vi "Optical Power Meter Utility.vi"() -> ()   [LabVIEW 2011]
uses:
  StateMachine.ctl
  <vilib>/printing/EasyPrintingControls.llb/layout_options.ctl
  <vilib>/printing/EasyPrintingControls.llb/orientation.ctl
  <vilib>/printing/EasyPrintingControls.llb/panel_scaling_for_page.ctl
  <vilib>/printing/EasyPrintingControls.llb/margins.ctl
  <vilib>/printing/EasyPrintingControls.llb/margin_values.ctl
  <vilib>/printing/EasyPrintingControls.llb/measurement_system.ctl
  <vilib>/printing/EasyPrintingControls.llb/printer_options.ctl
  <vilib>/printing/EasyPrintingControls.llb/printing_method.ctl
  <vilib>/printing/EasyPrintingControls.llb/color_or_monochrome.ctl
  <vilib>/printing/EasyPrintingControls.llb/page_header_options.ctl
  <vilib>/printing/EasyPrintingControls.llb/page_headers.ctl
  <vilib>/printing/EasyPrintingControls.llb/page_header_content_options.ctl
  <vilib>/printing/EasyPrintingControls.llb/report_type.ctl
  <vilib>/printing/EasyPrintingControls.llb/contents.ctl
  <vilib>/Utility/sysdir.llb/System Directory Type.ctl
  <vilib>/Instr/_visa.llb/VISA GPIB Control REN Mode.ctl
  <vilib>/Utility/config.llb/Write Key (I32).vi
  <vilib>/Utility/config.llb/Write Key (U32).vi
  <vilib>/Utility/config.llb/Write Key (Boolean).vi
  <vilib>/Utility/config.llb/Write Key (Double).vi
  <vilib>/printing/EasyPrinting.llb/Easy Print VI Panel or Documentation (path).vi
  <vilib>/Utility/config.llb/Read Key (I32).vi
  <vilib>/Utility/config.llb/Read Key (Double).vi
  <vilib>/Utility/config.llb/Read Key (Boolean).vi
  <vilib>/regexp/Match Regular Expression.xnode
  <vilib>/ptbypt/NI_PtbyPt.lvlib
  <vilib>/Utility/config.llb/NI_LVConfig.lvlib
  <vilib>/Utility/NIReport.llb/NI_ReportGenerationCore.lvlib
  <vilib>/Analysis/NI_AALBase.lvlib
panel:
  in  "Setup":string
  out "Res":bool
  out "Data_Dir":path
  in  "att":string
  in  "Print":bool
  in  "LTM":bool caption="Long Term Measurement"
  out "Log":bool
  in  "Arm":string
  out "VI_Path":path
  in  "Button9":bool
  in  "Button10":bool
  out "Adapter":i16
  in  "Flag1":string
  in  "Flag0":string
  out "Tau":dbl
  out "Tau?":bool
  out "Temp":bool
  out "ARM":bool
  out "Stop":bool
  in  "Frame":T1
  out "Sensor?":bool
  out "SensType":i32(ring) items=["No Sensor", "Photo", "Thermo", "Pyro"]
  out "AUTO?":bool
  out "DiaIni":dbl
  out "PM100D":refnum<visa-resource-name>
  in  "Type":u16
  in  "BW":u16(ring) items=["HIGH", "LOW"]
  in  "ACC":string(combo)
  in  "Trig":dbl=5.0
  out "AOutcm²":dbl=5.0
  in  "LambdaMax":dbl=1100.0
  in  "LambdaMin":dbl=400.0
  in  "Lambda":dbl=635.0
  in  "Range Array":string[](array[string])=["AUTO", "50nA", "500nA", "5uA", "50uA", "500uA", "5mA"]
  out "Dia":dbl
  out "SlideMulti":dbl
  in  "AVG":u32=100
  out "FileRefnum":refnum<file>
  in  "File?":bool
  in  "Samples":u32=100
  out "N":u32
  out "Data":dbl
  in  "Interval":dbl=500.0
  in  "MainUnits":enum16{"W", "V", "J", "dBm", "A"}(ring)
  in  "Digits":i32=4
  in  "Sub2":enum16{"Off", "Max", "Ratio", "Area", "Second"}(ring)=enum."Max"
  in  "Sub1":enum16{"Off", "Min", "Freq", "Temp", "Res"}(ring)=enum."Min"
  in  "Button8":bool
  in  "Button7":bool
  in  "Button6":bool
  in  "Button4":bool
  in  "Button3":bool
  in  "Button2":bool
  in  "Button5":bool
  in  "Button1":bool
  out "Header":string
  out "Slide":u32(slide) scale=0.0..1000.0
  out "Sub1":string
  out "Sub2":string
  out "Readout":string
  out "FastOut":bool
  in  "FastIn":bool
  in  "Int.":i32=10 caption="Intervals" min=1 max=9999 step=1
  in  "LogCfg":string
  in  "Stat2":string
  in  "Stat1":string
  in  "Stat0":string
  out "Histogram":T2(graph)
  in  "LogData":string
  out "YT":cluster{timestamp[], dbl[]}(graph)
  out "Unit":string="Power / W"
  out "Chart_E":dbl(graph)
  out "Chart_P":dbl(graph)
  in  "NPL":i32=1 min=1 max=100 step=1
  out "16":bool
  in  "Att":dbl format="%_6g"
  out "Wav":bool
  in  "Scale":bool
  out "H":dbl
  in  "Unt":string
  in  "LFP":path caption="Log-File Path"
  in  "Imp":bool
  out "N2":u32
  out "T":dbl
  in  "EMM":bool caption="Environmental Data"
  out "Hum":string caption="Rel. Humidity"
  out "Temp":string caption="Temperature"
  in  "Exp":bool
  in  "ClrGr":bool
  in  "XScaleFit":bool
  in  "YScaleRep":bool
  in  "YScaleFit":bool
  # "PM Series\nOptical Power and Energy Meters"
  # "Count >"
  # "Histogram"
  # "Y-Scale"
  # "Scale Fit"
  # "Map Mode"
  # "X-Scale"
  # "Scale Fit"
  # "Scale"
  # "PM100 Utility\nVersion 5.4\n12-MAY-2015\nwww.thorlabs.com"
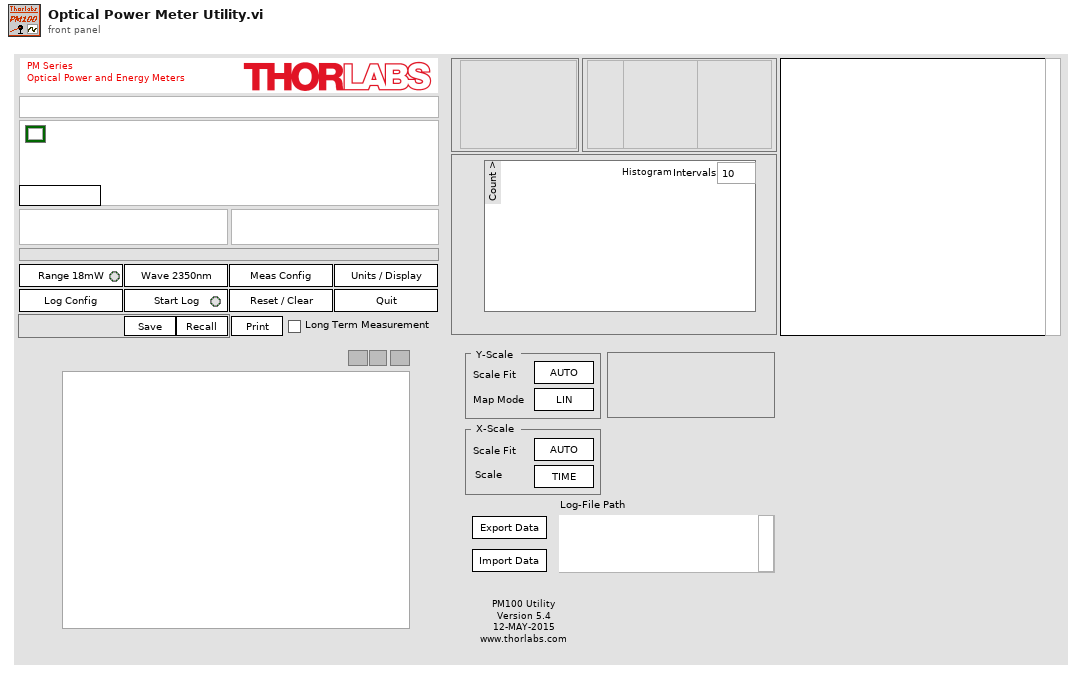
[diagram p1: front panel]
types:
  T1 = typedef "StateMachine.ctl" = enum16{"Initialize", "Load Settings", "20", "30", "40", "60", "80", "100", "120", "130", "140", "150", "160", "180", "200", "220", "240", "260", "280", "300", "320", "340", "360", "380", "400", "420", "440", "460", "480", "500", "Error", "Save Settings", "Stop"}
  T2 = cluster{"X Values":dbl[], "Histogram: h(x)":i32[]}
  T3 = enum16{"open", "replace", "create", "open or create", "replace or create", "replace or create with confirmation"}
  T4 = cluster{"X Values":i32[], "Histogram: h(x)":i32[]}
  T5 = typedef "NI_ReportGenerationCore.lvlib/layout_options.ctl" = cluster{"orientation (unchanged)":T6, "panel scaling for page (unchanged)":T7, "margins":T8, "printer options":T11, "page header options":T14}
  T6 = typedef "NI_ReportGenerationCore.lvlib/orientation.ctl" = u16
  T7 = typedef "NI_ReportGenerationCore.lvlib/panel_scaling_for_page.ctl" = u16
  T8 = typedef "NI_ReportGenerationCore.lvlib/margins.ctl" = cluster{"override VI margins (false)":bool, "margins (1.00)":T9, "measurement system (default)":T10}
  T9 = typedef "NI_ReportGenerationCore.lvlib/margin_values.ctl" = cluster{"top":dbl, "left":dbl, "right":dbl, "bottom":dbl}
  T10 = typedef "NI_ReportGenerationCore.lvlib/measurement_system.ctl" = u16
  T11 = typedef "NI_ReportGenerationCore.lvlib/printer_options.ctl" = cluster{"destination printer name (current)":string, "printing method (unchanged)":T12, "color or monochrome (unchanged)":T13}
  T12 = typedef "NI_ReportGenerationCore.lvlib/printing_method.ctl" = u16
  T13 = typedef "NI_ReportGenerationCore.lvlib/color_or_monochrome.ctl" = u16
  T14 = typedef "NI_ReportGenerationCore.lvlib/page_header_options.ctl" = cluster{"page headers (unchanged)":T15, "page header content options":T16}
  T15 = typedef "NI_ReportGenerationCore.lvlib/page_headers.ctl" = u16
  T16 = typedef "NI_ReportGenerationCore.lvlib/page_header_content_options.ctl" = cluster{"Include VI Name":bool, "Include VI Path":bool, "Include Last Modification Date":bool, "Include Date Printed":bool, "Include Page Number":bool, "Include VI Icon":bool}
  T17 = typedef "NI_LVConfig.lvlib/Config Data RefNum.ctl" = refnum<k1>
  T18 = typedef "NI_ReportGenerationCore.lvlib/report_type.ctl" = u16
  T19 = typedef "NI_ReportGenerationCore.lvlib/contents.ctl" = u16
  T20 = typedef "System Directory Type.ctl" = i32
  T21 = enum32{"invalid app kind", "Development System", "Run Time System", "Student Edition", "Embedded LabVIEW", "Evaluation", "Custom"}
  T22 = typedef "VISA GPIB Control REN Mode.ctl" = u16
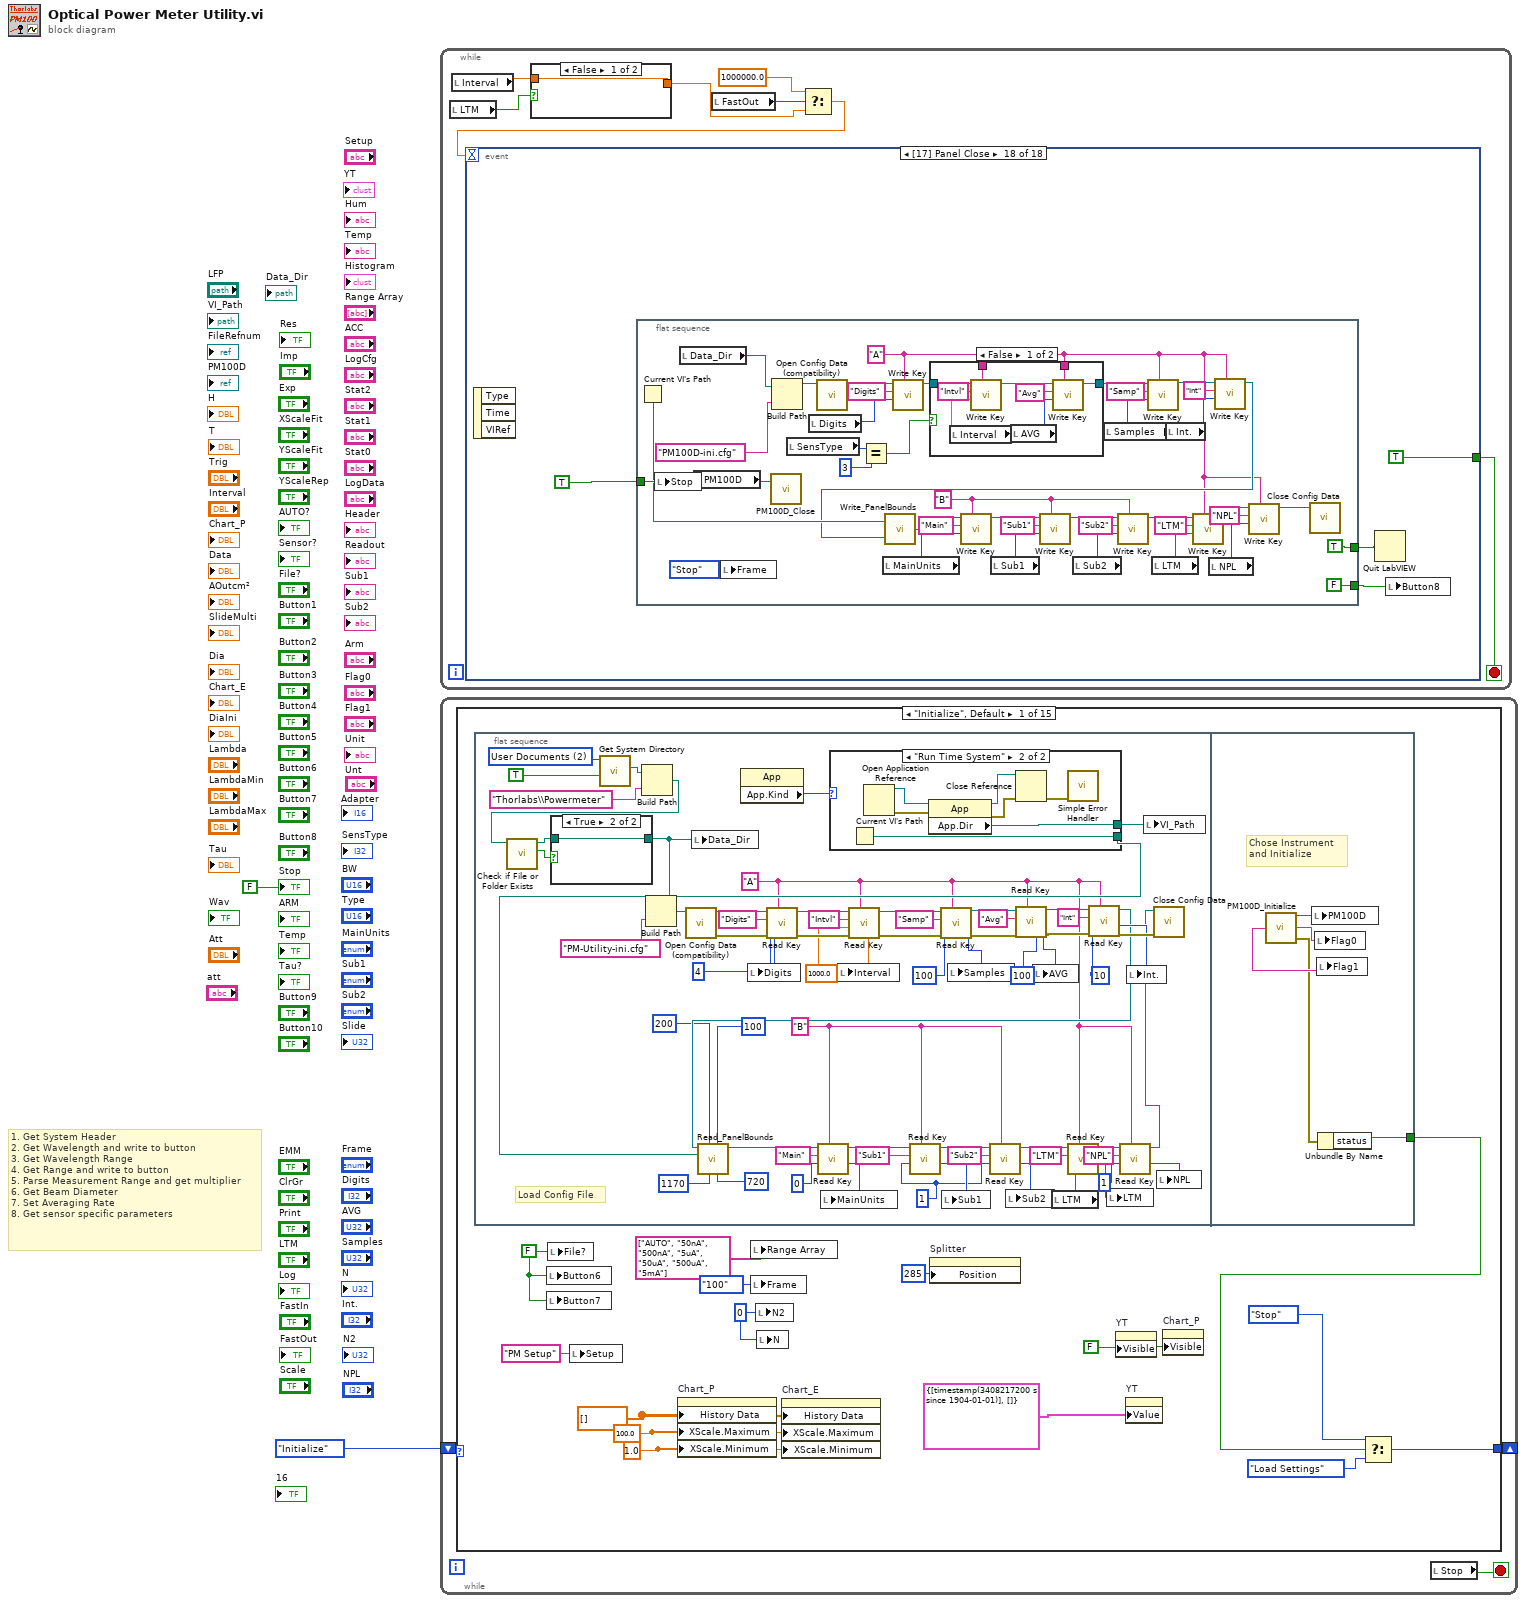
[diagram p0: block diagram]
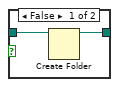
[diagram p2: hidden frame]
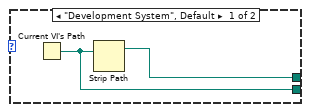
[diagram p3: hidden frame]
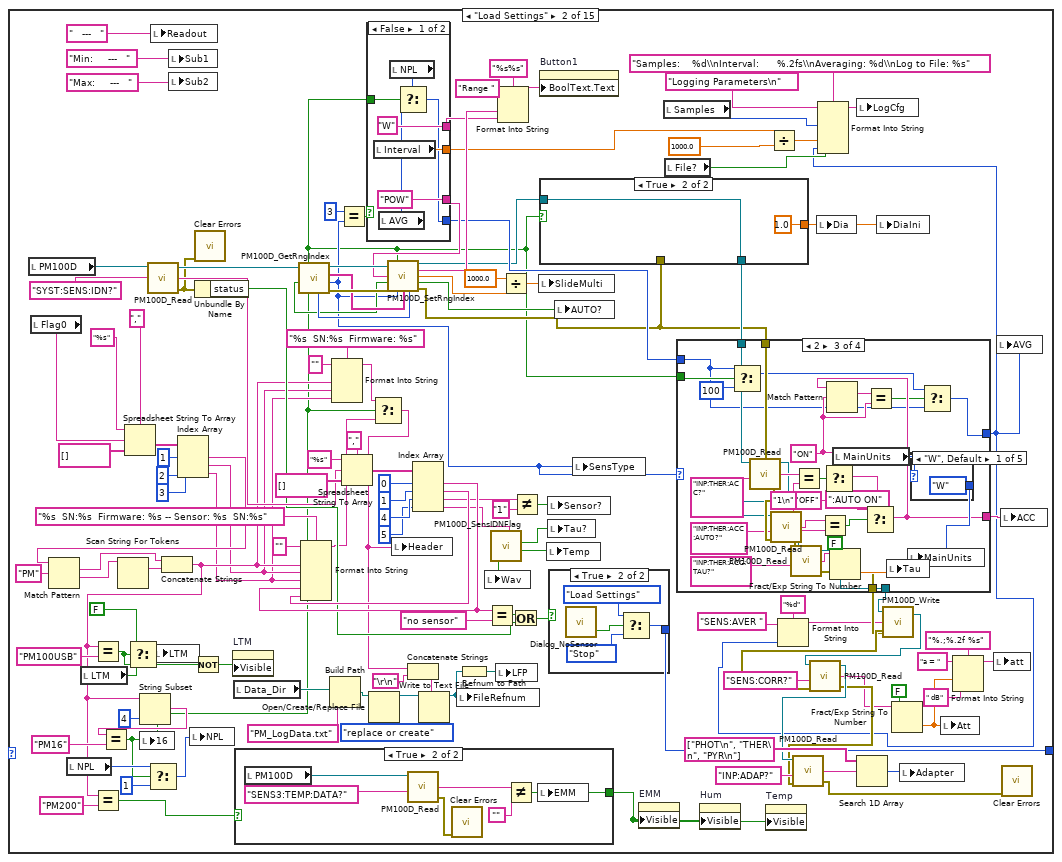
[diagram p4: hidden frame]
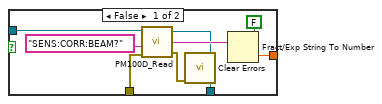
[diagram p5: hidden frame]
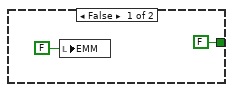
[diagram p6: hidden frame]
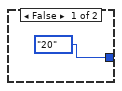
[diagram p7: hidden frame]
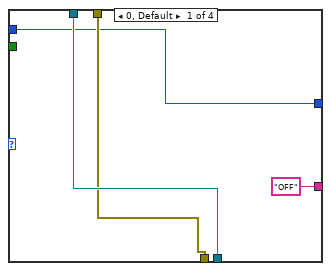
[diagram p8: hidden frame]
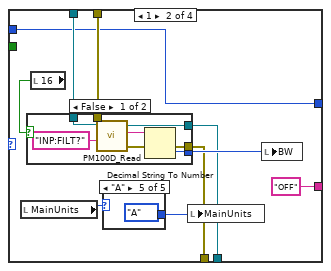
[diagram p9: hidden frame]
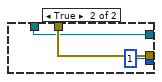
[diagram p10: hidden frame]
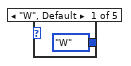
[diagram p11: hidden frame]
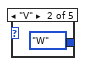
[diagram p12: hidden frame]
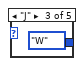
[diagram p13: hidden frame]
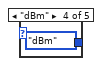
[diagram p14: hidden frame]
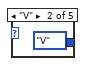
[diagram p15: hidden frame]
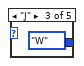
[diagram p16: hidden frame]
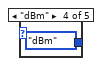
[diagram p17: hidden frame]
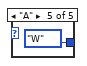
[diagram p18: hidden frame]
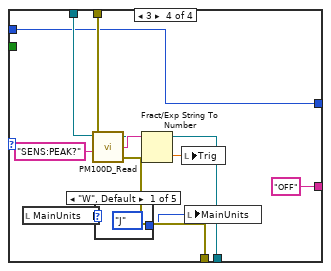
[diagram p19: hidden frame]
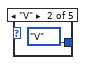
[diagram p20: hidden frame]
diagram:
  # "1. Get System Header\n2. Get Wavelength and write to button\n3. Get Wavelength Range\n4. Get Range and write to button\n5. Parse Measurement Range and get multiplier\n6. Get Beam Diameter\n7. Set Averaging Rate\n8. Get sensor specific parameters"
  n1 = while {
    stop <- w9 stop-if-true
    n2 = local read "LTM"() -> (w7:bool)
    n3 = local read "Interval"() -> (w8:dbl)
    n4 = case shown="False" w7 {
      tunnel: w8 -> [w10 w12]
      tunnel: [w10 w11] -> w4
      frame False {
      }
      frame True {
        n5 = Add(x=w12, y=100.0) -> (x+y=w11:dbl)
      }
    }
    n6 = local read "FastOut"() -> (w6:bool)
    n7 = Select(t=1000000.0, s=w6, f=w4) -> (s? t:f=w5:dbl)
    n8 = event shown="[17] Panel Close" {
      selector: _ -> [_ _ _ _ _ _ _ _ _ _ _ _ _ _ _ _ _ _]
      dyn-events: _ -> [_ _ _ _ _ _ _ _ _ _ _ _ _ _ _ _ _ _]
      timeout: w5 -> [_ _ _ _ _ _ _ _ _ _ _ _ _ _ _ _ _ _]
      tunnel: [_ _ _ _ _ _ _ _ _ TRUE ("NewVal") _ _ _ _ _ _ w537 TRUE ("NewVal")] -> w9
      event Timeout {
        # "Logging via Timeout\nmin. 0.1s interval"
        n9 = event-data() -> ()  [unwired: 1 in, 2 out]
        n10 = local read "Samples"() -> (w27:u32)
        n11 = local read "Button6"() -> (w15:bool)
        n12 = local read "SensType"() -> (w25:i32)
        n13 = local read "N"() -> (w29:u32)
        n14 = local read "Button1"() -> (w16:bool)
        n15 = local read "Button2"() -> (w17:bool)
        n16 = local read "Button3"() -> (w18:bool)
        n17 = local read "Button4"() -> (w19:bool)
        n18 = local read "Button5"() -> (w20:bool)
        n19 = Increment(x=w29) -> (x+1=w26:u32)
        n20 = Not Equal?(x=w25, y=3) -> (x != y?=w22:bool)
        n21 = Decrement(x=w26) -> (x-1=w28:u32)
        n22 = Not Equal?(x=w27, y=w28) -> (x != y?=w23:bool)
        n23 = local write "N"(w26) -> ()
        n24 = Compound Arithmetic op=AND(invert w16, invert w17, invert w18, invert w19, invert w20, w15, w22, w23) -> (w30:bool)
        n25 = case shown="True" w30 {
          tunnel: w27 -> [w36 w60]
          tunnel: w26 -> [w32 w59]
          tunnel: [0 w49] -> w21
          tunnel: w15 -> [w38 _]
          tunnel: [FALSE TRUE] -> w14
          frame False {
            n26 = Equal?(x=w38, y=TRUE) -> (x = y?=w35:bool)
            n27 = Less?(x=w32, y=w36) -> (x < y?=w34:bool)
            n28 = And(x=w35, y=w34) -> (x .and. y?=w33:bool)
            n29 = case shown="True" w33 {
              frame False {
                n30 = local write "Button6"(FALSE ("Button6")) -> ()
                n31 = local write "N"(i16 0 ("N")) -> ()
              }
              frame True {
                n32 = disable-structure shown="Enabled" {
                  frame Enabled {
                    n33 = local read "N"() -> (w43:u32)
                    n34 = Decrement(x=w43) -> (x-1=w42:u32)
                    n35 = local write "N"(w42) -> ()
                  }
                  frame Disabled {
                  }
                }
              }
            }
          }
          frame True {
            n36 = local read "PM100D"() -> (w46:refnum<visa-resource-name>)
            n37 = local read "MainUnits"() -> (w89:enum16{"W", "V", "J", "dBm", "A"})
            n38 = case shown="\"V\"" w89 {
              tunnel: ["W" "V" "J" "dBm" "A"] -> w53
              tunnel: [w133 w137 w140 FALSE w150] -> w73
              tunnel: [FALSE w137 TRUE FALSE w150] -> w72
              tunnel: [w133 TRUE w140 TRUE TRUE] -> w71
              tunnel: ["MEAS?" ("Command") "MEAS:VOLT?" ("Command") "MEAS:ENER?" ("Command") "MEAS?" ("Command") "MEAS:CURR?" ("Command")] -> w44
              frame "W", Default {
                w133 = TRUE
              }
              frame "V" {
                w137 = FALSE
              }
              frame "J" {
                w140 = FALSE
              }
              frame "dBm" {
              }
              frame "A" {
                w150 = FALSE
              }
            }
            n39 = disable-structure shown="Enabled" {
              disable-tunnel: [w99 w102] -> w57
              disable-tunnel: w46 -> [w97 w104]
              disable-tunnel: [w96 w101] -> w45
              disable-tunnel: w44 -> [w95 w103]
              frame Disabled {
                n40 = call "PM100D_Read.vi"("Command"=w95, "VISA in"=w97) -> ("error out"=w98:errorcluster, "ReadValue"=w99:string)  [unwired: 2 in, 1 out]
                n41 = Unbundle By Name(w98) -> ("status"=w96:bool)
                n42 = call <vilib>:"Clear Errors.vi"("error in (no error)"=w98) -> ()  [unwired: 6 in, 1 out]
              }
              frame Enabled {
                n43 = local read "NPL"() -> (w100:i32)
                n44 = call "PM100D_Meas_NPLC.vi"("Command"=w103, "NCPL"=w100, "VISA Refnum in"=w104) -> ("Error"=w101:bool, "Value"=w102:string)  [unwired: 5 in, 2 out]
              }
            }
            n45 = Equal?(x=i16 1, y=w59) -> (x = y?=w90:bool)
            n46 = case shown="True" w45 {
              tunnel: w46 -> [_ w105]
              frame False {
              }
              frame True {
                n47 = VISA Clear(VISA resource name=w105) -> ()  [unwired: 1 in, 2 out]
              }
            }
            n48 = Fract/Exp String To Number(use system decimal point (T)=FALSE, string=w57) -> (number=w55:dbl)  [unwired: 2 in, 1 out]
            n49 = local read "Int."() -> (w70:i32)
            n50 = Equal?(x="dBm", y=w53) -> (x = y?=w51:bool)
            n51 = local read "EMM"() -> (w66:bool)
            n52 = case shown="True" w51 {
              tunnel: w55 -> [w106 w108]
              tunnel: [w106 w107] -> w54
              frame False {
              }
              frame True {
                n53 = Multiply(x=w108, y=1000.0) -> (x*y=w110:dbl)
                n54 = Logarithm Base 10(1:w110) -> (0:w112:dbl)
                n55 = Multiply(x=10.0, y=w112) -> (x*y=w107:dbl)
              }
            }
            n56 = property on="Chart_E" class="WFChart (strict)"("Visible"=w72) -> ()  [unwired: 2 in, 2 out]
            n57 = property on="Chart_P" class="WFChart (strict)"("Visible"=w71) -> ()  [unwired: 2 in, 2 out]
            n58 = call <vilib>:"Histogram PtByPt.vi"("initialize"=w90, "sample length"=w60, "intervals"=w70, "x"=w54) -> ("Histogram Graph"=w93:T2)  [unwired: 4 in, 3 out]
            n59 = call <vilib>:"Array Max & Min PtByPt.vi"("input data point"=w54, "sample length"=w60, "initialize"=w90) -> ("max value"=w81:dbl, "min value"=w82:dbl)  [unwired: 3 out]
            n60 = call <vilib>:"Standard Deviation PtByPt.vi"("x"=w54, "sample length"=w60, "initialize"=w90) -> ("standard deviation"=w88:dbl, "mean"=w80:dbl)  [unwired: 1 out]
            n61 = call <vilib>:"RMS PtByPt.vi"("initialize"=w90, "sample length"=w60, "x"=w54) -> ("rms value"=w79:dbl)  [unwired: 1 in, 1 out]
            n62 = call "GetDateTime.vi"() -> ("date&time"=w47:string)
            n63 = Format Into String(format string="%d\\n%.3p%s\\n%.3p%s\\n%.3p%s\\n%.3p%s\\n%.3p%s", w59, w82, w53, w81, w53, w80, w53, w79, w53, w88, w53) -> (resulting string=w92:string)  [unwired: 2 in, 1 out]
            n64 = case shown="True" w66 {
              tunnel: [w124 w129] -> w50
              tunnel: w54 -> [w123 w128]
              tunnel: w53 -> [w122 w127]
              tunnel: w47 -> [w121 w126]
              frame True {
                n65 = local read "H"() -> (w119:dbl)
                n66 = local read "T"() -> (w120:dbl)
                n67 = Format Into String(format string="\\t%.4e\\t%s\\t%.1f\\t°C\\t%.1f\\tRH\\n", initial string=w121, w123, w122, w120, w119) -> (resulting string=w124:string)  [unwired: 1 in, 1 out]
              }
              frame False {
                n68 = Format Into String(format string="\\t%.4e\\t%s\\n", initial string=w126, w128, w127) -> (resulting string=w129:string)  [unwired: 1 in, 1 out]
              }
            }
            n69 = Concatenate Strings("Power / " ("string"), w53) -> (w68:string)
            n70 = local write "Unit"(w68) -> ()
            n71 = local write "Chart_E"(w54) -> ()
            n72 = call "lin-log.vi"("W In 1"=w79, "W In 2"=w80, "W In 3"=w81, "W In 4"=w82) -> ("dBm Out 1"=w83:dbl, "dBm Out 2"=w84:dbl, "dBm Out 3"=w85:dbl, "dBm Out 4"=w86:dbl)
            n73 = local write "Histogram"(w93) -> ()
            n74 = Format Into String(format string="%.3fdBm\\n%.3fdBm\\n%.3fdBm\\n%.3fdBm", initial string="\n", w86, w85, w84, w83) -> (resulting string=w77:string)  [unwired: 1 in, 1 out]
            n75 = local write "Chart_P"(w54) -> ()
            n76 = local read "FileRefnum"() -> (w63:refnum<file>)
            n77 = local write "Stat1"(w92) -> ()
            n78 = local write "Stat0"("Count:\nMin:\nMax:\nMean:\nRMS:\nSigma:" ("Stat0")) -> ()
            n79 = local read "LogData"() -> (w64:string)
            n80 = Select(t=w77, s=w73, f="") -> (s? t:f=w76:string)
            n81 = property on="YT" class="XYGraph (strict)"("Visible"=FALSE) -> ()  [unwired: 2 in, 2 out]
            n82 = Equal?(x=w60, y=w59) -> (x = y?=w61:bool)
            n83 = Concatenate Strings(w50, w64) -> (w65:string)
            n84 = local write "Stat2"(w76) -> ()
            n85 = Write to Text File(file (use dialog)=w63, text=w50) -> (refnum out=w58:refnum<file>)  [unwired: 2 in, 2 out]
            n86 = local write "LogData"(w65) -> ()
            n87 = case shown="True" w61 {
              tunnel: [StateMachine."120" ("Frame") StateMachine."300" ("Frame")] -> w62
              tunnel: w58 -> [_ w117]
              tunnel: [2 0] -> w49
              frame False {
              }
              frame True {
                n88 = Refnum to Path(1:w117) -> (0:w116:path)
                n89 = local write "LFP"(w116) -> ()
              }
            }
            n90 = local write "Frame"(w62) -> ()
          }
        }
        n91 = local write "Log"(w14) -> ()
        n92 = property on="Button1" class="Bool (strict)"("Disabled"=w21) -> ()  [unwired: 2 in, 2 out]
        n93 = property on="Button2" class="Bool (strict)"("Disabled"=w21) -> ()  [unwired: 2 in, 2 out]
        n94 = property on="Button3" class="Bool (strict)"("Disabled"=w21) -> ()  [unwired: 2 in, 2 out]
        n95 = property on="Button4" class="Bool (strict)"("Disabled"=w21) -> ()  [unwired: 2 in, 2 out]
        n96 = property on="Button5" class="Bool (strict)"("Disabled"=w21) -> ()  [unwired: 2 in, 2 out]
      }
      event "att": Mouse Down {
        n97 = event-data() -> ()  [unwired: 1 in, 8 out]
        n98 = local write "N2"(u32 0 ("N")) -> ()
        n99 = local write "Frame"(StateMachine."240" ("Frame")) -> ()
      }
      event "Button1": Value Change {
        # "Set Range - goto Frame 200"
        n100 = event-data() -> ("NewVal"=w157:bool)  [unwired: 1 in, 5 out]
        n101 = Equal?(x=w157, y=TRUE) -> (x = y?=w155:bool)
        n102 = case shown="True" w155 {
          frame False {
          }
          frame True {
            n103 = local write "Frame"(StateMachine."200" ("Frame")) -> ()
          }
        }
        n104 = local write "N2"(u32 0 ("N2")) -> ()
      }
      event "Button2": Value Change {
        # "Set Wavelength - goto Frame 220"
        n105 = event-data() -> ("NewVal"=w162:bool)  [unwired: 1 in, 5 out]
        n106 = Equal?(x=w162, y=TRUE) -> (x = y?=w160:bool)
        n107 = case shown="True" w160 {
          frame False {
          }
          frame True {
            n108 = local write "Frame"(StateMachine."220" ("Frame")) -> ()
          }
        }
        n109 = local write "N2"(u32 0 ("N2")) -> ()
      }
      event "Button3": Value Change {
        # "Set Measuremnt Configuration - goto Frame 240"
        n110 = event-data() -> ("NewVal"=w167:bool)  [unwired: 1 in, 5 out]
        n111 = Equal?(x=w167, y=TRUE) -> (x = y?=w165:bool)
        n112 = case shown="True" w165 {
          frame False {
          }
          frame True {
            n113 = local write "Frame"(StateMachine."240" ("Frame")) -> ()
          }
        }
        n114 = local write "N2"(u32 0 ("N2")) -> ()
      }
      event "Button4": Value Change {
        # "Set Units - goto Frame 260"
        n115 = event-data() -> ("NewVal"=w172:bool)  [unwired: 1 in, 5 out]
        n116 = Equal?(x=w172, y=TRUE) -> (x = y?=w170:bool)
        n117 = case shown="True" w170 {
          frame False {
          }
          frame True {
            n118 = local write "Frame"(StateMachine."260" ("Frame")) -> ()
          }
        }
        n119 = local write "N2"(u32 0 ("N2")) -> ()
      }
      event "Button5": Value Change {
        # "Set Logging Parameters Goto 280"
        n120 = event-data() -> ("NewVal"=w177:bool)  [unwired: 1 in, 5 out]
        n121 = Equal?(x=w177, y=TRUE) -> (x = y?=w175:bool)
        n122 = case shown="True" w175 {
          frame False {
          }
          frame True {
            n123 = local write "Frame"(StateMachine."280" ("Frame")) -> ()
          }
        }
        n124 = local write "N2"(u32 0 ("N2")) -> ()
      }
      event "Button6": Value Change {
        # "Start/Stop"
        n125 = event-data() -> ()  [unwired: 1 in, 6 out]
        n126 = local read "Button6"() -> (w181:bool)
        n127 = Equal?(x=w181, y=FALSE) -> (x = y?=w179:bool)
        n128 = case shown="True" w179 {
          frame False {
          }
          frame True {
            n129 = local write "Frame"(StateMachine."300" ("Frame")) -> ()
          }
        }
      }
      event "Button7": Value Change {
        w198 = 1.0 ("X Scale.Range:Minimum")
        w199 = 100.0 ("X Scale.Range:Maximum")
        w197 = i16 0 ("N")
        w203 = dbl[] [] ("History Data")
        w188 = ""
        # "Reset/Clear"
        n130 = event-data() -> ()  [unwired: 1 in, 6 out]
        n131 = local read "Data_Dir"() -> (w185:path)
        n132 = local write "N"(w197) -> ()
        n133 = local write "LogData"(w188) -> ()
        n134 = Build Path(base path=w185, name or relative path="PM_LogData.txt") -> (appended path=w195:path)
        n135 = property on="Chart_P" class="WFChart (strict)"("History Data"=w203, "XScale.Maximum"=w199, "XScale.Minimum"=w198) -> ()  [unwired: 2 in, 2 out]
        n136 = local write "Histogram"(T4 {"X Values"=[], "Histogram: h(x)"=[]} ("Histogram Graph")) -> ()
        n137 = local write "N2"(w197) -> ()
        n138 = local write "Stat2"(w188) -> ()
        n139 = local read "Header"() -> (w191:string)
        n140 = Open/Create/Replace File(file path (use dialog)=w195, operation (0:open)=T3."replace or create") -> (refnum out=w193:refnum<file>)  [unwired: 4 in, 2 out]
        n141 = local write "Stat1"(w188) -> ()
        n142 = property on="Chart_E" class="WFChart (strict)"("History Data"=w203, "XScale.Maximum"=w199, "XScale.Minimum"=w198) -> ()  [unwired: 2 in, 2 out]
        n143 = Concatenate Strings(w191, "\r\n") -> (w189:string)
        n144 = Write to Text File(file (use dialog)=w193, text=w189) -> (refnum out=w187:refnum<file>, error out=w190:errorcluster)  [unwired: 2 in, 1 out]
        n145 = local write "Frame"(StateMachine."100" ("Frame")) -> ()
        n146 = local read "File?"() -> (w186:bool)
        n147 = local write "Readout"("   ---   " ("Readout")) -> ()
        n148 = local write "Sub1"("Min:     ---   " ("Sub1")) -> ()
        n149 = local write "Sub2"("Max:     ---   " ("Sub2")) -> ()
        n150 = call <vilib>:"Clear Errors.vi"("error in (no error)"=w190) -> ()  [unwired: 6 in, 1 out]
        n151 = case shown="False" w186 {
          tunnel: w187 -> [w207 _]
          frame False {
            n152 = local write "FileRefnum"(w207) -> ()
            n153 = Refnum to Path(1:w207) -> (0:w206:path)
            n154 = local write "LFP"(w206) -> ()
          }
          frame True {
          }
        }
        n155 = local write "Res"(TRUE ("Res")) -> ()
        n156 = Wait (ms)(milliseconds to wait=u32 200) -> ()  [unwired: 1 out]
      }
      event "Button8": Value Change {
        # "Quit"
        n157 = event-data() -> ("NewVal"=w211:bool)  [unwired: 1 in, 5 out]
        n158 = Equal?(x=w211, y=TRUE) -> (x = y?=w210:bool)
        n159 = case shown="True" w210 {
          selector: w210 -> [_ w215]
          frame False {
          }
          frame True {
            n160 = flat-sequence {
              tunnel: w215 -> [w254]
              tunnel: [FALSE ("Button8")] -> w214
              tunnel: [TRUE] -> w213
              frame #0 {
                w233 = "B" ("section")
                w219 = "A" ("section")
                n161 = local write "Stop"(w254) -> ()
                n162 = local read "Data_Dir"() -> (w221:path)
                n163 = local read "PM100D"() -> (w256:refnum<visa-resource-name>)
                n164 = local write "Frame"(StateMachine."Stop" ("Frame")) -> ()
                n165 = call "PM100D_Close.vi"("VISA resource name"=w256) -> ()  [unwired: 3 in]
                n166 = Build Path(base path=w221, name or relative path="PM-Utility-ini.cfg") -> (appended path=w253:path)
                n167 = local read "SensType"() -> (w241:i32)
                n168 = local read "Digits"() -> (w250:i32)
                n169 = call <vilib>:"Open Config Data (compatibility).vi"("configuration file path"=w253) -> ("refnum"=w245:T17)  [unwired: 8 in, 2 out]
                n170 = Current VI's Path() -> (path=w222:path)
                n171 = Equal?(x=w241, y=3) -> (x = y?=w239:bool)
                n172 = local read "MainUnits"() -> (w229:enum16{"W", "V", "J", "dBm", "A"})
                n173 = call-poly <vilib>:"Write Key.vi"("section"=w219, "value"=w250, "key"="Digits", "refnum"=w245) -> ("refnum out"=w247:T17)  [unwired: 5 in, 2 out]
                n174 = case shown="False" w239 {
                  tunnel: [w259 w266] -> w249
                  tunnel: w247 -> [w264 w266]
                  tunnel: w219 -> [w262 _]
                  tunnel: w219 -> [w257 _]
                  frame False {
                    n175 = local read "Interval"() -> (w265:dbl)
                    n176 = call-poly <vilib>:"Write Key.vi"("section"=w262, "value"=w265, "key"="Intvl", "refnum"=w264) -> ("refnum out"=w258:T17)  [unwired: 5 in, 2 out]
                    n177 = local read "AVG"() -> (w261:u32)
                    n178 = call-poly <vilib>:"Write Key.vi"("section"=w257, "value"=w261, "key"="Avg", "refnum"=w258) -> ("refnum out"=w259:T17)  [unwired: 5 in, 2 out]
                  }
                  frame True {
                  }
                }
                n179 = local read "Sub1"() -> (w227:enum16{"Off", "Min", "Freq", "Temp", "Res"})
                n180 = local read "Sub2"() -> (w228:enum16{"Off", "Max", "Ratio", "Area", "Second"})
                n181 = local read "Samples"() -> (w251:u32)
                n182 = call-poly <vilib>:"Write Key.vi"("section"=w219, "value"=w251, "key"="Samp", "refnum"=w249) -> ("refnum out"=w237:T17)  [unwired: 5 in, 2 out]
                n183 = local read "LTM"() -> (w224:bool)
                n184 = local read "NPL"() -> (w216:i32)
                n185 = local read "Int."() -> (w243:i32)
                n186 = call-poly <vilib>:"Write Key.vi"("section"=w219, "value"=w243, "key"="Int", "refnum"=w237) -> ("refnum out"=w238:T17)  [unwired: 5 in, 2 out]
                n187 = call "Write_PanelBounds.vi"("refnum in"=w238, "path"=w222) -> ("refnum out"=w236:T17)
                n188 = call-poly <vilib>:"Write Key.vi"("section"=w233, "value"=w229, "key"="Main", "refnum"=w236) -> ("refnum out"=w235:T17)  [unwired: 5 in, 2 out]
                n189 = call-poly <vilib>:"Write Key.vi"("section"=w233, "value"=w227, "key"="Sub1", "refnum"=w235) -> ("refnum out"=w234:T17)  [unwired: 5 in, 2 out]
                n190 = call-poly <vilib>:"Write Key.vi"("section"=w233, "value"=w228, "key"="Sub2", "refnum"=w234) -> ("refnum out"=w225:T17)  [unwired: 5 in, 2 out]
                n191 = call-poly <vilib>:"Write Key.vi"("section"=w219, "value"=w224, "key"="LTM", "refnum"=w225) -> ("refnum out"=w220:T17)  [unwired: 5 in, 2 out]
                n192 = call-poly <vilib>:"Write Key.vi"("section"=w219, "value"=w216, "key"="NPL", "refnum"=w220) -> ("refnum out"=w218:T17)  [unwired: 5 in, 2 out]
                n193 = call <vilib>:"Close Config Data.vi"("refnum"=w218) -> ()  [unwired: 9 in, 2 out]
              }
            }
            n194 = local write "Button8"(w214) -> ()
            n195 = Quit LabVIEW(quit? (T)=w213) -> ()
          }
        }
        n196 = local write "N2"(u32 0 ("N2")) -> ()
      }
      event "Button9": Value Change {
        (unwired) "PM100 Setup_1" ("default name")
        # "Recall Instrument Setup"
        n197 = event-data() -> ()  [unwired: 1 in, 6 out]
        n198 = local read "Setup"() -> (w267:string)
        n199 = local read "Data_Dir"() -> (w272:path)
        n200 = call "File Dialog2"("start path"=w272, "default name"=w267, "pattern (all files)"="*.txt", "pattern label"="Textfile") -> ("selected path"=w271:path, "cancelled"=w276:bool, "error out"=w278:errorcluster)  [unwired: 8 in, 1 out]
        n201 = Strip Path(path=w271) -> (name=w270:string)  [unwired: 1 out]
        n202 = local write "N2"(u32 0 ("N2")) -> ()
        n203 = Open/Create/Replace File(file path (use dialog)=w271, error in=w278, operation (0:open)=T3."open") -> (refnum out=w275:refnum<file>, error out=w279:errorcluster)  [unwired: 3 in, 1 out]
        n204 = Match Pattern(string=w270, regular expression=".txt") -> (before substring=w268:string)  [unwired: 1 in, 3 out]
        n205 = local write "Setup"(w268) -> ()
        n206 = call <vilib>:"Clear Errors.vi"("error in (no error)"=w279) -> ()  [unwired: 6 in, 1 out]
        n207 = case shown="False" w276 {
          tunnel: w275 -> [w382 _]
          frame False {
            w345 = 0 ("default value 8")
            n208 = local read "PM100D"() -> (w281:refnum<visa-resource-name>)
            n209 = local read "Lambda"() -> (w380:dbl)
            n210 = local read "Tau"() -> (w379:dbl)
            n211 = local read "Dia"() -> (w378:dbl)
            n212 = local read "Adapter"() -> (w347:i16)
            n213 = local read "BW"() -> (w363:u16)
            n214 = local read "SensType"() -> (w344:i32)
            n215 = local read "Sensor?"() -> (w320:bool)
            n216 = local read "Trig"() -> (w326:dbl)
            n217 = local read "Digits"() -> (w325:i32)
            n218 = local read "AVG"() -> (w324:u32)
            n219 = local read "Att"() -> (w323:dbl)
            n220 = local read "Interval"() -> (w322:dbl)
            n221 = local read "Samples"() -> (w292:u32)
            n222 = local read "MainUnits"() -> (w336:enum16{"W", "V", "J", "dBm", "A"})
            n223 = Scan From String("%d %f %f %f %d %d %d %d %f %d %d %f %f %d" ("format string"), w382, default 1=1 ("default value 1"), default 2=w380, default 3=w379, default 4=w378, default 5=w347, default 6=w363, default 7=w345, default 8=w345, default 9=w326, default 10=w325, default 11=w324, default 12=w323, default 13=w322, default 14=w292) -> (w351:refnum<file>, w354:errorcluster, output 1=w353:i32, output 2=w366:dbl, output 3=w372:dbl, output 4=w377:dbl, output 5=w348:i16, output 6=w360:u16, output 7=w339:i32, output 8=w341:i32, output 9=w315:dbl, output 10=w321:i32, output 11=w284:u32, output 12=w302:dbl, output 13=w285:dbl, output 14=w286:u32)  [unwired: 1 in]
            n224 = Number To Boolean Array(number=w341) -> (Boolean array=w343:bool[])
            n225 = Index Array(array=w343, index=0) -> (element=w340:bool)
            n226 = Format Into String(format string="%.;%.2f %s", initial string="a = ", w302, " dB") -> (resulting string=w301:string)  [unwired: 1 in, 1 out]
            n227 = case shown="\"V\"" w336 {
              tunnel: ["POW" "VOLT" "ENER" "POW" "CURR"] -> w335
              tunnel: ["W" "V" "J" "W" "A"] -> w328
              tunnel: w281 -> [w383 w386 w389 w392 w395]
              tunnel: [w383 w386 w389 w392 w395] -> w282
              frame "W", Default {
              }
              frame "V" {
              }
              frame "J" {
              }
              frame "dBm" {
              }
              frame "A" {
              }
            }
            n228 = local write "att"(w301) -> ()
            n229 = local write "Interval"(w285) -> ()
            n230 = local write "Trig"(w315) -> ()
            n231 = local write "Digits"(w321) -> ()
            n232 = local write "AVG"(w284) -> ()
            n233 = local write "Att"(w302) -> ()
            n234 = Not Equal?(x=w348, y=w347) -> (x != y?=w346:bool)
            n235 = local write "Lambda"(w366) -> ()
            n236 = local write "Adapter"(w348) -> ()
            n237 = call <vilib>:"Clear Errors.vi"("error in (no error)"=w354) -> ()  [unwired: 6 in, 1 out]
            n238 = local write "Tau"(w372) -> ()
            n239 = local write "Dia"(w377) -> ()
            n240 = call "PM100D_Ranging.vi"("VISA in"=w282, "Index"=w339, "AUTO"=w340, "Unit"=w335) -> ("AUTO?"=w334:bool, "VISA out"=w338:refnum<visa-resource-name>, "RANG_Val"=w333:dbl, "RANG_lbl"=w327:string, "error out"=w337:errorcluster)  [unwired: 4 in, 3 out]
            n241 = case shown="0" w353 {
              tunnel: [" ON" ("ACCOut") " OFF" ("ACCOut") ":AUTO ON" ("ACCOut")] -> w367
              tunnel: ["ON" ("ACCOut") "OFF" ("ACCOut") "AUTO" ("ACCOut")] -> w352
              frame 0 {
              }
              frame 2 {
              }
              frame 1, Default {
              }
            }
            n242 = Close File(refnum=w351) -> ()  [unwired: 1 in, 2 out]
            n243 = local write "Samples"(w286) -> ()
            n244 = local write "BW"(w360) -> ()
            n245 = local read "File?"() -> (w283:bool)
            n246 = local write "ACC"(w352) -> ()
            n247 = Format Into String(format string="%.;%f", initial string="INP:THER:ACC:TAU ", w372) -> (resulting string=w373:string)  [unwired: 1 in, 1 out]
            n248 = Format Into String(format string="%.;%f", initial string="SENS:CORR:BEAM ", w377) -> (resulting string=w376:string)  [unwired: 1 in, 1 out]
            n249 = local write "AUTO?"(w334) -> ()
            n250 = Divide(x=w285, y=1000.0) -> (x/y=w289:dbl)
            n251 = Format Into String(format string="INP:THER:ACC%s", w367) -> (resulting string=w368:string)  [unwired: 2 in, 1 out]
            n252 = Format Into String(format string="Samples:    %d\\nInterval:      %.2fs\\nAveraging: %d\\nLog to File: %s", initial string="Logging Parameters\n", w286, w289, w284, w283) -> (resulting string=w287:string)  [unwired: 1 in, 1 out]
            n253 = call "PM100D_Write.vi"("error in (no error)"=w337, "Command"=w368, "VISA in"=w338) -> ("error out"=w297:errorcluster, "VISA out"=w359:refnum<visa-resource-name>)
            n254 = call "PM100D_Write.vi"("Command"=w373, "VISA in"=w359) -> ("error out"=w296:errorcluster, "VISA out"=w358:refnum<visa-resource-name>)  [unwired: 1 in]
            n255 = call "PM100D_Write.vi"("Command"=w376, "VISA in"=w358) -> ("error out"=w295:errorcluster, "VISA out"=w357:refnum<visa-resource-name>)  [unwired: 1 in]
            n256 = case shown="False" w346 {
              tunnel: w357 -> [w399 w403]
              tunnel: [w399 w402] -> w356
              tunnel: [errorcluster {"status"=FALSE, "code"=0, "source"=""} ("error out") w401] -> w294
              tunnel: w348 -> [_ w400]
              frame False {
              }
              frame True {
                n257 = case shown="2" w400 {
                  tunnel: ["INP:ADAP PHOT" "INP:ADAP THER" "INP:ADAP PYR"] -> w404
                  frame 0, Default {
                  }
                  frame 1 {
                  }
                  frame 2 {
                  }
                }
                n258 = call "PM100D_Write.vi"("Command"=w404, "VISA in"=w403) -> ("error out"=w401:errorcluster, "VISA out"=w402:refnum<visa-resource-name>)  [unwired: 1 in]
              }
            }
            n259 = call <vilib>:"Clear Errors.vi"("error in (no error)"=w295) -> ()  [unwired: 6 in, 1 out]
            n260 = call <vilib>:"Clear Errors.vi"("error in (no error)"=w296) -> ()  [unwired: 6 in, 1 out]
            n261 = case shown="True" w320 {
              tunnel: w366 -> [w410 _]
              tunnel: [w409 w416] -> w364
              tunnel: [w408 w415] -> w365
              tunnel: w344 -> [_ w418]
              tunnel: w366 -> [_ w417]
              frame True {
                n262 = Format Into String(format string="%dnm", initial string="Wave ", w410) -> (resulting string=w409:string)  [unwired: 1 in, 1 out]
                n263 = Format Into String(format string="%d", initial string="SENS:CORR:WAV " ("Command"), w410) -> (resulting string=w408:string)  [unwired: 1 in, 1 out]
              }
              frame False {
                n264 = case shown="1" w418 {
                  tunnel: [w423 "" ("initial string") "" ("initial string") "" ("initial string")] -> w422
                  tunnel: [w423 "%.;%_3pA/W" ("format string") "%.;%_3pV/W" ("format string") "%.;%_3pV/J" ("format string")] -> w421
                  tunnel: [w423 "SENS:CORR:POW " ("Command") "SENS:CORR:POW:THER " ("Command") "SENS:CORR:ENER " ("Command")] -> w420
                  tunnel: [w423 "%.;%.6e" ("format string") "%.;%.6e" ("format string") "%.;%.6e" ("format string")] -> w419
                  frame 0, Default {
                    w423 = "" ("format string")
                  }
                  frame 1 {
                  }
                  frame 2 {
                  }
                  frame 3 {
                  }
                }
                n265 = Format Into String(format string=w421, initial string=w422, w417) -> (resulting string=w416:string)  [unwired: 1 in, 1 out]
                n266 = Format Into String(format string=w419, initial string=w420, w417) -> (resulting string=w415:string)  [unwired: 1 in, 1 out]
              }
            }
            n267 = local write "LogCfg"(w287) -> ()
            n268 = call <vilib>:"Clear Errors.vi"("error in (no error)"=w294) -> ()  [unwired: 6 in, 1 out]
            n269 = Divide(x=1000.0, y=w333) -> (x/y=w331:dbl)
            n270 = call <vilib>:"Clear Errors.vi"("error in (no error)"=w297) -> ()  [unwired: 6 in, 1 out]
            n271 = local write "SlideMulti"(w331) -> ()
            n272 = Format Into String(format string="INP:FILT %d", w360) -> (resulting string=w362:string)  [unwired: 2 in, 1 out]
            n273 = Concatenate Strings("Range " ("string"), w327, w328) -> (w330:string)
            n274 = property on="Button1" class="Bool (strict)"("BoolText.Text"=w330) -> ()  [unwired: 2 in, 2 out]
            n275 = property on="Button2" class="Bool (strict)"("BoolText.Text"=w364) -> ()  [unwired: 2 in, 2 out]
            n276 = Number To Fractional String(use system decimal point (T)=FALSE, number=w302) -> (F-format string=w312:string)  [unwired: 2 in]
            n277 = call "PM100D_Write.vi"("Command"=w365, "VISA in"=w356) -> ("error out"=w293:errorcluster, "VISA out"=w355:refnum<visa-resource-name>)  [unwired: 1 in]
            n278 = call "PM100D_Write.vi"("Command"=w362, "VISA in"=w355) -> ("error out"=w298:errorcluster, "VISA out"=w309:refnum<visa-resource-name>)  [unwired: 1 in]
            n279 = Format Into String(format string="%d", initial string="SENS:AVER " ("Command"), w284) -> (resulting string=w317:string)  [unwired: 1 in, 1 out]
            n280 = local write "Button9"(FALSE ("Load")) -> ()
            n281 = Format Into String(format string="SENS:PEAK %.;%f", w315) -> (resulting string=w313:string)  [unwired: 2 in, 1 out]
            n282 = Concatenate Strings("SENS:CORR " ("string"), w312) -> (w307:string)
            n283 = call <vilib>:"Clear Errors.vi"("error in (no error)"=w293) -> ()  [unwired: 6 in, 1 out]
            n284 = call <vilib>:"Clear Errors.vi"("error in (no error)"=w298) -> ()  [unwired: 6 in, 1 out]
            n285 = call "PM100D_Write.vi"("Command"=w307, "VISA in"=w309) -> ("error out"=w299:errorcluster, "VISA out"=w308:refnum<visa-resource-name>)  [unwired: 1 in]
            n286 = call "PM100D_Write.vi"("Command"=w317, "VISA in"=w308) -> ("error out"=w300:errorcluster, "VISA out"=w314:refnum<visa-resource-name>)  [unwired: 1 in]
            n287 = call "PM100D_Write.vi"("Command"=w313, "VISA in"=w314) -> ("error out"=w306:errorcluster)  [unwired: 1 in, 1 out]
            n288 = call <vilib>:"Clear Errors.vi"("error in (no error)"=w299) -> ()  [unwired: 6 in, 1 out]
            n289 = call <vilib>:"Clear Errors.vi"("error in (no error)"=w300) -> ()  [unwired: 6 in, 1 out]
            n290 = call <vilib>:"Clear Errors.vi"("error in (no error)"=w306) -> ()  [unwired: 6 in, 1 out]
          }
          frame True {
          }
        }
      }
      event "Button10": Value Change {
        (unwired) "PM100 Setup_1" ("default name")
        # "01 %d Accelerator 0/1/2 --> Instr\n02 %f Lambda                 --> Instr\n03 %f Tau                         --> Instr\n04 %f Diameter                --> Instr   \n05 %d Adapter       0/1/2  --> Instr\n06 %d Bandwidth   0/1    --> Instr\n07 %d Range Index          --> Instr\n08 %d Autorange   0/1    --> Instr\n09 %f Trigger Level         --> Instr\n10 %d Digits                   xx App\n11 %d Averaging              --> Instr\n12 %f Attenuation           --> Instr\n13 %f Interval                xx App\n14 %d Samples              xx App"
        # "Save Instrument Setup"
        n291 = event-data() -> ()  [unwired: 1 in, 6 out]
        n292 = local read "Setup"() -> (w442:string)
        n293 = local read "Data_Dir"() -> (w447:path)
        n294 = call "File Dialog"("start path"=w447, "default name"=w442, "pattern (all files)"="*.txt", "pattern label"="Textfile") -> ("selected path"=w446:path, "cancelled"=w452:bool, "error out"=w453:errorcluster)  [unwired: 8 in, 1 out]
        n295 = Strip Path(path=w446) -> (name=w443:string)  [unwired: 1 out]
        n296 = Open/Create/Replace File(file path (use dialog)=w446, error in=w453, operation (0:open)=T3."replace or create") -> (refnum out=w457:refnum<file>, error out=w455:errorcluster)  [unwired: 3 in, 1 out]
        n297 = local read "PM100D"() -> (w449:refnum<visa-resource-name>)
        n298 = call <vilib>:"Clear Errors.vi"("error in (no error)"=w455) -> ()  [unwired: 6 in, 1 out]
        n299 = Match Pattern(string=w443, regular expression=".txt") -> (before substring=w444:string)  [unwired: 1 in, 3 out]
        n300 = local write "Setup"(w444) -> ()
        n301 = case shown="False" w452 {
          tunnel: w457 -> [w479 _]
          tunnel: w449 -> [w468 _]
          frame False {
            n302 = call "PM100D_GetRngIndex.vi"("VISA in"=w468) -> ("error out"=w464:errorcluster, "IndexOut"=w467:i32, "AutoOut"=w466:bool)  [unwired: 5 in, 3 out]
            n303 = call <vilib>:"Clear Errors.vi"("error in (no error)"=w464) -> ()  [unwired: 6 in, 1 out]
            n304 = local read "ACC"() -> (w470:string)
            n305 = local read "Samples"() -> (w458:u32)
            n306 = local read "Lambda"() -> (w478:dbl)
            n307 = local read "Adapter"() -> (w475:i16)
            n308 = local read "Trig"() -> (w463:dbl)
            n309 = local read "Tau"() -> (w477:dbl)
            n310 = local read "Dia"() -> (w476:dbl)
            n311 = local read "BW"() -> (w472:u16)
            n312 = case shown="\"OFF\"" w470 {
              tunnel: [0 0 1 1 2 2] -> w469
              frame "ON", Default {
              }
              frame " ON" {
              }
              frame "AUTO" {
              }
              frame ":AUTO ON" {
              }
              frame "OFF" {
              }
              frame " OFF" {
              }
            }
            n313 = Boolean To (0,1)(Boolean=w466) -> (0, 1=w465:i16)
            n314 = local read "Digits"() -> (w462:i32)
            n315 = local read "AVG"() -> (w461:u32)
            n316 = local read "Att"() -> (w460:dbl)
            n317 = local read "Interval"() -> (w459:dbl)
            n318 = Format Into String(format string="%d %f %f %f %d %d %d %d %f %d %d %f %f %d", initial string=w479, w469, w478, w477, w476, w475, w472, w467, w465, w463, w462, w461, w460, w459, w458) -> (resulting string=w473:refnum<file>, error out=w471:errorcluster)  [unwired: 1 in]
            n319 = Close File(refnum=w473) -> ()  [unwired: 1 in, 2 out]
            n320 = call <vilib>:"Clear Errors.vi"("error in (no error)"=w471) -> ()  [unwired: 6 in, 1 out]
          }
          frame True {
          }
        }
        n321 = local write "N2"(u32 0 ("N2")) -> ()
        n322 = local write "Button10"(FALSE ("Save")) -> ()
      }
      event "ClrGr": Value Change {
        n323 = event-data() -> ()  [unwired: 1 in, 6 out]
        n324 = flat-sequence {
          frame #0 {
            w487 = 1.0 ("X Scale.Range:Minimum")
            w488 = 100.0 ("X Scale.Range:Maximum")
            w489 = dbl[] [] ("History Data")
            n325 = disable-structure shown="Disabled" {
              frame Disabled {
                w495 = ""
                n326 = local write "LogData"(w495) -> ()
                n327 = local write "Histogram"(T4 {"X Values"=[], "Histogram: h(x)"=[]} ("Histogram Graph")) -> ()
                n328 = local write "Stat2"(w495) -> ()
                n329 = local write "Stat1"(w495) -> ()
                n330 = local write "N"(i16 0 ("N")) -> ()
                n331 = local write "Readout"("   ---   " ("Readout")) -> ()
                n332 = local write "Sub1"("Min:     ---   " ("Sub1")) -> ()
                n333 = local write "Sub2"("Max:     ---   " ("Sub2")) -> ()
              }
              frame Enabled {
              }
            }
            n334 = property on="Chart_P" class="WFChart (strict)"("History Data"=w489, "XScale.Maximum"=w488, "XScale.Minimum"=w487) -> ()  [unwired: 2 in, 2 out]
            n335 = property on="Chart_E" class="WFChart (strict)"("History Data"=w489, "XScale.Maximum"=w488, "XScale.Minimum"=w487) -> ()  [unwired: 2 in, 2 out]
            n336 = local write "Frame"(StateMachine."100" ("Frame")) -> ()
            n337 = property on="YT" class="XYGraph (strict)"("Value"=cluster{timestamp[], dbl[]} {[timestamp(3408217200 s since 1904-01-01)], []} ("YT")) -> ()  [unwired: 2 in, 2 out]
          }
          frame #1 {
            n338 = local write "ClrGr"(FALSE ("ClrGr")) -> ()
          }
        }
      }
      event "Imp": Value Change {
        # "Import Logging Data"
        n339 = event-data() -> ("NewVal"=w499:bool)  [unwired: 1 in, 5 out]
        n340 = Equal?(x=w499, y=TRUE) -> (x = y?=w498:bool)
        n341 = case shown="True" w498 {
          frame False {
          }
          frame True {
            n342 = local read "LFP"() -> (w504:path)
            n343 = Strip Path(path=w504) -> (name=w503:string)  [unwired: 1 out]
            n344 = call "File Dialog4"("start path"=w504, "default name"=w503) -> ("selected path"=w506:path, "cancelled"=w507:bool, "error out"=w502:errorcluster)  [unwired: 10 in, 1 out]
            n345 = call <vilib>:"Clear Errors.vi"("error in (no error)"=w502) -> ()  [unwired: 6 in, 1 out]
            n346 = case shown="False" w507 {
              tunnel: [w509 w511] -> w505
              tunnel: w506 -> [w509 _]
              tunnel: [StateMachine."300" ("Frame") StateMachine."300" ("Frame")] -> w501
              frame False {
              }
              frame True {
                n347 = local read "LFP"() -> (w511:path)
              }
            }
            n348 = local write "LFP"(w505) -> ()
            n349 = local write "Frame"(w501) -> ()
          }
        }
      }
      event "Exp": Value Change {
        # "Export\nData"
        n350 = event-data() -> ()  [unwired: 1 in, 6 out]
        n351 = flat-sequence {
          frame #0 {
            n352 = local read "Data_Dir"() -> (w512:path)
            n353 = call "File Dialog3"("start path"=w512, "prompt"="PM100 LogData" ("default name"), "default name"="PM_LogData", "pattern (all files)"="*.txt", "pattern label"="Textfile") -> ("selected path"=w513:path, "cancelled"=w519:bool, "error out"=w520:errorcluster)  [unwired: 7 in, 1 out]
            n354 = local read "LogData"() -> (w517:string)
            n355 = Open/Create/Replace File(file path (use dialog)=w513, error in=w520, operation (0:open)=T3."replace or create with confirmation") -> (refnum out=w518:refnum<file>, error out=w523:errorcluster)  [unwired: 3 in, 1 out]
            n356 = local write "LFP"(w513) -> ()
            n357 = case shown="False" w519 {
              tunnel: w517 -> [w525 _]
              tunnel: w518 -> [w528 _]
              frame False {
                n358 = Format Into String(format string="%s", initial string=w528, w525) -> (resulting string=w527:refnum<file>)  [unwired: 1 in, 1 out]
                n359 = Close File(refnum=w527) -> ()  [unwired: 1 in, 2 out]
              }
              frame True {
              }
            }
            n360 = call <vilib>:"Clear Errors.vi"("error in (no error)"=w523) -> ()  [unwired: 6 in, 1 out]
            n361 = local write "N2"(u32 0 ("N2")) -> ()
          }
          frame #1 {
            n362 = local write "Exp"(FALSE ("Exp")) -> ()
          }
        }
      }
      event "Print": Value Change {
        w531 = T18 0 items=["Quick Print", "Standard Report", "HTML"] ("report type (Quick Print)")
        w533 = T19 0 items=["Complete front panel", "Visible portion of front panel", "Icon, description, panel and diagram", "Documentation: Using the panel", "Documentation: Using as a subVI", "Documentation: Complete", "Documentation: Custom"] ("contents (complete front panel)")
        # "Print Front-Panel"
        n363 = event-data() -> ()  [unwired: 1 in, 6 out]
        n364 = local write "Print"(FALSE ("Print")) -> ()
        n365 = local write "N2"(u32 0 ("N2")) -> ()
        n366 = Current VI's Path() -> (path=w534:path)
        n367 = call-poly <vilib>:"Easy Print VI Panel or Documentation.vi"("layout options"=T5 {"orientation (unchanged)"=0, "panel scaling for page (unchanged)"=0, "margins"={"override VI margins (false)"=FALSE, "margins (1.00)"={"top"=1.0, "left"=1.0, "right"=1.0, "bottom"=1.0}, "measurement system (default)"=0}, "printer options"={"destination printer name (current)"="", "printing method (unchanged)"=0, "color or monochrome (unchanged)"=0}, "page header options"={"page headers (unchanged)"=0, "page header content options"={"Include VI Name"=TRUE, "Include VI Path"=FALSE, "Include Last Modification Date"=FALSE, "Include Date Printed"=TRUE, "Include Page Number"=FALSE, "Include VI Icon"=FALSE}}}, "report type (Quick Print)"=w531, "contents (complete front panel)"=w533, "VI path"=w534) -> ()  [unwired: 6 in, 2 out]
      }
      event "Stop": Value Change {
        n368 = event-data() -> ("NewVal"=w537:bool)  [unwired: 1 in, 5 out]
        n369 = local write "Frame"(StateMachine."Stop" ("Frame")) -> ()
      }
      event Panel Close {
        n370 = event-data() -> ()  [unwired: 1 in, 3 out]
        n371 = flat-sequence {
          tunnel: TRUE ("y") -> [w580]
          tunnel: [FALSE ("Button8")] -> w539
          tunnel: [TRUE] -> w538
          frame #0 {
            w558 = "B" ("section")
            w544 = "A" ("section")
            n372 = Current VI's Path() -> (path=w564:path)
            n373 = local write "Stop"(w580) -> ()
            n374 = local read "Data_Dir"() -> (w547:path)
            n375 = local read "PM100D"() -> (w582:refnum<visa-resource-name>)
            n376 = local write "Frame"(StateMachine."Stop" ("Frame")) -> ()
            n377 = call "PM100D_Close.vi"("VISA resource name"=w582) -> ()  [unwired: 3 in]
            n378 = Build Path(base path=w547, name or relative path="PM100D-ini.cfg") -> (appended path=w579:path)
            n379 = local read "SensType"() -> (w567:i32)
            n380 = local read "Digits"() -> (w576:i32)
            n381 = call <vilib>:"Open Config Data (compatibility).vi"("configuration file path"=w579) -> ("refnum"=w571:T17)  [unwired: 8 in, 2 out]
            n382 = Equal?(x=w567, y=3) -> (x = y?=w565:bool)
            n383 = local read "MainUnits"() -> (w554:enum16{"W", "V", "J", "dBm", "A"})
            n384 = call-poly <vilib>:"Write Key.vi"("section"=w544, "value"=w576, "key"="Digits", "refnum"=w571) -> ("refnum out"=w573:T17)  [unwired: 5 in, 2 out]
            n385 = case shown="False" w565 {
              tunnel: [w585 w592] -> w575
              tunnel: w573 -> [w590 w592]
              tunnel: w544 -> [w588 _]
              tunnel: w544 -> [w583 _]
              frame False {
                n386 = local read "Interval"() -> (w591:dbl)
                n387 = call-poly <vilib>:"Write Key.vi"("section"=w588, "value"=w591, "key"="Intvl", "refnum"=w590) -> ("refnum out"=w584:T17)  [unwired: 5 in, 2 out]
                n388 = local read "AVG"() -> (w587:u32)
                n389 = call-poly <vilib>:"Write Key.vi"("section"=w583, "value"=w587, "key"="Avg", "refnum"=w584) -> ("refnum out"=w585:T17)  [unwired: 5 in, 2 out]
              }
              frame True {
              }
            }
            n390 = local read "Sub1"() -> (w552:enum16{"Off", "Min", "Freq", "Temp", "Res"})
            n391 = local read "Sub2"() -> (w553:enum16{"Off", "Max", "Ratio", "Area", "Second"})
            n392 = local read "Samples"() -> (w577:u32)
            n393 = call-poly <vilib>:"Write Key.vi"("section"=w544, "value"=w577, "key"="Samp", "refnum"=w575) -> ("refnum out"=w562:T17)  [unwired: 5 in, 2 out]
            n394 = local read "LTM"() -> (w549:bool)
            n395 = local read "Int."() -> (w569:i32)
            n396 = local read "NPL"() -> (w542:i32)
            n397 = call-poly <vilib>:"Write Key.vi"("section"=w544, "value"=w569, "key"="Int", "refnum"=w562) -> ("refnum out"=w563:T17)  [unwired: 5 in, 2 out]
            n398 = call "Write_PanelBounds.vi"("refnum in"=w563, "path"=w564) -> ("refnum out"=w561:T17)
            n399 = call-poly <vilib>:"Write Key.vi"("section"=w558, "value"=w554, "key"="Main", "refnum"=w561) -> ("refnum out"=w560:T17)  [unwired: 5 in, 2 out]
            n400 = call-poly <vilib>:"Write Key.vi"("section"=w558, "value"=w552, "key"="Sub1", "refnum"=w560) -> ("refnum out"=w559:T17)  [unwired: 5 in, 2 out]
            n401 = call-poly <vilib>:"Write Key.vi"("section"=w558, "value"=w553, "key"="Sub2", "refnum"=w559) -> ("refnum out"=w550:T17)  [unwired: 5 in, 2 out]
            n402 = call-poly <vilib>:"Write Key.vi"("section"=w544, "value"=w549, "key"="LTM", "refnum"=w550) -> ("refnum out"=w546:T17)  [unwired: 5 in, 2 out]
            n403 = call-poly <vilib>:"Write Key.vi"("section"=w544, "value"=w542, "key"="NPL", "refnum"=w546) -> ("refnum out"=w545:T17)  [unwired: 5 in, 2 out]
            n404 = call <vilib>:"Close Config Data.vi"("refnum"=w545) -> ()  [unwired: 9 in, 2 out]
          }
        }
        n405 = Quit LabVIEW(quit? (T)=w538) -> ()
        n406 = local write "Button8"(w539) -> ()
      }
    }
  }
  n407 = while {
    shift-right: [w593] -> _
    shift-left: StateMachine."Initialize" ("Beginning State") -> [w594]
    stop <- w595 stop-if-true
    n408 = case shown="\"Initialize\", Default" w594 {
      tunnel: [w605 w765 StateMachine."100" ("Beginning State") w1007 w1297 w1639 w1743 w2007 StateMachine."100" ("Beginning State") StateMachine."100" ("Beginning State") w2178 StateMachine."100" ("Beginning State") StateMachine."100" ("Beginning State") StateMachine."100" ("Beginning State") StateMachine."Stop" ("Beginning State")] -> w593
      frame "Initialize", Default {
        w597 = FALSE ("Visible")
        w599 = 1.0 ("X Scale.Range:Minimum")
        w600 = 100.0 ("X Scale.Range:Maximum")
        w601 = dbl[] [] ("History Data")
        w602 = u32 0 ("N2")
        w608 = FALSE ("File?")
        n409 = flat-sequence {
          tunnel: [w689] -> w603
          frame #0 {
            w623 = T20 2 items=["User Home"=0, "User Desktop"=1, "User Documents"=2, "User Application Data"=3, "User Preferences"=4, "User Temporary"=5, "Public Documents"=6, "Public Application Data"=7, "Public Preferences"=8, "Public Cache"=13, "System Core Libraries"=9, "System Installed Libraries"=10, "Application Files"=11, "Boot Volume Root"=12] ("system directory type")
            w632 = 1
            w640 = "B" ("section")
            w614 = "A" ("section")
            # "Load Config File"
            n410 = call <vilib>:"Get System Directory.vi"("create directory if not found? (F)"=TRUE, "system directory type"=w623) -> ("system directory"=w622:path)  [unwired: 9 in]
            n411 = Build Path(base path=w622, name or relative path="Thorlabs\\Powermeter") -> (appended path=w620:path)
            n412 = call <vilib>:"Check if File or Folder Exists.vi"("path"=w620) -> ("file or folder exists?"=w619:bool, "dup path"=w618:path)  [unwired: 8 in, 1 out]
            n413 = case shown="True" w619 {
              tunnel: [w678 w679] -> w617
              tunnel: w618 -> [w677 w679]
              frame False {
                n414 = Create Folder(path (use dialog)=w677) -> (created path=w678:path)  [unwired: 2 in, 2 out]
              }
              frame True {
              }
            }
            n415 = Build Path(base path=w617, name or relative path="PM-Utility-ini.cfg") -> (appended path=w659:path)
            n416 = call <vilib>:"Open Config Data (compatibility).vi"("configuration file path"=w659) -> ("error out"=w668:errorcluster, "refnum"=w676:T17)  [unwired: 8 in, 1 out]
            n417 = local write "Data_Dir"(w617) -> ()
            n418 = property class="App"() -> ("App.Kind"=w627:T21)  [unwired: 2 in, 2 out]
            n419 = call-poly <vilib>:"Read Key.vi"("section"=w614, "error in (no error)"=w668, "default value"=4, "key"="Digits", "refnum"=w676) -> ("error out"=w667:errorcluster, "value"=w664:i32, "refnum out"=w673:T17)  [unwired: 3 in, 1 out]
            n420 = local write "Digits"(w664) -> ()
            n421 = case shown="\"Run Time System\"" w627 {
              tunnel: [w681 w687] -> w626
              tunnel: [w680 w688] -> w625
              frame "Development System", Default {
                n422 = Current VI's Path() -> (path=w680:path)
                n423 = Strip Path(path=w680) -> (stripped path=w681:path)  [unwired: 1 out]
              }
              frame "Run Time System" {
                n424 = Current VI's Path() -> (path=w688:path)
                n425 = Open Application Reference() -> (0:w686:errorcluster, 3:w685:refnum<vi>)  [unwired: 4 in]
                n426 = property class="App"(reference=w685, error in=w686) -> (reference out=w683:refnum<vi>, error out=w684:errorcluster, "App.Dir"=w687:path)
                n427 = Close Reference(reference=w683, error in (no error)=w684) -> (error out=w682:errorcluster)
                n428 = call <vilib>:"Simple Error Handler.vi"("error in (no error)"=w682) -> ()  [unwired: 4 in, 5 out]
              }
            }
            n429 = call-poly <vilib>:"Read Key.vi"("section"=w614, "error in (no error)"=w667, "default value"=1000.0, "key"="Intvl", "refnum"=w673) -> ("error out"=w666:errorcluster, "value"=w663:dbl, "refnum out"=w671:T17)  [unwired: 3 in, 1 out]
            n430 = local write "Interval"(w663) -> ()
            n431 = call-poly <vilib>:"Read Key.vi"("section"=w614, "error in (no error)"=w666, "default value"=100, "key"="Samp", "refnum"=w671) -> ("error out"=w665:errorcluster, "value"=w662:i32, "refnum out"=w670:T17)  [unwired: 3 in, 1 out]
            n432 = local write "Samples"(w662) -> ()
            n433 = call-poly <vilib>:"Read Key.vi"("section"=w614, "error in (no error)"=w665, "default value"=100, "key"="Avg", "refnum"=w670) -> ("error out"=w656:errorcluster, "value"=w661:i32, "refnum out"=w658:T17)  [unwired: 3 in, 1 out]
            n434 = local write "AVG"(w661) -> ()
            n435 = local read "LTM"() -> (w628:bool)
            n436 = call-poly <vilib>:"Read Key.vi"("section"=w614, "error in (no error)"=w656, "default value"=10, "key"="Int", "refnum"=w658) -> ("error out"=w657:errorcluster, "value"=w654:i32, "refnum out"=w653:T17)  [unwired: 3 in, 1 out]
            n437 = call "Read_PanelBounds.vi"("bot"=720, "top"=100, "right"=1170, "left"=200, "path"=w625, "refnum in"=w653) -> ("refnum out"=w643:T17)  [unwired: 5 in]
            n438 = call-poly <vilib>:"Read Key.vi"("section"=w640, "default value"=0, "key"="Main", "refnum"=w643) -> ("value"=w633:i32, "refnum out"=w642:T17)  [unwired: 4 in, 2 out]
            n439 = local write "MainUnits"(w633) -> ()
            n440 = call-poly <vilib>:"Read Key.vi"("section"=w640, "default value"=w632, "key"="Sub1", "refnum"=w642) -> ("value"=w634:i32, "refnum out"=w641:T17)  [unwired: 4 in, 2 out]
            n441 = local write "Sub1"(w634) -> ()
            n442 = call-poly <vilib>:"Read Key.vi"("section"=w640, "default value"=w632, "key"="Sub2", "refnum"=w641) -> ("value"=w635:i32, "refnum out"=w631:T17)  [unwired: 4 in, 2 out]
            n443 = local write "Sub2"(w635) -> ()
            n444 = call-poly <vilib>:"Read Key.vi"("section"=w614, "default value"=w628, "key"="LTM", "refnum"=w631) -> ("value"=w629:bool, "refnum out"=w616:T17)  [unwired: 4 in, 2 out]
            n445 = local write "LTM"(w629) -> ()
            n446 = call-poly <vilib>:"Read Key.vi"("section"=w614, "default value"=1 ("NPL"), "key"="NPL", "refnum"=w616) -> ("value"=w611:i32, "refnum out"=w615:T17)  [unwired: 4 in, 2 out]
            n447 = local write "Int."(w654) -> ()
            n448 = local write "VI_Path"(w626) -> ()
            n449 = call <vilib>:"Close Config Data.vi"("error in (no error)"=w657, "refnum"=w615) -> ()  [unwired: 8 in, 2 out]
            n450 = local write "NPL"(w611) -> ()
          }
          frame #1 {
            # "Chose Instrument \nand Initialize"
            n451 = call "PM100D_Initialize.vi"() -> ("error out"=w690:errorcluster, "Instrument"=w692:string, "VISA out"=w693:refnum<visa-resource-name>, "SN"=w691:string)  [unwired: 2 in]
            n452 = local write "PM100D"(w693) -> ()
            n453 = local write "Flag0"(w692) -> ()
            n454 = local write "Flag1"(w691) -> ()
            n455 = Unbundle By Name(w690) -> ("status"=w689:bool)
          }
        }
        n456 = local write "Button6"(w608) -> ()
        n457 = local write "Button7"(w608) -> ()
        n458 = local write "File?"(w608) -> ()
        n459 = local write "Setup"("PM Setup" ("Setup")) -> ()
        n460 = property on="Chart_P" class="WFChart (strict)"("History Data"=w601, "XScale.Maximum"=w600, "XScale.Minimum"=w599) -> ()  [unwired: 2 in, 2 out]
        n461 = local write "Range Array"(string[] ["AUTO", "50nA", "500nA", "5uA", "50uA", "500uA", "5mA"] ("Range Array")) -> ()
        n462 = local write "Frame"(StateMachine."100" ("Frame")) -> ()
        n463 = local write "N2"(w602) -> ()
        n464 = local write "N"(w602) -> ()
        n465 = property on="Chart_E" class="WFChart (strict)"("History Data"=w601, "XScale.Maximum"=w600, "XScale.Minimum"=w599) -> ()  [unwired: 2 in, 2 out]
        n466 = property on="Splitter" class="Splitter"("Position"=285 ("Splitter Position")) -> ()  [unwired: 2 in, 2 out]
        n467 = property on="YT" class="XYGraph (strict)"("Visible"=w597) -> ()  [unwired: 2 in, 2 out]
        n468 = property on="YT" class="XYGraph (strict)"("Value"=cluster{timestamp[], dbl[]} {[timestamp(3408217200 s since 1904-01-01)], []} ("YT")) -> ()  [unwired: 2 in, 2 out]
        n469 = property on="Chart_P" class="WFChart (strict)"("Visible"=w597) -> ()  [unwired: 2 in, 2 out]
        n470 = Select(t=StateMachine."Stop", s=w603, f=StateMachine."Load Settings" ("Beginning State")) -> (s? t:f=w605:T1)
      }
      frame "Load Settings" {
        n471 = local read "PM100D"() -> (w826:refnum<visa-resource-name>)
        n472 = local read "Flag0"() -> (w753:string)
        n473 = local read "NPL"() -> (w703:i32)
        n474 = local read "LTM"() -> (w760:bool)
        n475 = Spreadsheet String To Array(delimiter (Tab)=",", format string="%s", spreadsheet string=w753, array type (2D Dbl)=string[] [] ("Rng_Array")) -> (array=w754:string[])
        n476 = call "PM100D_Read.vi"("Command"="SYST:SENS:IDN?", "VISA in"=w826) -> ("error out"=w764:errorcluster, "ReadValue"=w778:string, "VISA out"=w797:refnum<visa-resource-name>)  [unwired: 2 in]
        n477 = local write "Readout"("   ---   " ("Readout")) -> ()
        n478 = local write "Sub1"("Min:     ---   " ("Sub1")) -> ()
        n479 = local write "Sub2"("Max:     ---   " ("Sub2")) -> ()
        n480 = Index Array(array=w754, index #1=1 ("index"), index #2=2 ("index"), index #3=3 ("index")) -> (element #1=w749:string, element #2=w699:string, element #3=w698:string)
        n481 = Match Pattern(string=w749, regular expression="PM") -> (match substring=w745:string, after substring=w748:string)  [unwired: 1 in, 2 out]
        n482 = Scan String For Tokens(9:w748) -> (1:w746:string)  [unwired: 5 in, 3 out]
        n483 = Concatenate Strings(w745, w746) -> (w700:string)
        n484 = Equal?(x=w700, y="PM100USB") -> (x = y?=w758:bool)
        n485 = Equal?(x=w700, y="PM200") -> (x = y?=w742:bool)
        n486 = Select(t=FALSE, s=w758, f=w760) -> (s? t:f=w762:bool)
        n487 = String Subset(string=w700, length (rest)=4 ("length (rest)")) -> (substring=w707:string)  [unwired: 1 in]
        n488 = Equal?(x=w707, y="PM16") -> (x = y?=w694:bool)
        n489 = local write "16"(w694) -> ()
        n490 = Select(t=w703, s=w694, f=1) -> (s? t:f=w705:i32)
        n491 = local write "LTM"(w762) -> ()
        n492 = local write "NPL"(w705) -> ()
        n493 = Not(x=w758) -> (.not. x?=w759:bool)
        n494 = call <vilib>:"Clear Errors.vi"("error in (no error)"=w764) -> ()  [unwired: 6 in, 1 out]
        n495 = Unbundle By Name(w764) -> ("status"=w766:bool)
        n496 = property on="LTM" class="Bool (strict)"("Visible"=w759) -> ()  [unwired: 2 in, 2 out]
        n497 = local read "Data_Dir"() -> (w710:path)
        n498 = case shown="True" w742 {
          tunnel: [FALSE w840] -> w741
          frame False {
            n499 = local write "EMM"(FALSE ("EMM")) -> ()
          }
          frame True {
            n500 = local read "PM100D"() -> (w844:refnum<visa-resource-name>)
            n501 = call "PM100D_Read.vi"("Command"="SENS3:TEMP:DATA?" ("write buffer"), "VISA in"=w844) -> ("error out"=w839:errorcluster, "ReadValue"=w842:string)  [unwired: 2 in, 1 out]
            n502 = call <vilib>:"Clear Errors.vi"("error in (no error)"=w839) -> ()  [unwired: 6 in, 1 out]
            n503 = Not Equal?(x=w842, y="") -> (x != y?=w840:bool)
            n504 = local write "EMM"(w840) -> ()
          }
        }
        n505 = call "PM100D_GetRngIndex.vi"("VISA in"=w797) -> ("error out"=w799:errorcluster, "SensType"=w788:i32, "Rng_Array"=w798:string[], "dup VISA session"=w800:refnum<visa-resource-name>, "IndexOut"=w796:i32, "AutoOut"=w792:bool)  [unwired: 5 in]
        n506 = Build Path(base path=w710, name or relative path="PM_LogData.txt") -> (appended path=w739:path)
        n507 = Format Into String(format string="%s  SN:%s  Firmware: %s", initial string="", w700, w699, w698) -> (resulting string=w697:string)  [unwired: 1 in, 1 out]
        n508 = Equal?(x=3, y=w788) -> (x = y?=w791:bool)
        n509 = Spreadsheet String To Array(delimiter (Tab)=",", format string="%s", spreadsheet string=w778, array type (2D Dbl)=string[] [] ("Rng_Array")) -> (array=w820:string[])
        n510 = case shown="False" w791 {
          tunnel: ["W" ("input 2") "J" ("t")] -> w790
          tunnel: ["POW" ("t") "ENER" ("t")] -> w789
          tunnel: [w935 u32 1 ("AVG")] -> w720
          tunnel: [w937 60000.0 ("x")] -> w774
          tunnel: w694 -> [w933 _]
          frame False {
            n511 = local read "Interval"() -> (w937:dbl)
            n512 = local read "AVG"() -> (w936:u32)
            n513 = local read "NPL"() -> (w934:i32)
            n514 = Select(t=w934, s=w933, f=w936) -> (s? t:f=w935:u32)
          }
          frame True {
          }
        }
        n515 = Open/Create/Replace File(file path (use dialog)=w739, operation (0:open)=T3."replace or create") -> (refnum out=w735:refnum<file>)  [unwired: 4 in, 2 out]
        n516 = call "PM100D_SetRngIndex.vi"("PM16"=w694, "VISAin"=w800, "Unit"=w789, "AUTO"=w792, "error in"=w799, "SensType"=w788, "Rng_Array"=w798, "Index"=w796) -> ("VISAout"=w719:refnum<visa-resource-name>, "lblRange"=w793:string, "Numeric 2"=w795:dbl, "AUTO?"=w794:bool, "error out 2"=w706:errorcluster)  [unwired: 3 in]
        n517 = Index Array(array=w820, index #1=0 ("index"), index #2=1 ("index"), index #3=4 ("index"), index #4=5 ("index")) -> (element #1=w787:string, element #2=w815:string, element #3=w784:string, element #4=w782:string)
        n518 = Format Into String(format string="%s  SN:%s  Firmware: %s -- Sensor: %s  SN:%s", initial string="", w700, w699, w698, w787, w815) -> (resulting string=w696:string)  [unwired: 1 in, 1 out]
        n519 = Select(t=w697, s=w694, f=w696) -> (s? t:f=w695:string)
        n520 = local write "Header"(w695) -> ()
        n521 = Concatenate Strings(w695, "\r\n") -> (w733:string)
        n522 = Write to Text File(file (use dialog)=w735, text=w733) -> (refnum out=w734:refnum<file>)  [unwired: 2 in, 2 out]
        n523 = local write "FileRefnum"(w734) -> ()
        n524 = Refnum to Path(1:w734) -> (0:w737:path)
        n525 = Equal?(x=w787, y="no sensor") -> (x = y?=w767:bool)
        n526 = call "PM100D_SensIDNFlag.vi"("String"=w782) -> ("Wave?"=w732:bool, "Tau?"=w779:bool, "Temp?"=w781:bool)  [unwired: 4 out]
        n527 = local write "Wav"(w732) -> ()
        n528 = local write "LFP"(w737) -> ()
        n529 = Format Into String(format string="%s%s", initial string="Range ", w793, w790) -> (resulting string=w813:string)  [unwired: 1 in, 1 out]
        n530 = Divide(x=1000.0, y=w795) -> (x/y=w808:dbl)
        n531 = Or(x=w767, y=w766) -> (x .or. y?=w768:bool)
        n532 = Not Equal?(x=w784, y="1") -> (x != y?=w780:bool)
        n533 = local write "SlideMulti"(w808) -> ()
        n534 = property on="Button1" class="Bool (strict)"("BoolText.Text"=w813) -> ()  [unwired: 2 in, 2 out]
        n535 = case shown="True" w694 {
          tunnel: [w832 w836] -> w822
          tunnel: [w830 1.0] -> w744
          tunnel: w719 -> [w829 w836]
          tunnel: w706 -> [w828 _]
          frame False {
            n536 = call "PM100D_Read.vi"("error in (no error)"=w828, "Command"="SENS:CORR:BEAM?", "VISA in"=w829) -> ("error out"=w827:errorcluster, "ReadValue"=w833:string, "VISA out"=w832:refnum<visa-resource-name>)  [unwired: 1 in]
            n537 = call <vilib>:"Clear Errors.vi"("error in (no error)"=w827) -> ()  [unwired: 6 in, 1 out]
            n538 = Fract/Exp String To Number(use system decimal point (T)=FALSE, string=w833) -> (number=w830:dbl)  [unwired: 2 in, 1 out]
          }
          frame True {
          }
        }
        n539 = local write "Temp"(w781) -> ()
        n540 = local write "Sensor?"(w780) -> ()
        n541 = local write "Tau?"(w779) -> ()
        n542 = case shown="True" w768 {
          tunnel: [StateMachine."20" ("Beginning State") w847] -> w765
          frame False {
          }
          frame True {
            n543 = call "Dialog_NoSensor.vi"() -> ("Cancel"=w849:bool)  [unwired: 5 in, 1 out]
            n544 = Select(t=StateMachine."Load Settings", s=w849, f=StateMachine."Stop" ("Beginning State")) -> (s? t:f=w847:T1)
          }
        }
        n545 = local write "AUTO?"(w794) -> ()
        n546 = local write "SensType"(w788) -> ()
        n547 = property on="EMM" class="Bool (strict)"("Visible"=w741) -> ()  [unwired: 2 in, 2 out]
        n548 = local read "Samples"() -> (w804:u32)
        n549 = local read "File?"() -> (w803:bool)
        n550 = case shown="2" w788 {
          tunnel: w822 -> [w853 w863 w910 w924]
          tunnel: [w853 w861 w902 w923] -> w718
          tunnel: w706 -> [w852 w860 w901 w922]
          tunnel: [w852 w859 w883 w921] -> w715
          tunnel: ["OFF" ("f") "OFF" ("f") w889 "OFF" ("f")] -> w721
          tunnel: w720 -> [w850 w855 w880 w917]
          tunnel: [w850 w855 w885 w917] -> w711
          tunnel: w694 -> [_ _ w882 _]
          frame 0, Default {
          }
          frame 1 {
            n551 = local read "MainUnits"() -> (w858:enum16{"W", "V", "J", "dBm", "A"})
            n552 = local read "16"() -> (w854:bool)
            n553 = case shown="False" w854 {
              tunnel: w863 -> [w868 w872]
              tunnel: [w867 1] -> w862
              tunnel: [w866 w872] -> w861
              tunnel: w860 -> [w865 w873]
              tunnel: [w864 w873] -> w859
              frame False {
                n554 = call "PM100D_Read.vi"("error in (no error)"=w865, "Command"="INP:FILT?", "VISA in"=w868) -> ("error out"=w864:errorcluster, "ReadValue"=w869:string, "VISA out"=w866:refnum<visa-resource-name>)  [unwired: 1 in]
                n555 = Decimal String To Number(string=w869) -> (number=w867:i32)  [unwired: 2 in, 1 out]
              }
              frame True {
              }
            }
            n556 = case shown="\"A\"" w858 {
              tunnel: [enum16{"W", "V", "J", "dBm", "A"}."W" ("MainUnits") enum16{"W", "V", "J", "dBm", "A"}."W" ("MainUnits") enum16{"W", "V", "J", "dBm", "A"}."W" ("MainUnits") enum16{"W", "V", "J", "dBm", "A"}."dBm" ("MainUnits") enum16{"W", "V", "J", "dBm", "A"}."A" ("MainUnits")] -> w857
              frame "W", Default {
              }
              frame "V" {
              }
              frame "J" {
              }
              frame "dBm" {
              }
              frame "A" {
              }
            }
            n557 = local write "MainUnits"(w857) -> ()
            n558 = local write "BW"(w862) -> ()
          }
          frame 2 {
            w887 = "ON"
            w895 = "1\n" ("y")
            n559 = Select(t=w880, s=w882, f=u32 100 ("t")) -> (s? t:f=w879:u32)
            n560 = call "PM100D_Read.vi"("error in (no error)"=w901, "Command"="INP:THER:ACC?", "VISA in"=w910) -> ("error out"=w900:errorcluster, "ReadValue"=w909:string, "VISA out"=w884:refnum<visa-resource-name>)  [unwired: 1 in]
            n561 = call "PM100D_Read.vi"("error in (no error)"=w900, "Command"="INP:THER:ACC:AUTO?", "VISA in"=w884) -> ("error out"=w897:errorcluster, "ReadValue"=w896:string, "VISA out"=w898:refnum<visa-resource-name>)  [unwired: 1 in]
            n562 = call "PM100D_Read.vi"("error in (no error)"=w897, "Command"="INP:THER:ACC:TAU?", "VISA in"=w898) -> ("error out"=w883:errorcluster, "ReadValue"=w904:string, "VISA out"=w902:refnum<visa-resource-name>)  [unwired: 1 in]
            n563 = Equal?(x=w909, y=w895) -> (x = y?=w908:bool)
            n564 = Equal?(x=w896, y=w895) -> (x = y?=w894:bool)
            n565 = Select(t=w887, s=w908, f="OFF") -> (s? t:f=w892:string)
            n566 = Fract/Exp String To Number(use system decimal point (T)=FALSE, string=w904) -> (number=w903:dbl)  [unwired: 2 in, 1 out]
            n567 = local read "MainUnits"() -> (w890:enum16{"W", "V", "J", "dBm", "A"})
            n568 = Select(t=":AUTO ON", s=w894, f=w892) -> (s? t:f=w889:string)
            n569 = Match Pattern(string=w889, regular expression=w887) -> (match substring=w888:string)  [unwired: 1 in, 3 out]
            n570 = Equal?(x=w888, y=w887) -> (x = y?=w886:bool)
            n571 = local write "Tau"(w903) -> ()
            n572 = case shown="\"W\", Default" w890 {
              tunnel: [enum16{"W", "V", "J", "dBm", "A"}."W" ("MainUnits") enum16{"W", "V", "J", "dBm", "A"}."V" ("MainUnits") enum16{"W", "V", "J", "dBm", "A"}."W" ("MainUnits") enum16{"W", "V", "J", "dBm", "A"}."dBm" ("MainUnits") enum16{"W", "V", "J", "dBm", "A"}."W" ("MainUnits")] -> w891
              frame "W", Default {
              }
              frame "V" {
              }
              frame "J" {
              }
              frame "dBm" {
              }
              frame "A" {
              }
            }
            n573 = local write "MainUnits"(w891) -> ()
            n574 = Select(t=w879, s=w886, f=w880) -> (s? t:f=w885:u32)
          }
          frame 3 {
            n575 = local read "MainUnits"() -> (w920:enum16{"W", "V", "J", "dBm", "A"})
            n576 = call "PM100D_Read.vi"("error in (no error)"=w922, "Command"="SENS:PEAK?", "VISA in"=w924) -> ("error out"=w921:errorcluster, "ReadValue"=w926:string, "VISA out"=w923:refnum<visa-resource-name>)  [unwired: 1 in]
            n577 = case shown="\"W\", Default" w920 {
              tunnel: [enum16{"W", "V", "J", "dBm", "A"}."J" ("MainUnits") enum16{"W", "V", "J", "dBm", "A"}."V" ("MainUnits") enum16{"W", "V", "J", "dBm", "A"}."J" ("MainUnits") enum16{"W", "V", "J", "dBm", "A"}."J" ("MainUnits") enum16{"W", "V", "J", "dBm", "A"}."J" ("MainUnits")] -> w919
              frame "W", Default {
              }
              frame "V" {
              }
              frame "J" {
              }
              frame "dBm" {
              }
              frame "A" {
              }
            }
            n578 = Fract/Exp String To Number(string=w926) -> (number=w927:dbl)  [unwired: 3 in, 1 out]
            n579 = local write "Trig"(w927) -> ()
            n580 = local write "MainUnits"(w919) -> ()
          }
        }
        n581 = property on="Hum" class="Str"("Visible"=w741) -> ()  [unwired: 2 in, 2 out]
        n582 = property on="Temp" class="Str"("Visible"=w741) -> ()  [unwired: 2 in, 2 out]
        n583 = Divide(x=w774, y=1000.0) -> (x/y=w801:dbl)
        n584 = Format Into String(format string="%d", initial string="SENS:AVER " ("Command"), w711) -> (resulting string=w712:string)  [unwired: 1 in, 1 out]
        n585 = local write "Dia"(w744) -> ()
        n586 = Format Into String(format string="Samples:    %d\\nInterval:      %.2fs\\nAveraging: %d\\nLog to File: %s", initial string="Logging Parameters\n", w804, w801, w711, w803) -> (resulting string=w805:string)  [unwired: 1 in, 1 out]
        n587 = local write "LogCfg"(w805) -> ()
        n588 = local write "DiaIni"(w744) -> ()
        n589 = call "PM100D_Write.vi"("error in (no error)"=w715, "Command"=w712, "VISA in"=w718) -> ("error out"=w716:errorcluster, "VISA out"=w717:refnum<visa-resource-name>)
        n590 = call "PM100D_Read.vi"("error in (no error)"=w716, "Command"="SENS:CORR?", "VISA in"=w717) -> ("error out"=w730:errorcluster, "ReadValue"=w726:string, "VISA out"=w731:refnum<visa-resource-name>)  [unwired: 1 in]
        n591 = call "PM100D_Read.vi"("error in (no error)"=w730, "Command"="INP:ADAP?", "VISA in"=w731) -> ("error out"=w769:errorcluster, "ReadValue"=w772:string)  [unwired: 1 in, 1 out]
        n592 = Search 1D Array(1D array=string[] ["PHOT\n", "THER\n", "PYR\n"], element=w772) -> (index of element=w771:i32)  [unwired: 1 in]
        n593 = Fract/Exp String To Number(use system decimal point (T)=FALSE, string=w726) -> (number=w722:dbl)  [unwired: 2 in, 1 out]
        n594 = local write "Adapter"(w771) -> ()
        n595 = local write "Att"(w722) -> ()
        n596 = Format Into String(format string="%.;%.2f %s", initial string="a = ", w722, " dB") -> (resulting string=w724:string)  [unwired: 1 in, 1 out]
        n597 = local write "att"(w724) -> ()
        n598 = local write "AVG"(w711) -> ()
        n599 = local write "ACC"(w721) -> ()
        n600 = call <vilib>:"Clear Errors.vi"("error in (no error)"=w769) -> ()  [unwired: 6 in, 1 out]
      }
      frame "20" {
        n601 = local read "PM100D"() -> (w950:refnum<visa-resource-name>)
        n602 = local read "SensType"() -> (w945:i32)
        n603 = local read "Sensor?"() -> (w949:bool)
        n604 = local read "MainUnits"() -> (w947:enum16{"W", "V", "J", "dBm", "A"})
        n605 = case shown="True" w949 {
          tunnel: [w977 "Wave " ("initial string")] -> w957
          tunnel: [w976 "%dnm" ("format string")] -> w956
          tunnel: [w980 w1000] -> w955
          tunnel: [1e-07 ("WAV_MAX") w999] -> w954
          tunnel: [1000.0 ("WAV_MAX") w998] -> w953
          tunnel: w950 -> [w975 w997]
          tunnel: w945 -> [w974 _]
          tunnel: [w973 w996] -> w948
          frame False {
            # "CORR:POW?\nCORR:POW:THER?\nCORR:ENER?"
            n606 = case shown="0, Default" w974 {
              tunnel: ["" ("format string") "SENS:CORR:POW?" ("format string") "SENS:CORR:POW:THER?" ("format string") "SENS:CORR:ENER?" ("format string")] -> w978
              tunnel: ["" ("initial string") "" ("initial string") "" ("initial string") "" ("initial string")] -> w977
              tunnel: ["" ("format string") "%.;%_3pA/W" ("format string") "%.;%_3pV/W" ("format string") "%.;%_3pV/J" ("format string")] -> w976
              frame 0, Default {
              }
              frame 1 {
              }
              frame 2 {
              }
              frame 3 {
              }
            }
            n607 = call "PM100D_Read.vi"("Command"=w978, "VISA in"=w975) -> ("error out"=w973:errorcluster, "ReadValue"=w981:string)  [unwired: 2 in, 1 out]
            n608 = Fract/Exp String To Number(use system decimal point (T)=FALSE, string=w981) -> (number=w980:dbl)  [unwired: 2 in, 1 out]
          }
          frame True {
            n609 = call "PM100D_Get-Wave.vi"("VISA in"=w997) -> ("WAV_MAX"=w998:dbl, "WAV"=w1000:dbl, "WAV_MIN"=w999:dbl, "error out"=w996:errorcluster)  [unwired: 10 in, 1 out]
          }
        }
        n610 = case shown="\"A\"" w947 {
          tunnel: ["Power / W" w961 "Energy / J" "dBm" "Power / A"] -> w946
          tunnel: w945 -> [_ w962 _ _ _]
          tunnel: [TRUE FALSE TRUE TRUE FALSE] -> w944
          frame "W", Default {
          }
          frame "V" {
            n611 = case shown="0, Default" w962 {
              tunnel: ["" "Power / V" "Power / V" "Energy / V"] -> w961
              frame 0, Default {
              }
              frame 1 {
              }
              frame 2 {
              }
              frame 3 {
              }
            }
          }
          frame "J" {
          }
          frame "dBm" {
          }
          frame "A" {
          }
        }
        n612 = local write "Unit"(w946) -> ()
        n613 = property on="att" class="Str"("Visible"=w944) -> ()  [unwired: 2 in, 2 out]
        n614 = Format Into String(format string=w956, initial string=w957, w955) -> (resulting string=w952:string)  [unwired: 1 in, 1 out]
        n615 = call <vilib>:"Clear Errors.vi"("error in (no error)"=w948) -> ()  [unwired: 6 in, 1 out]
        n616 = local write "LambdaMax"(w953) -> ()
        n617 = property on="Button2" class="Bool (strict)"("BoolText.Text"=w952) -> ()  [unwired: 2 in, 2 out]
        n618 = local write "LambdaMin"(w954) -> ()
        n619 = local write "Lambda"(w955) -> ()
      }
      frame "100" {
        n620 = flat-sequence {
          tunnel: [w1100] -> w1006
          tunnel: [w1099] -> w1005
          tunnel: [w1081] -> w1004
          tunnel: [w1087] -> w1003
          frame #0 {
            n621 = local read "MainUnits"() -> (w1098:enum16{"W", "V", "J", "dBm", "A"})
            n622 = local read "LTM"() -> (w1083:bool)
            n623 = case shown="False" w1083 {
              tunnel: [w1105 w1118] -> w1084
              frame False {
                n624 = local read "Wav"() -> (w1104:bool)
                n625 = case shown="False" w1104 {
                  tunnel: [w1109 w1115] -> w1105
                  frame False {
                    n626 = local read "PM100D"() -> (w1110:refnum<visa-resource-name>)
                    n627 = call "PM100D_Get-Wave.vi"("VISA in"=w1110) -> ("VISA out"=w1109:refnum<visa-resource-name>, "WAV"=w1108:dbl, "error out"=w1107:errorcluster)  [unwired: 10 in, 2 out]
                    n628 = Unbundle By Name(w1107) -> ("status"=w1106:bool)
                    n629 = case shown="False" w1106 {
                      tunnel: w1108 -> [w1112 _]
                      frame False {
                        n630 = Format Into String(format string="%dnm", initial string="Wave ", w1112) -> (resulting string=w1111:string)  [unwired: 1 in, 1 out]
                        n631 = property on="Button2" class="Bool (strict)"("BoolText.Text"=w1111) -> ()  [unwired: 2 in, 2 out]
                        n632 = local write "Lambda"(w1112) -> ()
                      }
                      frame True {
                      }
                    }
                    n633 = call <vilib>:"Clear Errors.vi"("error in (no error)"=w1107) -> ()  [unwired: 6 in, 1 out]
                  }
                  frame True {
                    n634 = local read "PM100D"() -> (w1115:refnum<visa-resource-name>)
                  }
                }
              }
              frame True {
                n635 = local read "PM100D"() -> (w1116:refnum<visa-resource-name>)
                n636 = call "PM100D_Open.vi"("VISA resource name"=w1116) -> ("VISA out"=w1118:refnum<visa-resource-name>, "error out"=w1117:errorcluster)  [unwired: 2 out]
                n637 = call <vilib>:"Clear Errors.vi"("error in (no error)"=w1117) -> ()  [unwired: 6 in, 1 out]
              }
            }
            n638 = call "PM100D_Read.vi"("Command"="SYST:SENS:IDN?", "VISA in"=w1084) -> ("error out"=w1085:errorcluster, "ReadValue"=w1094:string)  [unwired: 2 in, 1 out]
            n639 = case shown="\"A\"" w1098 {
              tunnel: ["VOLT" ("ConfPara") "ENER" ("ConfPara") "POW" ("ConfPara") "CURR" ("ConfPara") "POW" ("ConfPara")] -> w1099
              tunnel: ["V" "J" "dBm" "A" "W"] -> w1082
              frame "V" {
              }
              frame "J" {
              }
              frame "dBm" {
              }
              frame "A" {
              }
              frame "W", Default {
              }
            }
            n640 = local write "Button7"(FALSE ("Button7")) -> ()
            n641 = local read "SensType"() -> (w1097:i32)
            n642 = Unbundle By Name(w1085) -> ("status"=w1088:bool)
            n643 = xnode "Match Regular Expression"("input string"=w1094, "regular expression"=",") -> ("before match"=w1091:string)  [unwired: 4 in, 4 out]
            n644 = local read "PM100D"() -> (w1100:refnum<visa-resource-name>)
            n645 = Equal?(x="no sensor" ("y"), y=w1091) -> (x = y?=w1089:bool)
            n646 = Or(x=w1088, y=w1089) -> (x .or. y?=w1090:bool)
            n647 = case shown="True" w1090 {
              tunnel: [FALSE w1120] -> w1087
              frame False {
              }
              frame True {
                n648 = disable-structure shown="Enabled" {
                  disable-tunnel: [w1121 TRUE ("OK")] -> w1120
                  frame Disabled {
                    n649 = call "Dialog_LostConnection.vi"() -> ("OK"=w1121:bool)  [unwired: 7 in]
                  }
                  frame Enabled {
                  }
                }
              }
            }
            n650 = call <vilib>:"Clear Errors.vi"("error in (no error)"=w1085) -> ()  [unwired: 6 in, 1 out]
            n651 = Equal?(x=w1097, y=3) -> (x = y?=w1081:bool)
            n652 = case shown="True" w1081 {
              tunnel: [0 2] -> w1080
              frame False {
              }
              frame True {
                n653 = property on="YT" class="XYGraph (strict)"("Visible"=FALSE) -> ()  [unwired: 2 in, 2 out]
              }
            }
            n654 = property on="Scale" class="Bool (strict)"("Disabled"=w1080) -> ()  [unwired: 2 in, 2 out]
            n655 = local write "Unt"(w1082) -> ()
          }
        }
        n656 = case shown="False" w1003 {
          tunnel: [w1011 StateMachine."Load Settings" ("Frame")] -> w1007
          tunnel: w1006 -> [w1009 w1078]
          tunnel: w1005 -> [w1010 _]
          tunnel: w1004 -> [w1008 _]
          frame False {
            n657 = case shown="False" w1008 {
              tunnel: [w1013 w1044] -> w1011
              tunnel: w1010 -> [w1027 w1043]
              tunnel: w1008 -> [_ w1038]
              tunnel: w1009 -> [w1028 w1036]
              frame False {
                w1016 = 0 ("t")
                w1015 = 2
                n658 = local read "FastOut"() -> (w1024:bool)
                n659 = local read "Button6"() -> (w1023:bool)
                n660 = Concatenate Strings("CONF:" ("string"), w1027) -> (w1030:string)
                n661 = And(x=w1024, y=w1023) -> (x .and. y?=w1022:bool)
                n662 = local read "XScaleFit"() -> (w1014:bool)
                n663 = local read "YScaleFit"() -> (w1019:bool)
                n664 = local read "YScaleRep"() -> (w1018:bool)
                n665 = call "PM100D_Write.vi"("Command"=w1030, "VISA in"=w1028) -> ("error out"=w1012:errorcluster)  [unwired: 1 in, 1 out]
                n666 = case shown="False" w1022 {
                  tunnel: [StateMachine."120" ("Frame") StateMachine."130" ("Frame")] -> w1013
                  frame False {
                  }
                  frame True {
                    w1033 = "---" ("Sub1")
                    n667 = local write "Sub1"(w1033) -> ()
                    n668 = local write "Sub2"(w1033) -> ()
                    n669 = local write "Readout"("- Acquiring -" ("Readout")) -> ()
                    n670 = local write "Stat0"("Count:" ("Stat0")) -> ()
                  }
                }
                n671 = call <vilib>:"Clear Errors.vi"("error in (no error)"=w1012) -> ()  [unwired: 6 in, 1 out]
                n672 = Select(t=w1016, s=w1014, f=w1015) -> (s? t:f=w1017:i32)
                n673 = Select(t=w1016, s=w1019, f=w1015) -> (s? t:f=w1021:i32)
                n674 = Boolean To (0,1)(Boolean=w1018) -> (0, 1=w1020:i16)
                n675 = property on="Chart_P" class="WFChart (strict)"("XScale.ScaleFit"=w1017, "YScale.ScaleFit"=w1021, "YScale.Mapping Mode"=w1020) -> ()  [unwired: 2 in, 2 out]
                n676 = local write "ARM"(TRUE ("ARM")) -> ()
                n677 = local write "Arm"("T" ("Arm")) -> ()
              }
              frame True {
                n678 = call "PM100D_ConfMeas.vi"("Conf:"=w1043, "VISA In"=w1036) -> ("error out"=w1037:errorcluster, "dup VISA session"=w1042:refnum<visa-resource-name>)  [unwired: 1 in]
                n679 = call <vilib>:"Clear Errors.vi"("error in (no error)"=w1037) -> ()  [unwired: 6 in, 1 out]
                n680 = while {
                  tunnel: w1042 -> [w1075]
                  tunnel: [w1052] -> w1046
                  tunnel: w1038 -> [w1061]
                  i -> [w1064]
                  stop <- w1074 stop-if-true
                  n681 = local read "Button1"() -> (w1073:bool)
                  n682 = local read "Button2"() -> (w1072:bool)
                  n683 = local read "Button3"() -> (w1071:bool)
                  n684 = local read "Button4"() -> (w1070:bool)
                  n685 = local read "Button5"() -> (w1069:bool)
                  n686 = local read "Button8"() -> (w1068:bool)
                  n687 = Select(t=10000, s=w1061, f=2) -> (s? t:f=w1060:i32)
                  n688 = local read "AVG"() -> (w1062:u32)
                  n689 = call "PM100D_Read.vi"("Command"="STAT:OPER:COND?", "VISA in"=w1075) -> ("error out"=w1047:errorcluster, "ReadValue"=w1076:string)  [unwired: 2 in, 1 out]
                  n690 = Unbundle By Name(w1047) -> ("status"=w1048:bool)
                  n691 = Decimal String To Number(string=w1076) -> (number=w1054:i32)  [unwired: 2 in, 1 out]
                  n692 = Multiply(x=w1060, y=w1062) -> (x*y=w1063:u32)
                  n693 = Number To Boolean Array(number=w1054) -> (Boolean array=w1051:bool[])
                  n694 = local read "Button9"() -> (w1056:bool)
                  n695 = local read "Button10"() -> (w1055:bool)
                  n696 = call <vilib>:"Clear Errors.vi"("error in (no error)"=w1047) -> ()  [unwired: 6 in, 1 out]
                  n697 = Equal?(x=w1064, y=w1063) -> (x = y?=w1057:bool)
                  n698 = Rotate 1D Array(1:w1051, 2:0 ("n")) -> (0:w1050:bool[])
                  n699 = Index Array(array=w1050, index=9) -> (element=w1052:bool)
                  n700 = Select(t="T", s=w1052, f="A") -> (s? t:f=w1067:string)
                  n701 = Compound Arithmetic op=OR(w1048, w1052, w1073, w1072, w1071, w1070, w1069, w1068, w1057, w1056, w1055) -> (w1074:bool)
                  n702 = local write "ARM"(w1052) -> ()
                  n703 = local write "Arm"(w1067) -> ()
                }
                n704 = local read "Frame"() -> (w1045:T1)
                n705 = Select(t=StateMachine."140", s=w1038, f=StateMachine."120" ("t")) -> (s? t:f=w1040:T1)
                n706 = Select(t=w1040, s=w1046, f=w1045) -> (s? t:f=w1044:T1)
              }
            }
          }
          frame True {
            n707 = call "PM100D_Close.vi"("VISA resource name"=w1078) -> ()  [unwired: 3 in]
          }
        }
      }
      frame "120" {
        n708 = local read "PM100D"() -> (w1244:refnum<visa-resource-name>)
        n709 = local read "Digits"() -> (w1282:i32)
        n710 = local read "MainUnits"() -> (w1248:enum16{"W", "V", "J", "dBm", "A"})
        n711 = case shown="\"A\"" w1248 {
          tunnel: ["POW?" "ENER?" "VOLT?" "POW?" "CURR?"] -> w1245
          frame "W", Default {
          }
          frame "J" {
          }
          frame "V" {
          }
          frame "dBm" {
          }
          frame "A" {
          }
        }
        n712 = local read "Button6"() -> (w1250:bool)
        n713 = local read "SensType"() -> (w1269:i32)
        n714 = local read "Scale"() -> (w1251:bool)
        n715 = local read "Res"() -> (w1264:bool)
        n716 = local read "Sub1"() -> (w1289:enum16{"Off", "Min", "Freq", "Temp", "Res"})
        n717 = local read "AVG"() -> (w1270:u32)
        n718 = local read "Sub2"() -> (w1288:enum16{"Off", "Max", "Ratio", "Area", "Second"})
        n719 = local read "N2"() -> (w1253:u32)
        n720 = local read "EMM"() -> (w1254:bool)
        n721 = Increment(x=w1253) -> (x+1=w1252:u32)
        n722 = Concatenate Strings("MEAS:" ("Command"), w1245) -> (w1246:string)
        n723 = Equal?(x=w1269, y=3) -> (x = y?=w1273:bool)
        n724 = local write "N2"(w1252) -> ()
        n725 = case shown="True" w1250 {
          tunnel: w1251 -> [w1323 _]
          frame False {
            n726 = property on="Chart_P" class="WFChart (strict)"("Visible"=w1323) -> ()  [unwired: 2 in, 2 out]
            n727 = Not(x=w1323) -> (.not. x?=w1324:bool)
            n728 = property on="YT" class="XYGraph (strict)"("Visible"=w1324) -> ()  [unwired: 2 in, 2 out]
          }
          frame True {
            n729 = property on="Chart_P" class="WFChart (strict)"("Visible"=TRUE) -> ()  [unwired: 2 in, 2 out]
          }
        }
        n730 = case shown="True" w1254 {
          frame True {
            n731 = local read "AVG"() -> (w1329:u32)
            n732 = Greater Or Equal?(x=w1329, y=u32 100) -> (x >= y?=w1330:bool)
            n733 = Divide(x=w1329, y=u32 1000) -> (x/y=w1328:dbl)
            n734 = local read "N2"() -> (w1336:u32)
            n735 = Select(t=w1328, s=w1330, f=0.1) -> (s? t:f=w1326:dbl)
            n736 = Divide(x=u32 3 ("y"), y=w1326) -> (x/y=w1332:dbl)
            n737 = Round Toward +Infinity(x=w1332) -> (ceil(x): smallest int >= x=w1333:dbl)
            n738 = Equal?(x=w1336, y=w1333) -> (x = y?=w1337:bool)
            n739 = case shown="False" w1337 {
              frame False {
              }
              frame True {
                n740 = local read "PM100D"() -> (w1349:refnum<visa-resource-name>)
                n741 = call "PM100D_Read.vi"("Command"="SENS3:TEMP:DATA?" ("write buffer"), "VISA in"=w1349) -> ("error out"=w1339:errorcluster, "ReadValue"=w1345:string, "VISA out"=w1348:refnum<visa-resource-name>)  [unwired: 2 in]
                n742 = Equal?(x="", y=w1345) -> (x = y?=w1346:bool)
                n743 = case shown="False" w1346 {
                  tunnel: w1345 -> [w1360 _]
                  frame False {
                    n744 = Fract/Exp String To Number(use system decimal point (T)=FALSE, string=w1360) -> (number=w1356:dbl)  [unwired: 2 in, 1 out]
                    n745 = local write "T"(w1356) -> ()
                    n746 = Format Into String(format string="%.;%.1f\\B0C", w1356) -> (resulting string=w1358:string)  [unwired: 2 in, 1 out]
                    n747 = local write "Temp"(w1358) -> ()
                  }
                  frame True {
                  }
                }
                n748 = call "PM100D_Read.vi"("error in (no error)"=w1339, "Command"="SENS2:HUM:DATA?" ("write buffer"), "VISA in"=w1348) -> ("error out"=w1344:errorcluster, "ReadValue"=w1341:string)  [unwired: 1 in, 1 out]
                n749 = call <vilib>:"Clear Errors.vi"("error in (no error)"=w1344) -> ()  [unwired: 6 in, 1 out]
                n750 = Equal?(x=w1341, y="") -> (x = y?=w1342:bool)
                n751 = case shown="False" w1342 {
                  tunnel: w1341 -> [w1352 _]
                  frame False {
                    n752 = Fract/Exp String To Number(use system decimal point (T)=FALSE, string=w1352) -> (number=w1351:dbl)  [unwired: 2 in, 1 out]
                    n753 = Format Into String(format string="%.;%.1f%", w1351) -> (resulting string=w1354:string)  [unwired: 2 in, 1 out]
                    n754 = local write "Hum"(w1354) -> ()
                    n755 = local write "H"(w1351) -> ()
                  }
                  frame True {
                  }
                }
                n756 = local write "N2"(u32 0 ("N2")) -> ()
              }
            }
          }
          frame False {
          }
        }
        n757 = disable-structure shown="Enabled" {
          disable-tunnel: [w1306 w1313] -> w1262
          disable-tunnel: [w1302 w1314] -> w1261
          disable-tunnel: [w1301 w1310] -> w1249
          disable-tunnel: w1246 -> [w1299 w1311]
          disable-tunnel: w1244 -> [w1298 w1312]
          frame Disabled {
            n758 = call "PM100D_Read.vi"("Command"=w1299, "VISA in"=w1298) -> ("error out"=w1300:errorcluster, "ReadValue"=w1306:string)  [unwired: 2 in, 1 out]
            n759 = Unbundle By Name(w1300) -> ("status"=w1301:bool)
            n760 = call <vilib>:"Clear Errors.vi"("error in (no error)"=w1300) -> ()  [unwired: 6 in, 1 out]
            n761 = Equal?(x="9.9E37\n", y=w1306) -> (x = y?=w1304:bool)
            n762 = Equal?(x="-9.9E37\n", y=w1306) -> (x = y?=w1305:bool)
            n763 = Build Array(w1304, w1305) -> (w1303:bool[])
            n764 = Boolean Array To Number(Boolean array=w1303) -> (number=w1302:u32)
          }
          frame Enabled {
            n765 = local read "NPL"() -> (w1309:i32)
            n766 = call "PM100D_Meas_NPLC.vi"("Command"=w1311, "NCPL"=w1309, "VISA Refnum in"=w1312) -> ("Error"=w1310:bool, "Value"=w1313:string, "INF"=w1314:u32)  [unwired: 5 in, 1 out]
          }
        }
        n767 = case shown="True" w1249 {
          tunnel: w1244 -> [_ w1322]
          frame False {
          }
          frame True {
            n768 = VISA Clear(VISA resource name=w1322) -> (error out=w1320:errorcluster)  [unwired: 1 in, 1 out]
            n769 = call <vilib>:"Clear Errors.vi"("error in (no error)"=w1320) -> ()  [unwired: 6 in, 1 out]
            n770 = local write "Readout"("High") -> ()
          }
        }
        n771 = case shown="0, Default" w1261 {
          tunnel: [w1370 w1408 w1417] -> w1284
          tunnel: w1282 -> [w1369 _ _]
          tunnel: [w1363 w1407 w1416] -> w1275
          tunnel: w1248 -> [w1368 w1409 w1418]
          tunnel: [w1363 w1407 w1416] -> w1268
          tunnel: [w1367 "High     " "Low      "] -> w1263
          tunnel: w1262 -> [w1364 _ _]
          tunnel: [w1362 w1407 w1416] -> w1258
          frame 0, Default {
            n772 = Number To Decimal String(number=w1369) -> (decimal integer string=w1365:string)  [unwired: 1 in]
            n773 = case shown="\"W\", Default" w1368 {
              tunnel: [w1375 w1382 w1389 w1397 w1404] -> w1366
              tunnel: [w1372 w1379 w1386 w1396 w1401] -> w1363
              tunnel: w1365 -> [w1376 w1383 w1390 w1398 w1405]
              tunnel: [w1374 w1381 w1388 w1395 w1403] -> w1370
              tunnel: [w1372 w1379 w1386 w1393 w1401] -> w1362
              tunnel: w1364 -> [w1371 w1378 w1385 w1392 w1400]
              frame "W", Default {
                w1374 = "pW" ("string")
                n774 = Fract/Exp String To Number(use system decimal point (T)=FALSE, string=w1371) -> (number=w1372:dbl)  [unwired: 2 in, 1 out]
                n775 = Concatenate Strings("%.;%_" ("string"), w1376, w1374) -> (w1375:string)
              }
              frame "V" {
                w1381 = "pV" ("string")
                n776 = Fract/Exp String To Number(use system decimal point (T)=FALSE, string=w1378) -> (number=w1379:dbl)  [unwired: 2 in, 1 out]
                n777 = Concatenate Strings("%.;%_" ("string"), w1383, w1381) -> (w1382:string)
              }
              frame "J" {
                w1388 = "pJ" ("string")
                n778 = Fract/Exp String To Number(use system decimal point (T)=FALSE, string=w1385) -> (number=w1386:dbl)  [unwired: 2 in, 1 out]
                n779 = Concatenate Strings("%.;%_" ("string"), w1390, w1388) -> (w1389:string)
              }
              frame "dBm" {
                w1395 = "fdBm" ("string")
                n780 = Fract/Exp String To Number(use system decimal point (T)=FALSE, string=w1392) -> (number=w1393:dbl)  [unwired: 2 in, 1 out]
                n781 = call "lin-log.vi"("W In 2"=w1393) -> ("dBm Out 2"=w1396:dbl)  [unwired: 3 in, 3 out]
                n782 = Concatenate Strings("%.;%_" ("string"), w1398, w1395) -> (w1397:string)
              }
              frame "A" {
                w1403 = "pA" ("string")
                n783 = Fract/Exp String To Number(use system decimal point (T)=FALSE, string=w1400) -> (number=w1401:dbl)  [unwired: 2 in, 1 out]
                n784 = Concatenate Strings("%.;%_" ("string"), w1405, w1403) -> (w1404:string)
              }
            }
            n785 = Format Into String(format string=w1366, w1363) -> (resulting string=w1367:string, error out=w1361:errorcluster)  [unwired: 2 in]
            n786 = call <vilib>:"Clear Errors.vi"("error in (no error)"=w1361) -> ()  [unwired: 6 in, 1 out]
          }
          frame 1 {
            w1407 = 0.0
            n787 = case shown="\"dBm\"" w1409 {
              tunnel: ["W" ("string") "V" ("string") "J" ("string") "A" ("string") "dBm" ("string")] -> w1408
              frame "W", Default {
              }
              frame "V" {
              }
              frame "J" {
              }
              frame "A" {
              }
              frame "dBm" {
              }
            }
          }
          frame 2 {
            w1416 = 0.0
            n788 = case shown="\"A\"" w1418 {
              tunnel: ["W" ("string") "V" ("string") "J" ("string") "A" ("string") "dBm" ("string")] -> w1417
              frame "W", Default {
              }
              frame "V" {
              }
              frame "J" {
              }
              frame "A" {
              }
              frame "dBm" {
              }
            }
          }
        }
        n789 = call <vilib>:"Array Max & Min PtByPt.vi"("input data point"=w1268, "sample length"=0, "initialize"=w1264) -> ("max value"=w1286:dbl, "min value"=w1285:dbl)  [unwired: 3 out]
        n790 = case shown="\"Res\"" w1289 {
          tunnel: ["%d" "%.;%_6fHz" "%.;%_3f°C" "%.;%d Ohm" w1612] -> w1296
          tunnel: ["" "f: " "T: " "R: " "Min:  "] -> w1294
          tunnel: [0.0 ("min value") w1565 w1585 w1605 w1616] -> w1291
          tunnel: w1285 -> [_ _ _ _ w1616]
          tunnel: w1284 -> [w1547 w1568 w1588 w1608 w1613]
          tunnel: [w1547 w1568 w1588 w1608 w1613] -> w1283
          tunnel: w1244 -> [w1546 w1563 w1583 w1603 w1611]
          tunnel: w1270 -> [_ w1557 w1577 w1597 _]
          tunnel: [w1546 w1555 w1575 w1595 w1611] -> w1257
          frame "Off", Default {
            (unwired) FALSE
          }
          frame "Freq" {
            (unwired) FALSE
            n791 = call "PM100D_Write.vi"("Command"="SENS:AVER 1", "VISA in"=w1563) -> ("error out"=w1554:errorcluster, "VISA out"=w1562:refnum<visa-resource-name>)  [unwired: 1 in]
            n792 = call "PM100D_Meas.vi"("error in"=w1554, "Timeout"=500 ("Aver"), "ConfPara"="FREQ", "VISA Out"=w1562) -> ("error out"=w1553:errorcluster, "ReadValue"=w1567:string, "dup VISA session"=w1560:refnum<visa-resource-name>)  [unwired: 1 out]
            n793 = Format Into String(format string="SENS:AVER %d", error in=w1553, w1557) -> (resulting string=w1558:string, error out=w1552:errorcluster)  [unwired: 1 in]
            n794 = call "PM100D_Write.vi"("error in (no error)"=w1552, "Command"=w1558, "VISA in"=w1560) -> ("error out"=w1551:errorcluster, "VISA out"=w1555:refnum<visa-resource-name>)
            n795 = Fract/Exp String To Number(use system decimal point (T)=FALSE, string=w1567) -> (number=w1565:dbl)  [unwired: 2 in, 1 out]
            n796 = call <vilib>:"Clear Errors.vi"("error in (no error)"=w1551) -> ()  [unwired: 6 in, 1 out]
          }
          frame "Temp" {
            n797 = call "PM100D_Write.vi"("Command"="SENS:AVER 1", "VISA in"=w1583) -> ("error out"=w1574:errorcluster, "VISA out"=w1582:refnum<visa-resource-name>)  [unwired: 1 in]
            n798 = call "PM100D_Meas.vi"("error in"=w1574, "Timeout"=10 ("Aver"), "ConfPara"="TEMP", "VISA Out"=w1582) -> ("error out"=w1573:errorcluster, "ReadValue"=w1587:string, "dup VISA session"=w1579:refnum<visa-resource-name>)  [unwired: 1 out]
            n799 = Format Into String(format string="SENS:AVER %d", error in=w1573, w1577) -> (resulting string=w1578:string, error out=w1572:errorcluster)  [unwired: 1 in]
            n800 = call "PM100D_Write.vi"("error in (no error)"=w1572, "Command"=w1578, "VISA in"=w1579) -> ("error out"=w1571:errorcluster, "VISA out"=w1575:refnum<visa-resource-name>)
            n801 = Fract/Exp String To Number(use system decimal point (T)=FALSE, string=w1587) -> (number=w1585:dbl)  [unwired: 2 in, 1 out]
            n802 = call <vilib>:"Clear Errors.vi"("error in (no error)"=w1571) -> ()  [unwired: 6 in, 1 out]
          }
          frame "Res" {
            (unwired) FALSE
            n803 = call "PM100D_Write.vi"("Command"="SENS:AVER 1", "VISA in"=w1603) -> ("error out"=w1594:errorcluster, "VISA out"=w1602:refnum<visa-resource-name>)  [unwired: 1 in]
            n804 = call "PM100D_Meas.vi"("error in"=w1594, "Timeout"=10 ("Aver"), "ConfPara"="RES", "VISA Out"=w1602) -> ("error out"=w1593:errorcluster, "ReadValue"=w1607:string, "dup VISA session"=w1599:refnum<visa-resource-name>)  [unwired: 1 out]
            n805 = Format Into String(format string="SENS:AVER %d", error in=w1593, w1597) -> (resulting string=w1598:string, error out=w1592:errorcluster)  [unwired: 1 in]
            n806 = Fract/Exp String To Number(use system decimal point (T)=FALSE, string=w1607) -> (number=w1605:dbl)  [unwired: 2 in, 1 out]
            n807 = call "PM100D_Write.vi"("error in (no error)"=w1592, "Command"=w1598, "VISA in"=w1599) -> ("error out"=w1591:errorcluster, "VISA out"=w1595:refnum<visa-resource-name>)
            n808 = call <vilib>:"Clear Errors.vi"("error in (no error)"=w1591) -> ()  [unwired: 6 in, 1 out]
          }
          frame "Min" {
            n809 = Concatenate Strings("%.;%_4" ("format string"), w1613) -> (w1612:string)
          }
        }
        n810 = case shown="\"Area\"" w1288 {
          tunnel: ["%d" w1439 w1444 w1476 w1490] -> w1295
          tunnel: ["" "Max:  " "Ratio:  " "D: " ""] -> w1293
          tunnel: [0.0 ("min value") w1440 w1446 w1477 w1492] -> w1290
          tunnel: w1286 -> [_ w1440 w1448 _ _]
          tunnel: w1285 -> [_ _ w1447 _ _]
          tunnel: w1283 -> [_ w1437 _ w1472 _]
          tunnel: w1248 -> [_ _ w1445 w1474 w1494]
          tunnel: w1258 -> [_ _ _ w1479 w1493]
          tunnel: w1257 -> [w1432 w1436 w1442 w1470 w1489]
          tunnel: w1273 -> [_ _ _ _ w1488]
          tunnel: [w1432 w1436 w1442 w1470 w1487] -> w1256
          frame "Off", Default {
            (unwired) FALSE
          }
          frame "Max" {
            n811 = Concatenate Strings("%.;%_4" ("format string"), w1437) -> (w1439:string)
          }
          frame "Ratio" {
            (unwired) FALSE
            n812 = case shown="\"W\", Default" w1445 {
              tunnel: w1448 -> [w1453 w1457 w1461 w1465 w1468]
              tunnel: w1447 -> [w1452 w1456 w1460 w1464 w1469]
              tunnel: [w1451 w1455 w1459 w1463 w1467] -> w1446
              tunnel: [w1450 w1454 w1458 w1462 "%.;%_4fdB" ("format string")] -> w1444
              tunnel: "%.;%_6f:1" ("format string") -> [w1450 w1454 w1458 w1462 _]
              frame "W", Default {
                n813 = Divide(x=w1453, y=w1452) -> (x/y=w1451:dbl)
              }
              frame "V" {
                n814 = Divide(x=w1457, y=w1456) -> (x/y=w1455:dbl)
              }
              frame "J" {
                n815 = Divide(x=w1461, y=w1460) -> (x/y=w1459:dbl)
              }
              frame "A" {
                n816 = Divide(x=w1465, y=w1464) -> (x/y=w1463:dbl)
              }
              frame "dBm" {
                n817 = Subtract(x=w1468, y=w1469) -> (x-y=w1467:dbl)
              }
            }
          }
          frame "Area" {
            (unwired) FALSE
            n818 = local read "AOutcm²"() -> (w1478:dbl)
            n819 = case shown="\"A\"" w1474 {
              tunnel: [w1481 w1482 "pW" ("string") w1484 w1485] -> w1471
              tunnel: w1472 -> [w1481 w1482 _ w1484 w1485]
              frame "W", Default {
              }
              frame "J" {
              }
              frame "dBm" {
              }
              frame "A" {
              }
              frame "V" {
              }
            }
            n820 = Divide(x=w1479, y=w1478) -> (x/y=w1477:dbl)
            n821 = Concatenate Strings("%.;%_4" ("format string"), w1471, "/cm²" ("string")) -> (w1476:string)
          }
          frame "Second" {
            n822 = case shown="\"J\"" w1494 {
              tunnel: w1493 -> [w1499 _ _ _ _]
              tunnel: [w1498 w1504 w1525 w1533 w1541] -> w1492
              tunnel: ["%.;%_6fdBm" ("string") w1503 "%.;%_5pW" ("string") "%.;%_5pW" ("string") "%.;%_5pV" ("string")] -> w1490
              tunnel: w1489 -> [w1496 w1505 w1528 w1536 w1544]
              tunnel: w1488 -> [_ w1502 _ _ _]
              tunnel: [w1496 w1501 w1523 w1531 w1539] -> w1487
              tunnel: [errorcluster {"status"=FALSE, "code"=0, "source"=""} ("error out") w1500 w1522 w1530 w1538] -> w1486
              frame "W", Default {
                n823 = call "lin-log.vi"("W In 2"=w1499) -> ("dBm Out 2"=w1498:dbl)  [unwired: 3 in, 3 out]
              }
              frame "V" {
                n824 = case shown="True" w1502 {
                  tunnel: w1505 -> [w1512 w1520]
                  tunnel: [w1509 w1517] -> w1504
                  tunnel: ["%.;%_5pW" ("string") "%.;%_5pJ" ("string")] -> w1503
                  tunnel: [w1507 w1515] -> w1501
                  tunnel: [w1506 w1514] -> w1500
                  frame False {
                    n825 = call "PM100D_Read.vi"("Command"="MEAS?", "VISA in"=w1512) -> ("error out"=w1506:errorcluster, "ReadValue"=w1510:string, "VISA out"=w1507:refnum<visa-resource-name>)  [unwired: 2 in]
                    n826 = Fract/Exp String To Number(use system decimal point (T)=FALSE, string=w1510) -> (number=w1509:dbl)  [unwired: 2 in, 1 out]
                  }
                  frame True {
                    n827 = call "PM100D_Read.vi"("Command"="MEAS:ENER?", "VISA in"=w1520) -> ("error out"=w1514:errorcluster, "ReadValue"=w1518:string, "VISA out"=w1515:refnum<visa-resource-name>)  [unwired: 2 in]
                    n828 = Fract/Exp String To Number(use system decimal point (T)=FALSE, string=w1518) -> (number=w1517:dbl)  [unwired: 2 in, 1 out]
                  }
                }
              }
              frame "dBm" {
                n829 = call "PM100D_Read.vi"("Command"="MEAS?", "VISA in"=w1528) -> ("error out"=w1522:errorcluster, "ReadValue"=w1526:string, "VISA out"=w1523:refnum<visa-resource-name>)  [unwired: 2 in]
                n830 = Fract/Exp String To Number(use system decimal point (T)=FALSE, string=w1526) -> (number=w1525:dbl)  [unwired: 2 in, 1 out]
              }
              frame "A" {
                n831 = call "PM100D_Read.vi"("Command"="MEAS?", "VISA in"=w1536) -> ("error out"=w1530:errorcluster, "ReadValue"=w1534:string, "VISA out"=w1531:refnum<visa-resource-name>)  [unwired: 2 in]
                n832 = Fract/Exp String To Number(use system decimal point (T)=FALSE, string=w1534) -> (number=w1533:dbl)  [unwired: 2 in, 1 out]
              }
              frame "J" {
                n833 = call "PM100D_Read.vi"("Command"="MEAS:VOLT?", "VISA in"=w1544) -> ("error out"=w1538:errorcluster, "ReadValue"=w1542:string, "VISA out"=w1539:refnum<visa-resource-name>)  [unwired: 2 in]
                n834 = Fract/Exp String To Number(use system decimal point (T)=FALSE, string=w1542) -> (number=w1541:dbl)  [unwired: 2 in, 1 out]
              }
            }
            n835 = call <vilib>:"Clear Errors.vi"("error in (no error)"=w1486) -> ()  [unwired: 6 in, 1 out]
          }
        }
        n836 = Format Into String(format string=w1296, initial string=w1294, w1291) -> (resulting string=w1272:string, error out=w1260:errorcluster)  [unwired: 1 in]
        n837 = Format Into String(format string=w1295, initial string=w1293, w1290) -> (resulting string=w1271:string, error out=w1259:errorcluster)  [unwired: 1 in]
        n838 = call <vilib>:"Clear Errors.vi"("error in (no error)"=w1260) -> ()  [unwired: 6 in, 1 out]
        n839 = case shown="True" TRUE {
          tunnel: [w1425 w1428] -> w1281
          tunnel: w1256 -> [_ w1431]
          tunnel: w1248 -> [_ w1429]
          frame False {
            n840 = local read "SlideMulti"() -> (w1425:dbl)
          }
          frame True {
            n841 = local read "16"() -> (w1426:bool)
            n842 = call "PM100D_GetRngLbl.vi"("PM16"=w1426, "MainUnits"=w1429, "PM100D"=w1431) -> ("Auto"=w1427:bool, "Numeric"=w1428:dbl, "String"=w1430:string)
            n843 = local write "AUTO?"(w1427) -> ()
            n844 = property on="Button1" class="Bool (strict)"("BoolText.Text"=w1430) -> ()  [unwired: 2 in, 2 out]
          }
        }
        n845 = call <vilib>:"Clear Errors.vi"("error in (no error)"=w1259) -> ()  [unwired: 6 in, 1 out]
        n846 = Equal?(x="0", y=w1271) -> (x = y?=w1277:bool)
        n847 = Equal?(x="0", y=w1272) -> (x = y?=w1280:bool)
        n848 = Select(t="", s=w1277, f=w1271) -> (s? t:f=w1267:string)
        n849 = Select(t="", s=w1280, f=w1272) -> (s? t:f=w1266:string)
        n850 = local write "Sub2"(w1267) -> ()
        n851 = local write "Sub1"(w1266) -> ()
        n852 = flat-sequence {
          tunnel: [w1619] -> w1297
          frame #0 {
            w1617 = FALSE ("Button7")
            n853 = local read "LTM"() -> (w1618:bool)
            n854 = case shown="False" w1618 {
              frame False {
              }
              frame True {
                n855 = local read "PM100D"() -> (w1621:refnum<visa-resource-name>)
                n856 = local read "Interval"() -> (w1620:dbl)
                n857 = Wait (ms)(milliseconds to wait=w1620) -> ()  [unwired: 1 out]
                n858 = call "PM100D_Close.vi"("VISA resource name"=w1621) -> ()  [unwired: 3 in]
              }
            }
            n859 = local write "Button7"(w1617) -> ()
            n860 = local write "Res"(w1617) -> ()
            n861 = local read "Frame"() -> (w1619:T1)
          }
        }
        n862 = Multiply(x=w1275, y=w1281) -> (x*y=w1292:dbl)
        n863 = local write "Readout"(w1263) -> ()
        n864 = local write "Data"(w1275) -> ()
        n865 = local write "Slide"(w1292) -> ()
      }
      frame "130" {
        n866 = local read "PM100D"() -> (w1628:refnum<visa-resource-name>)
        n867 = local read "MainUnits"() -> (w1625:enum16{"W", "V", "J", "dBm", "A"})
        n868 = case shown="\"W\", Default" w1625 {
          tunnel: ["POW?" "ENER?" "VOLT?" "POW?" "CURR?"] -> w1622
          frame "W", Default {
          }
          frame "J" {
          }
          frame "V" {
          }
          frame "dBm" {
          }
          frame "A" {
          }
        }
        n869 = Concatenate Strings("MEAS:" ("Command"), w1622) -> (w1623:string)
        n870 = call "PM100D_Read.vi"("Command"=w1623, "VISA in"=w1628) -> ("error out"=w1627:errorcluster, "ReadValue"=w1638:string)  [unwired: 2 in, 1 out]
        n871 = local read "Unt"() -> (w1633:string)
        n872 = Unbundle By Name(w1627) -> ("status"=w1626:bool)
        n873 = call <vilib>:"Clear Errors.vi"("error in (no error)"=w1627) -> ()  [unwired: 6 in, 1 out]
        n874 = Equal?(x=w1633, y="dBm") -> (x = y?=w1631:bool)
        n875 = Fract/Exp String To Number(use system decimal point (T)=FALSE, string=w1638) -> (number=w1634:dbl)  [unwired: 2 in, 1 out]
        n876 = local read "Samples"() -> (w1636:u32)
        n877 = case shown="True" w1626 {
          tunnel: w1628 -> [_ w1653]
          frame False {
          }
          frame True {
            n878 = VISA Clear(VISA resource name=w1653) -> (error out=w1652:errorcluster)  [unwired: 1 in, 1 out]
            n879 = call <vilib>:"Clear Errors.vi"("error in (no error)"=w1652) -> ()  [unwired: 6 in, 1 out]
          }
        }
        n880 = local read "N"() -> (w1641:u32)
        n881 = case shown="True" w1631 {
          tunnel: w1634 -> [w1654 w1656]
          tunnel: [w1654 w1655] -> w1630
          frame False {
          }
          frame True {
            n882 = Multiply(x=w1656, y=1000.0) -> (x*y=w1658:dbl)
            n883 = Logarithm Base 10(1:w1658) -> (0:w1660:dbl)
            n884 = Multiply(x=10.0, y=w1660) -> (x*y=w1655:dbl)
          }
        }
        n885 = Increment(x=w1641) -> (x+1=w1640:u32)
        n886 = local read "FileRefnum"() -> (w1645:refnum<file>)
        n887 = local read "EMM"() -> (w1642:bool)
        n888 = call "GetDateTime.vi"() -> ("date&time"=w1629:string)
        n889 = local write "N"(w1640) -> ()
        n890 = Number To Decimal String(number=w1640) -> (decimal integer string=w1635:string)  [unwired: 1 in]
        n891 = Equal?(x=w1636, y=w1640) -> (x = y?=w1644:bool)
        n892 = local write "Stat1"(w1635) -> ()
        n893 = case shown="True" w1642 {
          tunnel: [w1675 w1680] -> w1643
          tunnel: w1630 -> [w1674 w1679]
          tunnel: w1629 -> [w1673 w1678]
          tunnel: w1633 -> [w1671 w1677]
          frame True {
            n894 = local read "T"() -> (w1672:dbl)
            n895 = local read "H"() -> (w1670:dbl)
            n896 = Format Into String(format string="\\t%.4e\\t%s\\t%.1f\\t°C\\t%.1f\\tRH\\n", initial string=w1673, w1674, w1671, w1672, w1670) -> (resulting string=w1675:string)  [unwired: 1 in, 1 out]
          }
          frame False {
            n897 = Format Into String(format string="\\t%.4e\\t%s\\n", initial string=w1678, w1679, w1677) -> (resulting string=w1680:string)  [unwired: 1 in, 1 out]
          }
        }
        n898 = Write to Text File(file (use dialog)=w1645, text=w1643) -> (refnum out=w1646:refnum<file>)  [unwired: 2 in, 2 out]
        n899 = case shown="False" w1644 {
          tunnel: w1646 -> [_ w1669]
          tunnel: [w1661 StateMachine."300" ("Frame")] -> w1639
          frame False {
            n900 = local read "Button6"() -> (w1663:bool)
            n901 = Select(t=StateMachine."130" ("Beginning State"), s=w1663, f=StateMachine."300") -> (s? t:f=w1661:T1)
          }
          frame True {
            n902 = Refnum to Path(1:w1669) -> (0:w1668:path)
            n903 = local write "LFP"(w1668) -> ()
            n904 = local write "Button6"(FALSE ("Button6")) -> ()
            n905 = local write "N"(u32 0 ("N")) -> ()
          }
        }
      }
      frame "140" {
        w1703 = 0 ("t")
        w1702 = 2
        # "Energiemessung"
        n906 = local read "MainUnits"() -> (w1728:enum16{"W", "V", "J", "dBm", "A"})
        n907 = local read "PM100D"() -> (w1706:refnum<visa-resource-name>)
        n908 = local read "Digits"() -> (w1727:i32)
        n909 = local read "Button7"() -> (w1709:bool)
        n910 = local read "SensType"() -> (w1715:i32)
        n911 = local read "Sub1"() -> (w1735:enum16{"Off", "Min", "Freq", "Temp", "Res"})
        n912 = local read "Sub2"() -> (w1734:enum16{"Off", "Max", "Ratio", "Area", "Second"})
        n913 = local read "N2"() -> (w1683:u32)
        n914 = local read "AVG"() -> (w1708:u32)
        n915 = local read "EMM"() -> (w1684:bool)
        n916 = Increment(x=w1683) -> (x+1=w1682:u32)
        n917 = local write "N2"(w1682) -> ()
        n918 = Equal?(x=w1715, y=3) -> (x = y?=w1713:bool)
        n919 = case shown="True" w1684 {
          frame False {
          }
          frame True {
            n920 = local read "N2"() -> (w1744:u32)
            n921 = Equal?(x=w1744, y=u32 20) -> (x = y?=w1745:bool)
            n922 = case shown="True" w1745 {
              frame False {
              }
              frame True {
                n923 = local read "PM100D"() -> (w1758:refnum<visa-resource-name>)
                n924 = call "PM100D_Read.vi"("Command"="SENS3:TEMP:DATA?" ("write buffer"), "VISA in"=w1758) -> ("error out"=w1748:errorcluster, "ReadValue"=w1754:string, "VISA out"=w1757:refnum<visa-resource-name>)  [unwired: 2 in]
                n925 = Equal?(x="", y=w1754) -> (x = y?=w1755:bool)
                n926 = case shown="False" w1755 {
                  tunnel: w1754 -> [w1769 _]
                  frame False {
                    n927 = Fract/Exp String To Number(use system decimal point (T)=FALSE, string=w1769) -> (number=w1765:dbl)  [unwired: 2 in, 1 out]
                    n928 = local write "T"(w1765) -> ()
                    n929 = Format Into String(format string="%.;%.1f\\B0C", w1765) -> (resulting string=w1767:string)  [unwired: 2 in, 1 out]
                    n930 = local write "Temp"(w1767) -> ()
                  }
                  frame True {
                  }
                }
                n931 = call "PM100D_Read.vi"("error in (no error)"=w1748, "Command"="SENS2:HUM:DATA?" ("write buffer"), "VISA in"=w1757) -> ("error out"=w1753:errorcluster, "ReadValue"=w1750:string)  [unwired: 1 in, 1 out]
                n932 = call <vilib>:"Clear Errors.vi"("error in (no error)"=w1753) -> ()  [unwired: 6 in, 1 out]
                n933 = Equal?(x=w1750, y="") -> (x = y?=w1751:bool)
                n934 = case shown="False" w1751 {
                  tunnel: w1750 -> [w1761 _]
                  frame False {
                    n935 = Fract/Exp String To Number(use system decimal point (T)=FALSE, string=w1761) -> (number=w1760:dbl)  [unwired: 2 in, 1 out]
                    n936 = Format Into String(format string="%.;%.1f%", w1760) -> (resulting string=w1763:string)  [unwired: 2 in, 1 out]
                    n937 = local write "Hum"(w1763) -> ()
                    n938 = local write "H"(w1760) -> ()
                  }
                  frame True {
                  }
                }
                n939 = local write "N2"(u32 0 ("N2")) -> ()
              }
            }
          }
        }
        n940 = call "PM100D_Read.vi"("Command"="FETC?", "VISA in"=w1706) -> ("error out"=w1705:errorcluster, "ReadValue"=w1689:string, "VISA out"=w1686:refnum<visa-resource-name>)  [unwired: 2 in]
        n941 = call <vilib>:"Clear Errors.vi"("error in (no error)"=w1705) -> ()  [unwired: 6 in, 1 out]
        n942 = Equal?(x=w1689, y="9.91E37\n") -> (x = y?=w1694:bool)
        n943 = Equal?(x=w1689, y="-9.9E37\n") -> (x = y?=w1695:bool)
        n944 = Build Array(w1694, w1695) -> (w1693:bool[])
        n945 = Boolean Array To Number(Boolean array=w1693) -> (number=w1692:u32)
        n946 = case shown="0, Default" w1692 {
          tunnel: [w1777 w1819 w1828] -> w1730
          tunnel: w1728 -> [w1776 w1818 w1827]
          tunnel: w1727 -> [w1775 _ _]
          tunnel: [w1774 w1816 w1825] -> w1725
          tunnel: [w1773 w1816 w1825] -> w1716
          tunnel: [w1772 "High     " "Low     "] -> w1710
          tunnel: w1689 -> [w1771 _ _]
          frame 0, Default {
            n947 = Number To Decimal String(number=w1775) -> (decimal integer string=w1778:string)  [unwired: 1 in]
            n948 = case shown="\"V\"" w1776 {
              tunnel: [w1784 w1791 w1798 w1806 w1813] -> w1779
              tunnel: [w1781 w1788 w1795 w1805 w1810] -> w1774
              tunnel: w1778 -> [w1785 w1792 w1799 w1807 w1814]
              tunnel: [w1783 w1790 w1797 w1804 w1812] -> w1777
              tunnel: [w1781 w1788 w1795 w1802 w1810] -> w1773
              tunnel: w1771 -> [w1780 w1787 w1794 w1801 w1809]
              frame "W", Default {
                w1783 = "pW" ("string")
                n949 = Fract/Exp String To Number(use system decimal point (T)=FALSE, string=w1780) -> (number=w1781:dbl)  [unwired: 2 in, 1 out]
                n950 = Concatenate Strings("%.;%_" ("string"), w1785, w1783) -> (w1784:string)
              }
              frame "V" {
                w1790 = "pV" ("string")
                n951 = Fract/Exp String To Number(use system decimal point (T)=FALSE, string=w1787) -> (number=w1788:dbl)  [unwired: 2 in, 1 out]
                n952 = Concatenate Strings("%.;%_" ("string"), w1792, w1790) -> (w1791:string)
              }
              frame "J" {
                w1797 = "pJ" ("string")
                n953 = Fract/Exp String To Number(use system decimal point (T)=FALSE, string=w1794) -> (number=w1795:dbl)  [unwired: 2 in, 1 out]
                n954 = Concatenate Strings("%.;%_" ("string"), w1799, w1797) -> (w1798:string)
              }
              frame "dBm" {
                w1804 = "fdBm" ("string")
                n955 = Fract/Exp String To Number(use system decimal point (T)=FALSE, string=w1801) -> (number=w1802:dbl)  [unwired: 2 in, 1 out]
                n956 = call "lin-log.vi"("W In 2"=w1802) -> ("dBm Out 2"=w1805:dbl)  [unwired: 3 in, 3 out]
                n957 = Concatenate Strings("%.;%_" ("string"), w1807, w1804) -> (w1806:string)
              }
              frame "A" {
                w1812 = "pA" ("string")
                n958 = Fract/Exp String To Number(use system decimal point (T)=FALSE, string=w1809) -> (number=w1810:dbl)  [unwired: 2 in, 1 out]
                n959 = Concatenate Strings("%.;%_" ("string"), w1814, w1812) -> (w1813:string)
              }
            }
            n960 = Format Into String(format string=w1779, w1774) -> (resulting string=w1772:string, error out=w1770:errorcluster)  [unwired: 2 in]
            n961 = call <vilib>:"Clear Errors.vi"("error in (no error)"=w1770) -> ()  [unwired: 6 in, 1 out]
          }
          frame 1 {
            w1816 = 0.0
            n962 = case shown="\"dBm\"" w1818 {
              tunnel: ["W" ("string") "V" ("string") "J" ("string") "A" ("string") "dBm" ("string")] -> w1819
              frame "W", Default {
              }
              frame "V" {
              }
              frame "J" {
              }
              frame "A" {
              }
              frame "dBm" {
              }
            }
          }
          frame 2 {
            w1825 = 0.0
            n963 = case shown="\"dBm\"" w1827 {
              tunnel: ["W" ("string") "V" ("string") "J" ("string") "A" ("string") "dBm" ("string")] -> w1828
              frame "W", Default {
              }
              frame "V" {
              }
              frame "J" {
              }
              frame "A" {
              }
              frame "dBm" {
              }
            }
          }
        }
        n964 = call <vilib>:"Array Max & Min PtByPt.vi"("input data point"=w1725, "sample length"=0, "initialize"=w1709) -> ("max value"=w1732:dbl, "min value"=w1731:dbl)  [unwired: 3 out]
        n965 = case shown="\"Off\", Default" w1735 {
          tunnel: ["%d" "%.;%_6fHz" "%.;%_3f°C" w1989] -> w1742
          tunnel: ["" "f: " "T: " "Min:  "] -> w1740
          tunnel: [0.0 ("min value") w1961 w1981 w1993] -> w1737
          tunnel: w1731 -> [_ _ _ w1993]
          tunnel: w1730 -> [w1943 w1964 w1984 w1990]
          tunnel: [w1943 w1964 w1984 w1990] -> w1729
          tunnel: w1686 -> [w1941 w1959 w1979 w1987]
          tunnel: w1708 -> [_ w1953 w1973 _]
          tunnel: [errorcluster {"status"=FALSE, "code"=0, "source"=""} ("error out") w1947 w1971 errorcluster {"status"=FALSE, "code"=0, "source"=""} ("error out")] -> w1704
          tunnel: [w1941 w1950 w1969 w1987] -> w1685
          frame "Off", Default {
          }
          frame "Freq" {
            n966 = call "PM100D_Write.vi"("Command"="SENS:AVER 1", "VISA in"=w1959) -> ("error out"=w1951:errorcluster, "VISA out"=w1958:refnum<visa-resource-name>)  [unwired: 1 in]
            n967 = call "PM100D_Meas.vi"("error in"=w1951, "Timeout"=500 ("Aver"), "ConfPara"="FREQ", "VISA Out"=w1958) -> ("error out"=w1949:errorcluster, "ReadValue"=w1963:string, "dup VISA session"=w1956:refnum<visa-resource-name>)  [unwired: 1 out]
            n968 = Format Into String(format string="SENS:AVER %d", error in=w1949, w1953) -> (resulting string=w1954:string, error out=w1948:errorcluster)  [unwired: 1 in]
            n969 = call "PM100D_Write.vi"("error in (no error)"=w1948, "Command"=w1954, "VISA in"=w1956) -> ("error out"=w1947:errorcluster, "VISA out"=w1950:refnum<visa-resource-name>)
            n970 = Fract/Exp String To Number(use system decimal point (T)=FALSE, string=w1963) -> (number=w1961:dbl)  [unwired: 2 in, 1 out]
          }
          frame "Temp" {
            n971 = call "PM100D_Write.vi"("Command"="SENS:AVER 1", "VISA in"=w1979) -> ("error out"=w1970:errorcluster, "VISA out"=w1978:refnum<visa-resource-name>)  [unwired: 1 in]
            n972 = call "PM100D_Meas.vi"("error in"=w1970, "Timeout"=10 ("Aver"), "ConfPara"="TEMP", "VISA Out"=w1978) -> ("error out"=w1968:errorcluster, "ReadValue"=w1983:string, "dup VISA session"=w1975:refnum<visa-resource-name>)  [unwired: 1 out]
            n973 = Format Into String(format string="SENS:AVER %d", error in=w1968, w1973) -> (resulting string=w1974:string, error out=w1967:errorcluster)  [unwired: 1 in]
            n974 = call "PM100D_Write.vi"("error in (no error)"=w1967, "Command"=w1974, "VISA in"=w1975) -> ("error out"=w1971:errorcluster, "VISA out"=w1969:refnum<visa-resource-name>)
            n975 = Fract/Exp String To Number(use system decimal point (T)=FALSE, string=w1983) -> (number=w1981:dbl)  [unwired: 2 in, 1 out]
          }
          frame "Min" {
            n976 = Concatenate Strings("%.;%_4" ("format string"), w1990) -> (w1989:string)
          }
        }
        n977 = case shown="\"Second\"" w1734 {
          tunnel: ["%d" w1844 w1848 w1879 w1892] -> w1741
          tunnel: ["" "Max:  " "Ratio:  " "D: " ""] -> w1739
          tunnel: [0.0 ("min value") w1845 w1850 w1880 w1894] -> w1736
          tunnel: w1732 -> [_ w1845 w1852 _ _]
          tunnel: w1731 -> [_ _ w1851 _ _]
          tunnel: w1729 -> [_ w1842 _ w1875 _]
          tunnel: w1728 -> [_ _ w1849 w1877 w1896]
          tunnel: w1716 -> [_ _ _ w1882 w1895]
          tunnel: w1685 -> [_ _ _ _ w1891]
          tunnel: w1713 -> [_ _ _ _ w1890]
          frame "Off", Default {
            (unwired) FALSE
          }
          frame "Max" {
            n978 = Concatenate Strings("%.;%_4" ("format string"), w1842) -> (w1844:string)
          }
          frame "Ratio" {
            (unwired) FALSE
            n979 = case shown="\"W\", Default" w1849 {
              tunnel: w1852 -> [w1857 w1861 w1865 w1869 w1872]
              tunnel: w1851 -> [w1856 w1860 w1864 w1868 w1873]
              tunnel: [w1855 w1859 w1863 w1867 w1871] -> w1850
              tunnel: [w1854 w1858 w1862 w1866 "%.;%_4fdB" ("format string")] -> w1848
              tunnel: "%.;%_6f:1" ("format string") -> [w1854 w1858 w1862 w1866 _]
              frame "W", Default {
                n980 = Divide(x=w1857, y=w1856) -> (x/y=w1855:dbl)
              }
              frame "V" {
                n981 = Divide(x=w1861, y=w1860) -> (x/y=w1859:dbl)
              }
              frame "J" {
                n982 = Divide(x=w1865, y=w1864) -> (x/y=w1863:dbl)
              }
              frame "A" {
                n983 = Divide(x=w1869, y=w1868) -> (x/y=w1867:dbl)
              }
              frame "dBm" {
                n984 = Subtract(x=w1872, y=w1873) -> (x-y=w1871:dbl)
              }
            }
          }
          frame "Area" {
            (unwired) FALSE
            n985 = local read "AOutcm²"() -> (w1881:dbl)
            n986 = case shown="\"A\"" w1877 {
              tunnel: [w1884 w1885 "pW" ("string") w1887 w1888] -> w1874
              tunnel: w1875 -> [w1884 w1885 _ w1887 w1888]
              frame "W", Default {
              }
              frame "J" {
              }
              frame "dBm" {
              }
              frame "A" {
              }
              frame "V" {
              }
            }
            n987 = Divide(x=w1882, y=w1881) -> (x/y=w1880:dbl)
            n988 = Concatenate Strings("%.;%_4" ("format string"), w1874, "/cm²" ("string")) -> (w1879:string)
          }
          frame "Second" {
            n989 = case shown="\"V\"" w1896 {
              tunnel: w1895 -> [w1900 _ _ _ _]
              tunnel: [w1899 w1904 w1922 w1929 w1936] -> w1894
              tunnel: ["%.;%_6fdBm" ("string") w1903 "%.;%_5pW" ("string") "%.;%_5pW" ("string") "%.;%_5pV" ("string")] -> w1892
              tunnel: w1891 -> [_ w1905 w1925 w1932 w1939]
              tunnel: w1890 -> [_ w1902 _ _ _]
              tunnel: [errorcluster {"status"=FALSE, "code"=0, "source"=""} ("error out") w1901 w1920 w1927 w1934] -> w1889
              frame "W", Default {
                n990 = call "lin-log.vi"("W In 2"=w1900) -> ("dBm Out 2"=w1899:dbl)  [unwired: 3 in, 3 out]
              }
              frame "V" {
                n991 = case shown="False" w1902 {
                  tunnel: w1905 -> [w1911 w1918]
                  tunnel: [w1908 w1915] -> w1904
                  tunnel: ["%.;%_5pW" ("string") "%.;%_5pJ" ("string")] -> w1903
                  tunnel: [w1906 w1913] -> w1901
                  frame False {
                    n992 = call "PM100D_Read.vi"("Command"="MEAS?", "VISA in"=w1911) -> ("error out"=w1906:errorcluster, "ReadValue"=w1909:string)  [unwired: 2 in, 1 out]
                    n993 = Fract/Exp String To Number(use system decimal point (T)=FALSE, string=w1909) -> (number=w1908:dbl)  [unwired: 2 in, 1 out]
                  }
                  frame True {
                    n994 = call "PM100D_Read.vi"("Command"="MEAS:ENER?", "VISA in"=w1918) -> ("error out"=w1913:errorcluster, "ReadValue"=w1916:string)  [unwired: 2 in, 1 out]
                    n995 = Fract/Exp String To Number(use system decimal point (T)=FALSE, string=w1916) -> (number=w1915:dbl)  [unwired: 2 in, 1 out]
                  }
                }
              }
              frame "dBm" {
                n996 = call "PM100D_Read.vi"("Command"="MEAS?", "VISA in"=w1925) -> ("error out"=w1920:errorcluster, "ReadValue"=w1923:string)  [unwired: 2 in, 1 out]
                n997 = Fract/Exp String To Number(use system decimal point (T)=FALSE, string=w1923) -> (number=w1922:dbl)  [unwired: 2 in, 1 out]
              }
              frame "A" {
                n998 = call "PM100D_Read.vi"("Command"="MEAS?", "VISA in"=w1932) -> ("error out"=w1927:errorcluster, "ReadValue"=w1930:string)  [unwired: 2 in, 1 out]
                n999 = Fract/Exp String To Number(use system decimal point (T)=FALSE, string=w1930) -> (number=w1929:dbl)  [unwired: 2 in, 1 out]
              }
              frame "J" {
                n1000 = call "PM100D_Read.vi"("Command"="MEAS:VOLT?", "VISA in"=w1939) -> ("error out"=w1934:errorcluster, "ReadValue"=w1937:string)  [unwired: 2 in, 1 out]
                n1001 = Fract/Exp String To Number(use system decimal point (T)=FALSE, string=w1937) -> (number=w1936:dbl)  [unwired: 2 in, 1 out]
              }
            }
            n1002 = call <vilib>:"Clear Errors.vi"("error in (no error)"=w1889) -> ()  [unwired: 6 in, 1 out]
          }
        }
        n1003 = Format Into String(format string=w1742, initial string=w1740, w1737) -> (resulting string=w1712:string, error out=w1688:errorcluster)  [unwired: 1 in]
        n1004 = call <vilib>:"Clear Errors.vi"("error in (no error)"=w1704) -> ()  [unwired: 6 in, 1 out]
        n1005 = Format Into String(format string=w1741, initial string=w1739, w1736) -> (resulting string=w1711:string, error out=w1687:errorcluster)  [unwired: 1 in]
        n1006 = local read "SlideMulti"() -> (w1726:dbl)
        n1007 = call <vilib>:"Clear Errors.vi"("error in (no error)"=w1688) -> ()  [unwired: 6 in, 1 out]
        n1008 = call <vilib>:"Clear Errors.vi"("error in (no error)"=w1687) -> ()  [unwired: 6 in, 1 out]
        n1009 = Equal?(x="0", y=w1712) -> (x = y?=w1724:bool)
        n1010 = Equal?(x="0", y=w1711) -> (x = y?=w1720:bool)
        n1011 = Select(t="", s=w1724, f=w1712) -> (s? t:f=w1723:string)
        n1012 = Select(t="", s=w1720, f=w1711) -> (s? t:f=w1718:string)
        n1013 = local write "Sub1"(w1723) -> ()
        n1014 = local write "Sub2"(w1718) -> ()
        n1015 = Multiply(x=w1716, y=w1726) -> (x*y=w1738:dbl)
        n1016 = local write "Readout"(w1710) -> ()
        n1017 = local read "XScaleFit"() -> (w1701:bool)
        n1018 = local read "YScaleFit"() -> (w1700:bool)
        n1019 = local read "YScaleRep"() -> (w1699:bool)
        n1020 = flat-sequence {
          tunnel: [StateMachine."150" ("Frame")] -> w1743
          frame #0 {
            n1021 = local read "LTM"() -> (w1834:bool)
            n1022 = case shown="True" w1834 {
              frame False {
              }
              frame True {
                n1023 = local read "PM100D"() -> (w1837:refnum<visa-resource-name>)
                n1024 = local read "Interval"() -> (w1838:dbl)
                n1025 = call "PM100D_Close.vi"("VISA resource name"=w1837) -> ()  [unwired: 3 in]
                n1026 = Wait (ms)(milliseconds to wait=w1838) -> ()  [unwired: 1 out]
              }
            }
            n1027 = local write "Button7"(FALSE ("Button7")) -> ()
          }
        }
        n1028 = local write "Slide"(w1738) -> ()
        n1029 = local write "Data"(w1716) -> ()
        n1030 = Boolean To (0,1)(Boolean=w1699) -> (0, 1=w1696:i16)
        n1031 = Select(t=w1703, s=w1701, f=w1702) -> (s? t:f=w1698:i32)
        n1032 = Select(t=w1703, s=w1700, f=w1702) -> (s? t:f=w1697:i32)
        n1033 = property on="Chart_E" class="WFChart (strict)"("XScale.ScaleFit"=w1698, "YScale.ScaleFit"=w1697, "YScale.Mapping Mode"=w1696) -> ()  [unwired: 2 in, 2 out]
      }
      frame "150" {
        n1034 = local read "Samples"() -> (w1995:u32)
        n1035 = local read "Button1"() -> (w1999:bool)
        n1036 = local read "Button2"() -> (w2000:bool)
        n1037 = local read "Button3"() -> (w2001:bool)
        n1038 = local read "Button4"() -> (w2002:bool)
        n1039 = local read "Button5"() -> (w2003:bool)
        n1040 = local read "Button6"() -> (w1998:bool)
        n1041 = local read "N"() -> (w1996:u32)
        n1042 = Increment(x=w1996) -> (x+1=w1997:u32)
        n1043 = Greater?(x=w1995, y=w1996) -> (0:w2006:bool)
        n1044 = local write "N"(w1997) -> ()
        n1045 = Compound Arithmetic op=AND(invert w1999, invert w2000, invert w2001, invert w2002, invert w2003, w1998, w2006) -> (w2005:bool)
        n1046 = case shown="True" w2005 {
          tunnel: w1995 -> [w2011 w2024]
          tunnel: w1997 -> [w2012 w2023]
          tunnel: [0 w2027] -> w2004
          tunnel: w1998 -> [w2010 _]
          tunnel: [FALSE TRUE] -> w1994
          frame False {
            n1047 = Equal?(x=w2010, y=TRUE) -> (x = y?=w2015:bool)
            n1048 = Less?(x=w2012, y=w2011) -> (x < y?=w2014:bool)
            n1049 = And(x=w2015, y=w2014) -> (x .and. y?=w2013:bool)
            n1050 = case shown="True" w2013 {
              frame False {
                n1051 = local write "Button6"(FALSE ("Button6")) -> ()
                n1052 = local write "N"(i16 0 ("N")) -> ()
              }
              frame True {
                n1053 = local read "N"() -> (w2019:u32)
                n1054 = Decrement(x=w2019) -> (x-1=w2020:u32)
                n1055 = local write "N"(w2020) -> ()
              }
            }
          }
          frame True {
            n1056 = local read "MainUnits"() -> (w2057:enum16{"W", "V", "J", "dBm", "A"})
            n1057 = case shown="\"dBm\"" w2057 {
              tunnel: ["W" "V" "J" "W" "A"] -> w2036
              tunnel: [w2087 w2091 w2094 w2099 w2103] -> w2041
              tunnel: [FALSE w2091 TRUE FALSE w2103] -> w2040
              tunnel: [w2087 FALSE w2094 w2099 TRUE] -> w2039
              tunnel: ["Power / W" "Energy / V" "Energy / J" "Power / W" ""] -> w2035
              frame "W", Default {
                w2087 = TRUE
              }
              frame "V" {
                w2091 = TRUE
              }
              frame "J" {
                w2094 = FALSE
              }
              frame "dBm" {
                w2099 = TRUE
              }
              frame "A" {
                w2103 = FALSE
              }
            }
            n1058 = Equal?(x=i16 1, y=w2023) -> (x = y?=w2058:bool)
            n1059 = local read "EMM"() -> (w2022:bool)
            n1060 = call "GetDateTime.vi"() -> ("date&time"=w2021:string)
            n1061 = local read "Data"() -> (w2038:dbl)
            n1062 = local read "Int."() -> (w2037:i32)
            n1063 = property on="Chart_E" class="WFChart (strict)"("Visible"=w2040) -> ()  [unwired: 2 in, 2 out]
            n1064 = property on="Chart_P" class="WFChart (strict)"("Visible"=w2039) -> ()  [unwired: 2 in, 2 out]
            n1065 = case shown="True" w2022 {
              tunnel: w2038 -> [w2069 w2077]
              tunnel: w2036 -> [w2068 w2076]
              tunnel: [w2067 w2075] -> w2033
              tunnel: w2021 -> [w2066 w2074]
              tunnel: [w2065 w2073] -> w2028
              frame False {
                n1066 = Format Into String(format string="\\t%.4e\\t%s\\n", initial string=w2066, w2069, w2068) -> (resulting string=w2065:string, error out=w2067:errorcluster)  [unwired: 1 in]
              }
              frame True {
                n1067 = local read "H"() -> (w2071:dbl)
                n1068 = local read "T"() -> (w2072:dbl)
                n1069 = Format Into String(format string="\\t%.4e\\t%s\\t%.1f\\t°C\\t%.1f\\tRH\\n", initial string=w2074, w2077, w2076, w2072, w2071) -> (resulting string=w2073:string, error out=w2075:errorcluster)  [unwired: 1 in]
              }
            }
            n1070 = call <vilib>:"Histogram PtByPt.vi"("initialize"=w2058, "sample length"=w2024, "intervals"=w2037, "x"=w2038) -> ("Histogram Graph"=w2063:T2)  [unwired: 4 in, 3 out]
            n1071 = call <vilib>:"Array Max & Min PtByPt.vi"("input data point"=w2038, "sample length"=w2024, "initialize"=w2058) -> ("max value"=w2049:dbl, "min value"=w2050:dbl)  [unwired: 3 out]
            n1072 = call <vilib>:"Standard Deviation PtByPt.vi"("x"=w2038, "sample length"=w2024, "initialize"=w2058) -> ("standard deviation"=w2056:dbl, "mean"=w2048:dbl)  [unwired: 1 out]
            n1073 = call <vilib>:"RMS PtByPt.vi"("initialize"=w2058, "sample length"=w2024, "x"=w2038) -> ("rms value"=w2047:dbl)  [unwired: 1 in, 1 out]
            n1074 = Format Into String(format string="%d\\n%.3p%s\\n%.3p%s\\n%.3p%s\\n%.3p%s\\n%.3p%s", error in=w2033, w2023, w2050, w2036, w2049, w2036, w2048, w2036, w2047, w2036, w2056, w2036) -> (resulting string=w2060:string, error out=w2032:errorcluster)  [unwired: 1 in]
            n1075 = local read "LogData"() -> (w2062:string)
            n1076 = local write "Unit"(w2035) -> ()
            n1077 = local write "Chart_E"(w2038) -> ()
            n1078 = call "lin-log.vi"("W In 1"=w2047, "W In 2"=w2048, "W In 3"=w2049, "W In 4"=w2050) -> ("dBm Out 1"=w2051:dbl, "dBm Out 2"=w2052:dbl, "dBm Out 3"=w2053:dbl, "dBm Out 4"=w2054:dbl)
            n1079 = local write "Histogram"(w2063) -> ()
            n1080 = Format Into String(format string="%.3fdBm\\n%.3fdBm\\n%.3fdBm\\n%.3fdBm", initial string="\n", error in=w2032, w2054, w2053, w2052, w2051) -> (resulting string=w2045:string, error out=w2031:errorcluster)
            n1081 = Concatenate Strings(w2028, w2062) -> (w2064:string)
            n1082 = local read "FileRefnum"() -> (w2029:refnum<file>)
            n1083 = local write "Chart_P"(w2038) -> ()
            n1084 = local write "Stat1"(w2060) -> ()
            n1085 = local write "Stat0"("Count:\nMin:\nMax:\nMean:\nRMS:\nSigma:" ("Stat0")) -> ()
            n1086 = local write "LogData"(w2064) -> ()
            n1087 = call <vilib>:"Clear Errors.vi"("error in (no error)"=w2031) -> ()  [unwired: 6 in, 1 out]
            n1088 = Select(t=w2045, s=w2041, f="") -> (s? t:f=w2044:string)
            n1089 = Write to Text File(file (use dialog)=w2029, text=w2028) -> (refnum out=w2026:refnum<file>)  [unwired: 2 in, 2 out]
            n1090 = local write "Stat2"(w2044) -> ()
            n1091 = Equal?(x=w2024, y=w2023) -> (x = y?=w2025:bool)
            n1092 = case shown="True" w2025 {
              tunnel: [2 0] -> w2027
              tunnel: [StateMachine."100" ("Frame") StateMachine."300" ("Frame")] -> w2030
              tunnel: w2026 -> [_ w2082]
              frame False {
              }
              frame True {
                n1093 = Refnum to Path(1:w2082) -> (0:w2081:path)
                n1094 = local write "LFP"(w2081) -> ()
              }
            }
            n1095 = local write "Frame"(w2030) -> ()
          }
        }
        n1096 = flat-sequence {
          tunnel: [w2106] -> w2007
          frame #0 {
            n1097 = local read "Frame"() -> (w2106:T1)
            n1098 = local write "Button7"(FALSE ("Button7")) -> ()
          }
        }
        n1099 = local write "Log"(w1994) -> ()
        n1100 = property on="Button1" class="Bool (strict)"("Disabled"=w2004) -> ()  [unwired: 2 in, 2 out]
        n1101 = property on="Button2" class="Bool (strict)"("Disabled"=w2004) -> ()  [unwired: 2 in, 2 out]
        n1102 = property on="Button3" class="Bool (strict)"("Disabled"=w2004) -> ()  [unwired: 2 in, 2 out]
        n1103 = property on="Button4" class="Bool (strict)"("Disabled"=w2004) -> ()  [unwired: 2 in, 2 out]
        n1104 = property on="Button5" class="Bool (strict)"("Disabled"=w2004) -> ()  [unwired: 2 in, 2 out]
      }
      frame "200" {
        # "Set Measurement Range\n1. Get lowest Amp or Voltage Range\n2. Calculate Current or Voltage Ranges\n3. Get Range Index\n4. Set New Range Index\n5. Get Range in the desired Unit"
        n1105 = flat-sequence {
          frame #0 {
            n1106 = local read "MainUnits"() -> (w2117:enum16{"W", "V", "J", "dBm", "A"})
            n1107 = local read "PM100D"() -> (w2118:refnum<visa-resource-name>)
            n1108 = local read "AUTO?"() -> (w2109:bool)
            n1109 = local read "16"() -> (w2108:bool)
            n1110 = case shown="\"W\", Default" w2117 {
              tunnel: ["POW" "VOLT" "ENER" "POW" "CURR"] -> w2116
              tunnel: ["W" "V" "J" "W" "A"] -> w2115
              frame "W", Default {
              }
              frame "V" {
              }
              frame "J" {
              }
              frame "dBm" {
              }
              frame "A" {
              }
            }
            n1111 = call "SetRange.vi"("PM16"=w2108, "Unit"=w2116, "AUTO"=w2109, "VISA in"=w2118) -> ("AUTO?"=w2113:bool, "RANG_Val"=w2111:dbl, "RANG_lbl"=w2119:string)  [unwired: 4 in, 1 out]
            n1112 = Divide(x=1000.0, y=w2111) -> (x/y=w2110:dbl)
            n1113 = Concatenate Strings("Range " ("string"), w2119, w2115) -> (w2120:string)
            n1114 = property on="Button1" class="Bool (strict)"("BoolText.Text"=w2120) -> ()  [unwired: 2 in, 2 out]
            n1115 = local write "SlideMulti"(w2110) -> ()
            n1116 = local write "AUTO?"(w2113) -> ()
          }
          frame #1 {
            n1117 = local write "Button1"(FALSE ("Button6")) -> ()
            n1118 = local write "Frame"(StateMachine."100" ("Frame")) -> ()
          }
        }
      }
      frame "220" {
        n1119 = flat-sequence {
          frame #0 {
            n1120 = local read "Lambda"() -> (w2143:dbl)
            n1121 = local read "LambdaMin"() -> (w2135:dbl)
            n1122 = local read "LambdaMax"() -> (w2136:dbl)
            n1123 = local read "SensType"() -> (w2142:i32)
            n1124 = local read "Sensor?"() -> (w2137:bool)
            n1125 = call "SetWavelength.vi"("LambdaIn"=w2143, "LambdaMax"=w2136, "LambdaMin"=w2135, "Sensor?"=w2137, "RespIn"=w2143, "Type"=w2142) -> ("LambdaOut"=w2145:dbl, "RespOut"=w2144:dbl)
            n1126 = case shown="True" w2137 {
              tunnel: w2145 -> [w2148 _]
              tunnel: [w2148 w2157] -> w2138
              tunnel: [w2147 w2156] -> w2139
              tunnel: [w2146 w2155] -> w2140
              tunnel: w2142 -> [_ w2158]
              tunnel: w2144 -> [_ w2157]
              frame True {
                n1127 = Format Into String(format string="%dnm", initial string="Wave ", w2148) -> (resulting string=w2147:string)  [unwired: 1 in, 1 out]
                n1128 = Format Into String(format string="%d", initial string="SENS:CORR:WAV " ("Command"), w2148) -> (resulting string=w2146:string)  [unwired: 1 in, 1 out]
              }
              frame False {
                n1129 = case shown="0, Default" w2158 {
                  tunnel: [w2163 "" ("initial string") "" ("initial string") "" ("initial string")] -> w2162
                  tunnel: [w2163 "%.;%_3pA/W" ("format string") "%.;%_3pV/W" ("format string") "%.;%_3pV/J" ("format string")] -> w2161
                  tunnel: [w2163 "SENS:CORR:POW " ("Command") "SENS:CORR:POW:THER " ("Command") "SENS:CORR:ENER " ("Command")] -> w2160
                  tunnel: [w2163 "%.;%.6e" ("format string") "%.;%.6e" ("format string") "%.;%.6e" ("format string")] -> w2159
                  frame 0, Default {
                    w2163 = "" ("format string")
                  }
                  frame 1 {
                  }
                  frame 2 {
                  }
                  frame 3 {
                  }
                }
                n1130 = Format Into String(format string=w2161, initial string=w2162, w2157) -> (resulting string=w2156:string, error out=w2154:errorcluster)  [unwired: 1 in]
                n1131 = Format Into String(format string=w2159, initial string=w2160, error in=w2154, w2157) -> (resulting string=w2155:string, error out=w2153:errorcluster)
                n1132 = call <vilib>:"Clear Errors.vi"("error in (no error)"=w2153) -> ()  [unwired: 6 in, 1 out]
              }
            }
            n1133 = local read "PM100D"() -> (w2141:refnum<visa-resource-name>)
            n1134 = property on="Button2" class="Bool (strict)"("BoolText.Text"=w2139) -> ()  [unwired: 2 in, 2 out]
            n1135 = local write "Lambda"(w2138) -> ()
            n1136 = call "PM100D_Write.vi"("Command"=w2140, "VISA in"=w2141) -> ("error out"=w2134:errorcluster)  [unwired: 1 in, 1 out]
            n1137 = call <vilib>:"Clear Errors.vi"("error in (no error)"=w2134) -> ()  [unwired: 6 in, 1 out]
          }
          frame #1 {
            n1138 = local write "Button2"(FALSE ("Button6")) -> ()
            n1139 = local write "Frame"(StateMachine."100" ("Frame")) -> ()
          }
        }
      }
      frame "240" {
        n1140 = flat-sequence {
          tunnel: [w2224] -> w2179
          tunnel: w2179 -> [w2318]
          tunnel: [w2315] -> w2178
          frame #0 {
            n1141 = local read "PM100D"() -> (w2228:refnum<visa-resource-name>)
            n1142 = local read "Adapter"() -> (w2222:i16)
            n1143 = local read "ACC"() -> (w2220:string)
            n1144 = local read "Digits"() -> (w2239:i32)
            n1145 = local read "SensType"() -> (w2229:i32)
            n1146 = local read "Tau"() -> (w2225:dbl)
            n1147 = local read "AVG"() -> (w2240:u32)
            n1148 = local read "Trig"() -> (w2243:dbl)
            n1149 = local read "Dia"() -> (w2241:dbl)
            n1150 = local read "BW"() -> (w2246:u16)
            n1151 = local read "Tau?"() -> (w2217:bool)
            n1152 = local read "Sensor?"() -> (w2223:bool)
            n1153 = local read "Att"() -> (w2209:dbl)
            n1154 = local read "16"() -> (w2183:bool)
            n1155 = case shown="\":AUTO ON\", Default" w2220 {
              tunnel: ["ON" "ON" "OFF" "OFF" "AUTO" "AUTO"] -> w2219
              frame "ON" {
              }
              frame " ON" {
              }
              frame "OFF" {
              }
              frame " OFF" {
              }
              frame ":AUTO ON", Default {
              }
              frame "AUTO" {
              }
            }
            n1156 = call "MeasCfg.vi"("DigitsIn"=w2239, "TauIn"=w2225, "PM16"=w2183, "AvgIn"=w2240, "TrigIn"=w2243, "DiaIn"=w2241, "AttIn"=w2209, "Type"=w2229, "VISA In"=w2228, "Sensor?"=w2223, "Adapter"=w2222, "BWIn"=w2246, "Tau?"=w2217, "ACCIn"=w2219) -> ("Ini"=w2224:bool, "DiaSet"=w2245:dbl, "ACCOut"=w2227:string, "BWOut"=w2215:u16, "AttOut"=w2198:dbl, "DigitsOut"=w2238:i32, "AvgOut"=w2197:i32, "TauIOut"=w2221:dbl, "TrigOut"=w2226:dbl, "DiaOut"=w2244:dbl, "AOutcm²"=w2242:dbl)  [unwired: 3 in]
            n1157 = local write "AOutcm²"(w2242) -> ()
            n1158 = local write "Digits"(w2238) -> ()
            n1159 = local write "ACC"(w2227) -> ()
            n1160 = local write "Tau"(w2221) -> ()
            n1161 = local write "Trig"(w2226) -> ()
            n1162 = local write "BW"(w2215) -> ()
            n1163 = local write "Dia"(w2245) -> ()
            n1164 = case shown="2" w2229 {
              tunnel: w2228 -> [_ w2287 w2301 w2314]
              tunnel: w2227 -> [_ _ w2299 _]
              tunnel: w2226 -> [_ _ _ w2311]
              tunnel: w2221 -> [_ _ w2296 _]
              tunnel: [errorcluster {"status"=FALSE, "code"=0, "source"=""} ("error out") w2286 w2295 w2310] -> w2216
              tunnel: w2217 -> [_ _ w2293 _]
              tunnel: w2215 -> [_ w2285 _ _]
              tunnel: w2197 -> [w2282 w2284 w2291 _]
              tunnel: [w2282 w2284 w2291 1 ("AvgOut")] -> w2180
              frame 0, Default {
              }
              frame 1 {
                n1165 = Format Into String(format string="%d", initial string="INP:FILT ", w2285) -> (resulting string=w2290:string)  [unwired: 1 in, 1 out]
                n1166 = call "PM100D_Write.vi"("Command"=w2290, "VISA in"=w2287) -> ("error out"=w2286:errorcluster)  [unwired: 1 in, 1 out]
              }
              frame 2 {
                n1167 = Format Into String(format string="INP:THER:ACC%s", w2299) -> (resulting string=w2300:string)  [unwired: 2 in, 1 out]
                n1168 = Wait (ms)(milliseconds to wait=u32 30) -> ()  [unwired: 1 out]
                n1169 = call "PM100D_Write.vi"("Command"=w2300, "VISA in"=w2301) -> ("error out"=w2294:errorcluster, "VISA out"=w2297:refnum<visa-resource-name>)  [unwired: 1 in]
                n1170 = case shown="True" w2293 {
                  tunnel: w2297 -> [_ w2308]
                  tunnel: w2296 -> [_ w2307]
                  tunnel: [w2302 w2304] -> w2295
                  tunnel: w2294 -> [w2302 w2303]
                  frame False {
                  }
                  frame True {
                    n1171 = Format Into String(format string="INP:THER:ACC:TAU %.;%f", w2307) -> (resulting string=w2305:string)  [unwired: 2 in, 1 out]
                    n1172 = call "PM100D_Write.vi"("error in (no error)"=w2303, "Command"=w2305, "VISA in"=w2308) -> ("error out"=w2304:errorcluster)  [unwired: 1 out]
                  }
                }
              }
              frame 3 {
                n1173 = Format Into String(format string="SENS:PEAK %.;%f", w2311) -> (resulting string=w2313:string)  [unwired: 2 in, 1 out]
                n1174 = call "PM100D_Write.vi"("Command"=w2313, "VISA in"=w2314) -> ("error out"=w2310:errorcluster)  [unwired: 1 in, 1 out]
              }
            }
            n1175 = Wait (ms)(milliseconds to wait=u32 30) -> ()  [unwired: 1 out]
            n1176 = local write "Att"(w2198) -> ()
            n1177 = local read "16"() -> (w2181:bool)
            n1178 = call <vilib>:"Clear Errors.vi"("error in (no error)"=w2216) -> ()  [unwired: 6 in, 1 out]
            n1179 = case shown="True" w2181 {
              tunnel: w2228 -> [w2253 w2255]
              tunnel: [w2249 w2255] -> w2218
              tunnel: w2180 -> [w2247 w2254]
              frame False {
                n1180 = Format Into String(format string="%d", initial string="SENS:AVER " ("Command"), w2247) -> (resulting string=w2251:string)  [unwired: 1 in, 1 out]
                n1181 = call "PM100D_Write.vi"("Command"=w2251, "VISA in"=w2253) -> ("error out"=w2248:errorcluster, "VISA out"=w2249:refnum<visa-resource-name>)  [unwired: 1 in]
                n1182 = call <vilib>:"Clear Errors.vi"("error in (no error)"=w2248) -> ()  [unwired: 6 in, 1 out]
              }
              frame True {
                n1183 = local write "NPL"(w2254) -> ()
              }
            }
            n1184 = Number To Fractional String(use system decimal point (T)=FALSE, number=w2244) -> (F-format string=w2212:string)  [unwired: 2 in]
            n1185 = Number To Fractional String(use system decimal point (T)=FALSE, number=w2198) -> (F-format string=w2200:string)  [unwired: 2 in]
            n1186 = local read "Samples"() -> (w2234:u32)
            n1187 = local read "Interval"() -> (w2232:dbl)
            n1188 = local read "File?"() -> (w2231:bool)
            n1189 = Concatenate Strings("SENS:CORR:BEAM " ("initial string"), w2212) -> (w2213:string)
            n1190 = local read "MainUnits"() -> (w2195:enum16{"W", "V", "J", "dBm", "A"})
            n1191 = Concatenate Strings("SENS:CORR " ("string"), w2200) -> (w2207:string)
            n1192 = Format Into String(format string="%.;%.2f %s", initial string="a = ", w2198, " dB") -> (resulting string=w2199:string)  [unwired: 1 in, 1 out]
            n1193 = local write "att"(w2199) -> ()
            n1194 = call "PM100D_Write.vi"("Command"=w2213, "VISA in"=w2218) -> ("error out"=w2182:errorcluster, "VISA out"=w2206:refnum<visa-resource-name>)  [unwired: 1 in]
            n1195 = call "PM100D_Write.vi"("Command"=w2207, "VISA in"=w2206) -> ("error out"=w2205:errorcluster, "VISA out"=w2196:refnum<visa-resource-name>)  [unwired: 1 in]
            n1196 = Divide(x=w2232, y=1000.0) -> (x/y=w2236:dbl)
            n1197 = case shown="\"W\", Default" w2195 {
              tunnel: ["POW" "VOLT" "ENER" "POW" "CURR"] -> w2191
              tunnel: ["W" "V" "J" "W" "A"] -> w2194
              tunnel: w2196 -> [w2257 w2261 w2265 w2269 w2273]
              tunnel: [w2257 w2261 w2265 w2269 w2273] -> w2190
              tunnel: [TRUE FALSE TRUE TRUE FALSE] -> w2192
              frame "W", Default {
              }
              frame "V" {
              }
              frame "J" {
              }
              frame "dBm" {
              }
              frame "A" {
              }
            }
            n1198 = call <vilib>:"Clear Errors.vi"("error in (no error)"=w2182) -> ()  [unwired: 6 in, 1 out]
            n1199 = call <vilib>:"Clear Errors.vi"("error in (no error)"=w2205) -> ()  [unwired: 6 in, 1 out]
            n1200 = Format Into String(format string="Samples:    %d\\nInterval:      %.2fs\\nAveraging: %d\\nLog to File: %s", initial string="Logging Parameters\n", w2234, w2236, w2180, w2231) -> (resulting string=w2235:string)  [unwired: 1 in, 1 out]
            n1201 = local write "AVG"(w2180) -> ()
            n1202 = property on="att" class="Str"("Visible"=w2192) -> ()  [unwired: 2 in, 2 out]
            n1203 = local write "LogCfg"(w2235) -> ()
            n1204 = call "PM100D-GetSetRng.vi"("Unit"=w2191, "VISA Refnum in"=w2190) -> ("error out"=w2189:errorcluster, "Range"=w2185:dbl, "lblRange"=w2187:string)  [unwired: 7 in]
            n1205 = Divide(x=1000.0, y=w2185) -> (x/y=w2184:dbl)
            n1206 = Concatenate Strings("Range " ("string"), w2187, w2194) -> (w2193:string)
            n1207 = property on="Button1" class="Bool (strict)"("BoolText.Text"=w2193) -> ()  [unwired: 2 in, 2 out]
            n1208 = local write "SlideMulti"(w2184) -> ()
            n1209 = call <vilib>:"Clear Errors.vi"("error in (no error)"=w2189) -> ()  [unwired: 6 in, 1 out]
          }
          frame #1 {
            w2316 = StateMachine."100" ("f")
            n1210 = local write "Button3"(FALSE ("Button6")) -> ()
            n1211 = Select(t=StateMachine."Load Settings" ("Frame"), s=w2318, f=w2316) -> (s? t:f=w2315:T1)
            n1212 = local write "Frame"(w2316) -> ()
          }
        }
      }
      frame "260" {
        n1213 = flat-sequence {
          tunnel: [w2322] -> w2320
          tunnel: w2320 -> [w2332]
          frame #0 {
            n1214 = local read "MainUnits"() -> (w2325:enum16{"W", "V", "J", "dBm", "A"})
            n1215 = local read "SensType"() -> (w2329:i32)
            n1216 = local read "Temp"() -> (w2323:bool)
            n1217 = local read "Sub1"() -> (w2326:enum16{"Off", "Min", "Freq", "Temp", "Res"})
            n1218 = local read "Sub2"() -> (w2327:enum16{"Off", "Max", "Ratio", "Area", "Second"})
            n1219 = call "SetUnits.vi"("Temp"=w2323, "SensType"=w2329, "Sub1In"=w2326, "Sub2In"=w2327, "MainUnitsIn"=w2325) -> ("Sub1Out"=w2324:enum16{"Off", "Min", "Freq", "Temp", "Res"}, "Sub2Out"=w2328:u16, "MainUnitsOut"=w2322:enum16{"W", "V", "J", "dBm", "A"})
            n1220 = local write "MainUnits"(w2322) -> ()
            n1221 = local write "Sub1"(w2324) -> ()
            n1222 = local write "Sub2"(w2328) -> ()
          }
          frame #1 {
            n1223 = local read "PM100D"() -> (w2340:refnum<visa-resource-name>)
            n1224 = case shown="\"dBm\"" w2332 {
              tunnel: ["POW" "VOLT" "ENER" "POW" "CURR"] -> w2336
              tunnel: ["W" "V" "J" "W" "A"] -> w2337
              tunnel: w2340 -> [w2343 w2347 w2351 w2355 w2359]
              tunnel: [w2343 w2347 w2351 w2355 w2359] -> w2341
              tunnel: [TRUE FALSE TRUE TRUE FALSE] -> w2331
              frame "W", Default {
              }
              frame "V" {
              }
              frame "J" {
              }
              frame "dBm" {
              }
              frame "A" {
              }
            }
            n1225 = call "PM100D-GetSetRng.vi"("Unit"=w2336, "VISA Refnum in"=w2341) -> ("Range"=w2330:dbl, "lblRange"=w2338:string)  [unwired: 7 in, 1 out]
            n1226 = property on="att" class="Str"("Visible"=w2331) -> ()  [unwired: 2 in, 2 out]
            n1227 = Divide(x=1000.0, y=w2330) -> (x/y=w2333:dbl)
            n1228 = Concatenate Strings("Range " ("string"), w2338, w2337) -> (w2335:string)
            n1229 = local write "SlideMulti"(w2333) -> ()
            n1230 = property on="Button1" class="Bool (strict)"("BoolText.Text"=w2335) -> ()  [unwired: 2 in, 2 out]
          }
          frame #2 {
            n1231 = local write "Button4"(FALSE ("Button6")) -> ()
            n1232 = local write "Frame"(StateMachine."100" ("Frame")) -> ()
          }
        }
      }
      frame "280" {
        n1233 = flat-sequence {
          frame #0 {
            w2368 = "ON" ("regular expression")
            w2394 = 1000 ("y")
            n1234 = local read "Samples"() -> (w2395:u32)
            n1235 = local read "Header"() -> (w2382:string)
            n1236 = local read "SensType"() -> (w2389:i32)
            n1237 = local read "AVG"() -> (w2397:u32)
            n1238 = local read "File?"() -> (w2396:bool)
            n1239 = local read "ACC"() -> (w2370:string)
            n1240 = local read "Interval"() -> (w2391:dbl)
            n1241 = local read "FastIn"() -> (w2378:bool)
            n1242 = Divide(x=w2391, y=w2394) -> (x/y=w2392:dbl)
            n1243 = Match Pattern(string=w2370, regular expression=w2368) -> (match substring=w2369:string)  [unwired: 1 in, 3 out]
            n1244 = local read "16"() -> (w2365:bool)
            n1245 = Equal?(x=w2369, y=w2368) -> (x = y?=w2367:bool)
            n1246 = local read "Data_Dir"() -> (w2366:path)
            n1247 = call "LogCfg.vi"("SamplesIn"=w2395, "FastIn"=w2378, "PM16"=w2365, "IntervalIn"=w2392, "ACCON"=w2367, "AveragingIn"=w2397, "FileIn"=w2396, "SensType"=w2389, "LogPath"=w2366) -> ("FileRefnum"=w2383:refnum<file>, "SamplesOut"=w2399:i32, "IntervalOut"=w2393:dbl, "AveragingOut"=w2390:i32, "FastOut"=w2375:bool, "FileOut"=w2385:bool)  [unwired: 1 in]
            n1248 = Refnum to Path(1:w2383) -> (0:w2388:path)
            n1249 = Concatenate Strings(w2382, "\r\n") -> (w2381:string)
            n1250 = local write "FastOut"(w2375) -> ()
            n1251 = local write "FastIn"(w2375) -> ()
            n1252 = Strip Path(path=w2388) -> (name=w2387:string)  [unwired: 1 out]
            n1253 = Write to Text File(file (use dialog)=w2383, text=w2381) -> (refnum out=w2376:refnum<file>, cancelled=w2377:bool, error out=w2379:errorcluster)  [unwired: 2 in]
            n1254 = Multiply(x=w2393, y=w2394) -> (x*y=w2402:dbl)
            n1255 = case shown="False" w2377 {
              tunnel: w2379 -> [_ w2412]
              tunnel: w2376 -> [w2411 _]
              frame False {
                n1256 = local write "FileRefnum"(w2411) -> ()
                n1257 = Refnum to Path(1:w2411) -> (0:w2410:path)
                n1258 = local write "LFP"(w2410) -> ()
              }
              frame True {
                n1259 = call <vilib>:"Clear Errors.vi"("error in (no error)"=w2412) -> ()  [unwired: 6 in, 1 out]
              }
            }
            n1260 = local write "Samples"(w2399) -> ()
            n1261 = local write "Interval"(w2402) -> ()
            n1262 = case shown="True" w2365 {
              tunnel: w2390 -> [w2404 w2409]
              frame False {
                n1263 = local read "PM100D"() -> (w2405:refnum<visa-resource-name>)
                n1264 = Format Into String(format string="%d", initial string="SENS:AVER " ("Command"), w2404) -> (resulting string=w2407:string)  [unwired: 1 in, 1 out]
                n1265 = call "PM100D_Write.vi"("Command"=w2407, "VISA in"=w2405) -> ("error out"=w2403:errorcluster)  [unwired: 1 in, 1 out]
                n1266 = call <vilib>:"Clear Errors.vi"("error in (no error)"=w2403) -> ()  [unwired: 6 in, 1 out]
              }
              frame True {
                n1267 = local write "NPL"(w2409) -> ()
              }
            }
            n1268 = local write "File?"(w2385) -> ()
            n1269 = local write "AVG"(w2390) -> ()
            n1270 = Divide(x=w2402, y=1000.0) -> (x/y=w2371:dbl)
            n1271 = Select(t=0.0, s=w2375, f=w2371) -> (s? t:f=w2372:dbl)
            n1272 = Select(t=w2387, s=w2385, f="") -> (s? t:f=w2386:string)
            n1273 = Format Into String(format string="Samples:    %d\\nInterval:      %.;%.1fs\\nAveraging: %d\\nLog to File: %s\\n%s", initial string="Logging Parameters\n", w2399, w2372, w2390, w2385, w2386) -> (resulting string=w2401:string)  [unwired: 1 in, 1 out]
            n1274 = local write "LogCfg"(w2401) -> ()
          }
          frame #1 {
            n1275 = local write "Button5"(FALSE ("Button6")) -> ()
            n1276 = local write "Frame"(StateMachine."100" ("Frame")) -> ()
          }
        }
      }
      frame "300" {
        n1277 = flat-sequence {
          frame #0 {
            n1278 = local read "LFP"() -> (w2416:path)
            n1279 = Read from Text File(file (use dialog)=w2416, count=-1) -> (text=w2418:string, cancelled=w2419:bool, error out=w2420:errorcluster)  [unwired: 2 in, 1 out]
            n1280 = case shown="False" w2419 {
              tunnel: w2418 -> [w2422 _]
              tunnel: w2420 -> [_ w2500]
              frame False {
                n1281 = flat-sequence {
                  tunnel: w2422 -> [w2425]
                  tunnel: [w2425] -> w2421
                  tunnel: w2421 -> [w2438]
                  frame #0 {
                    n1282 = local write "Histogram"(T4 {"X Values"=[], "Histogram: h(x)"=[]} ("Histogram Graph")) -> ()
                    n1283 = property on="Chart_P" class="WFChart (strict)"("History Data"=dbl[] []) -> ()  [unwired: 2 in, 2 out]
                  }
                  frame #1 {
                    n1284 = local write "LogData"(w2438) -> ()
                    n1285 = Spreadsheet String To Array(format string="%s", spreadsheet string=w2438, array type (2D Dbl)="") -> (array=w2435:string[][])  [unwired: 1 in]
                    n1286 = Array Subset(array=w2435, index (row)=1 ("index"), index (col)=0 ("index"), length (col)=1 ("length")) -> (w2431:string[][])  [unwired: 1 in]
                    n1287 = Index Array(array=w2431, index (col)=0 ("disabled index (col)")) -> (element=w2429:string[])  [unwired: 1 in]
                    n1288 = Array Subset(array=w2435, index (row)=1 ("index"), index (col)=1 ("index"), length (col)=1 ("length")) -> (w2436:string[][])  [unwired: 1 in]
                    n1289 = Array Subset(array=w2435, index (row)=1 ("index"), index (col)=2 ("index"), length (col)=1 ("length")) -> (w2441:string[][])  [unwired: 1 in]
                    n1290 = local read "Int."() -> (w2439:i32)
                    n1291 = Index Array(array=w2436, index (col)=0 ("disabled index (col)")) -> (element=w2449:string[])  [unwired: 1 in]
                    n1292 = Index Array(array=w2441, index (col)=0 ("disabled index (col)")) -> (element=w2440:string[])  [unwired: 1 in]
                    n1293 = Fract/Exp String To Number(string=w2449, default (0 dbl)=0.0 ("default (0 DBL)")) -> (number=w2430:dbl[])  [unwired: 2 in, 1 out]
                    n1294 = Array Size(array=w2430) -> (size(s)=w2447:i32)
                    n1295 = call <vilib>:"Histogram.vi"("intervals"=w2439, "X"=w2430) -> ("Histogram Graph"=w2446:T2)  [unwired: 6 in, 3 out]
                    n1296 = local write "Histogram"(w2446) -> ()
                    n1297 = for {
                      N: w2447 -> [w2463]
                      tunnel: w2430 -> [w2459] mode=indexing
                      tunnel: w2440 -> [w2491] mode=indexing
                      tunnel: w2429 -> [w2464] mode=indexing
                      tunnel: [w2474] -> w2428 mode=indexing
                      tunnel: [w2459] -> w2427 mode=indexing
                      i -> [w2461]
                      w2473 = " " ("delimiter (Tab)")
                      n1298 = local write "Chart_P"(w2459) -> ()
                      n1299 = local write "Chart_E"(w2459) -> ()
                      n1300 = Equal?(x=0, y=w2461) -> (x = y?=w2496:bool)
                      n1301 = call <vilib>:"Array Max & Min PtByPt.vi"("input data point"=w2459, "sample length"=w2463, "initialize"=w2496) -> ("max value"=w2480:dbl, "min value"=w2481:dbl)  [unwired: 3 out]
                      n1302 = call <vilib>:"Standard Deviation PtByPt.vi"("x"=w2459, "sample length"=w2463, "initialize"=w2496) -> ("standard deviation"=w2492:dbl, "mean"=w2479:dbl)  [unwired: 1 out]
                      n1303 = call <vilib>:"RMS PtByPt.vi"("initialize"=w2496, "sample length"=w2463, "x"=w2459) -> ("rms value"=w2478:dbl)  [unwired: 1 in, 1 out]
                      n1304 = local read "SensType"() -> (w2457:i32)
                      n1305 = Increment(x=w2461) -> (x+1=w2460:i32)
                      n1306 = Equal?(x=w2463, y=w2460) -> (x = y?=w2462:bool)
                      n1307 = Equal?(x=w2491, y="W") -> (x = y?=w2485:bool)
                      n1308 = Spreadsheet String To Array(delimiter (Tab)=w2473, format string="%s", spreadsheet string=w2464, array type (2D Dbl)=string[] []) -> (array=w2468:string[])
                      n1309 = Format Into String(format string="%d\\n%.3p%s\\n%.3p%s\\n%.3p%s\\n%.3p%s\\n%.3p%s", w2463, w2481, w2491, w2480, w2491, w2479, w2491, w2478, w2491, w2492, w2491) -> (resulting string=w2493:string)  [unwired: 2 in, 1 out]
                      n1310 = Equal?(x=w2457, y=3) -> (x = y?=w2456:bool)
                      n1311 = Index Array(array=w2468, index #1=1 ("index"), index #2=0 ("index")) -> (element #1=w2472:string, element #2=w2471:string)
                      n1312 = case shown="False" w2456 {
                        tunnel: w2462 -> [w2498 _]
                        frame False {
                          n1313 = Not(x=w2498) -> (.not. x?=w2499:bool)
                          n1314 = property on="Chart_P" class="WFChart (strict)"("Visible"=w2499) -> ()  [unwired: 2 in, 2 out]
                          n1315 = property on="YT" class="XYGraph (strict)"("Visible"=w2498) -> ()  [unwired: 2 in, 2 out]
                        }
                        frame True {
                        }
                      }
                      n1316 = call "lin-log.vi"("W In 1"=w2478, "W In 2"=w2479, "W In 3"=w2480, "W In 4"=w2481) -> ("dBm Out 1"=w2483:dbl, "dBm Out 2"=w2488:dbl, "dBm Out 3"=w2487:dbl, "dBm Out 4"=w2486:dbl)
                      n1317 = local write "Stat0"("Count:\nMin:\nMax:\nMean:\nRMS:\nSigma:" ("Stat0")) -> ()
                      n1318 = Concatenate Strings(w2472, w2473, w2471) -> (w2465:string)
                      n1319 = local write "Stat1"(w2493) -> ()
                      n1320 = Format Into String(format string="%.3fdBm\\n%.3fdBm\\n%.3fdBm\\n%.3fdBm", initial string="\n", w2486, w2487, w2488, w2483) -> (resulting string=w2476:string)  [unwired: 1 in, 1 out]
                      n1321 = Select(t=w2476, s=w2485, f="") -> (s? t:f=w2477:string)
                      n1322 = Scan From String(input string=w2465, default 1=timestamp(0 s since 1904-01-01)) -> (output 1=w2474:timestamp)  [unwired: 3 in, 3 out]
                      n1323 = local write "Stat2"(w2477) -> ()
                    }
                    n1324 = Bundle(w2428, w2427) -> (w2426:cluster{timestamp[], dbl[]})  [unwired: 1 in]
                    n1325 = local write "YT"(w2426) -> ()
                  }
                }
              }
              frame True {
                n1326 = call <vilib>:"Clear Errors.vi"("error in (no error)"=w2500) -> ()  [unwired: 6 in, 1 out]
              }
            }
          }
          frame #1 {
            n1327 = local write "Imp"(FALSE ("Imp")) -> ()
            n1328 = local write "Frame"(StateMachine."100" ("Frame")) -> ()
          }
        }
      }
      frame "Stop" {
        n1329 = flat-sequence {
          frame #0 {
            w2504 = T22 2 items=["Deassert REN", "Assert REN", "Go To Local; Deassert REN ", "Assert REN; Address Device", "Local Lockout (Addressed Devices)", "Local Lockout (This Device)", "Go To Local"] ("Mode")
            n1330 = local read "PM100D"() -> (w2506:refnum<visa-resource-name>)
            n1331 = disable-structure shown="Enabled" {
              frame Enabled {
                n1332 = local write "Frame"(StateMachine."Initialize" ("Frame")) -> ()
              }
              frame Disabled {
              }
            }
            n1333 = local write "Button8"(FALSE ("Button8")) -> ()
            n1334 = call "PM100D_Close.vi"("Mode"=w2504, "VISA resource name"=w2506) -> ()  [unwired: 2 in]
          }
          frame #1 {
            n1335 = Quit LabVIEW(quit? (T)=TRUE) -> ()
          }
        }
      }
    }
    n1336 = local read "Stop"() -> (w595:bool)
  }
  "Stop" <- FALSE ("Stop")
